vi "3.0.0_Power_Tunings & AW_Performance_Test_ECO_&_BOOST.vi"(7 "Data in":T1, 8 "error in (no error)":errorcluster, 9 "AllControls In":T2, 10 "?":T4, 11 "Message Queue out":T5) -> (0 "error out":errorcluster, 1 "Flow":string, 2 "Data":T4, 3 "Message Queue Out":T5, 5 "Data out":T1)   [LabVIEW 2017]
uses:
  Depends/AMC/subVIs/TypeDefs/amc_Message Queue.ctl
  Depends/AMC/subVIs/TypeDefs/amc_Message.ctl
  Depends/Tools/Keyed Array/Tools_KeyedArray KeyedArray.ctl
  Ctrls/Data.ctl
  DIPC 692 Daemon API/typdef/airwatt tune parameter.ctl
  Ctrls/AllControls.ctl
  Ctrls/CSV_Data.ctl
panel:
  in  "absolute position/mm 2":i32=10
  out "Array":T3[](array[typedef])
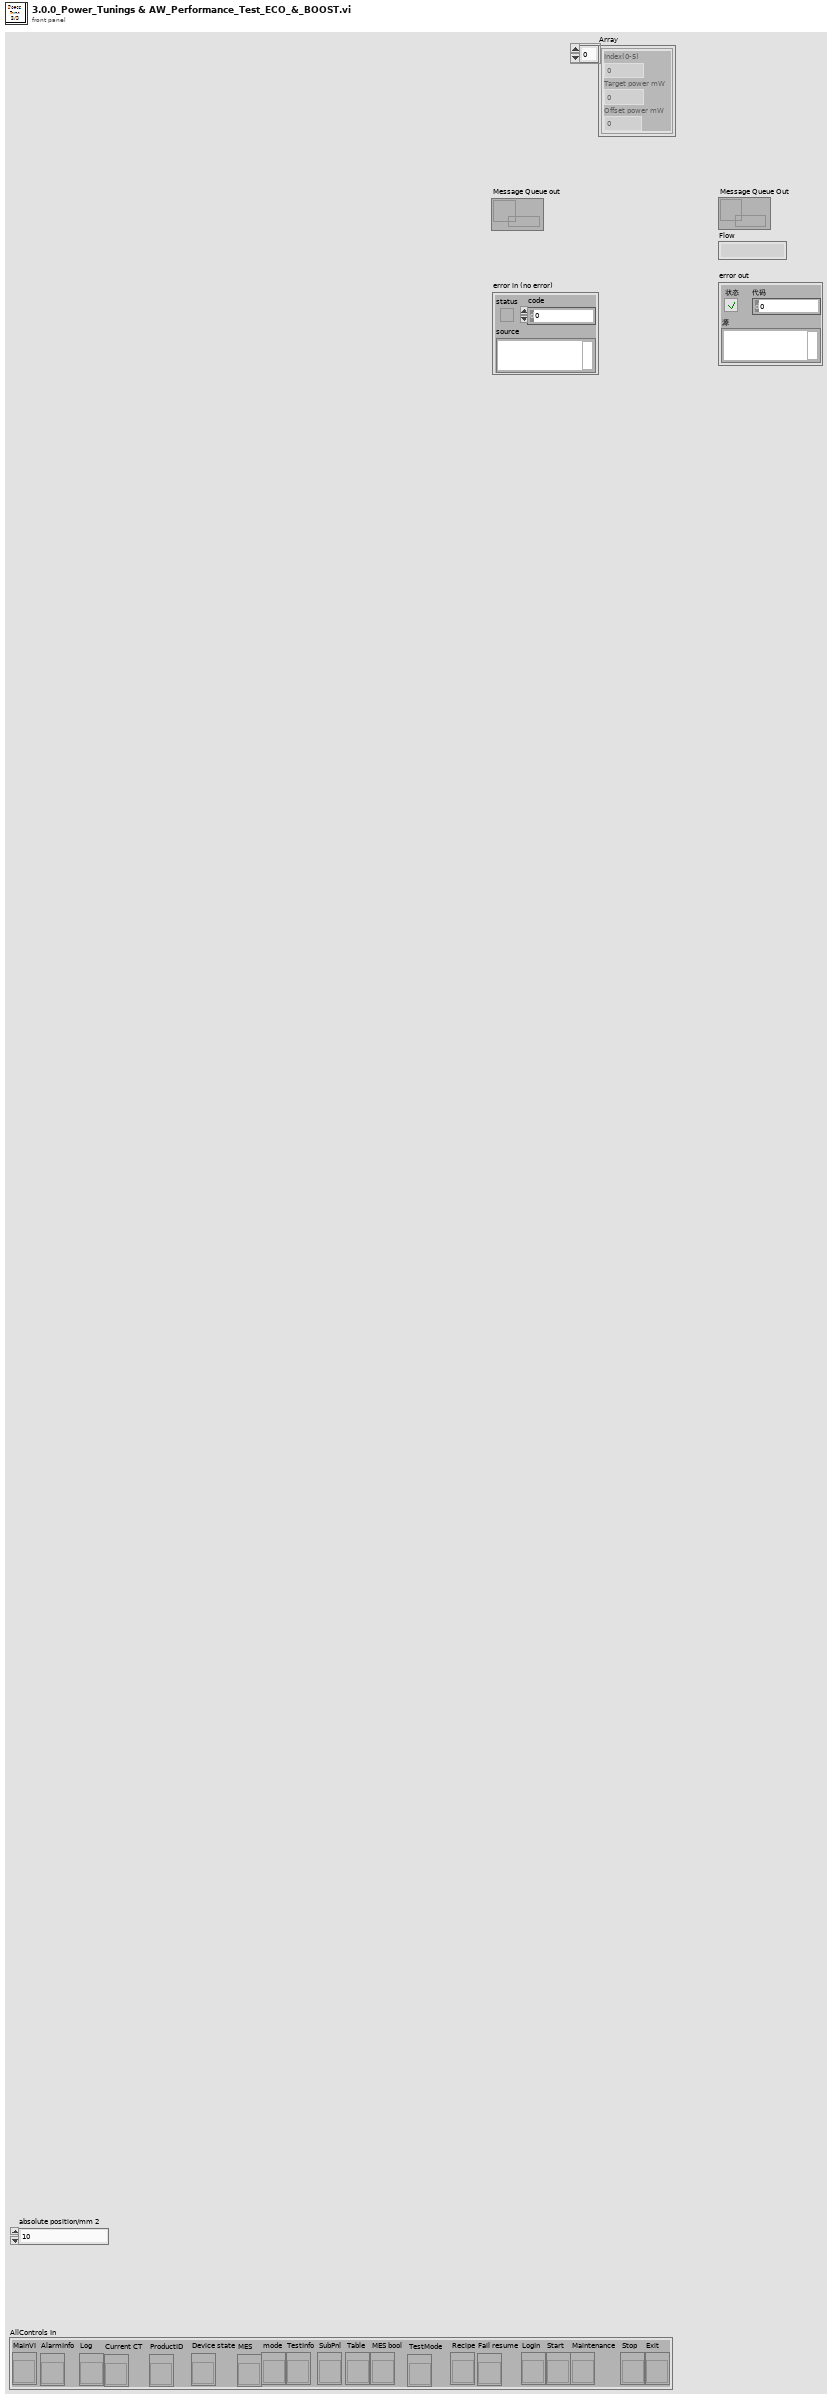
[diagram p1: front panel]
types:
  T1 = typedef "CSV_Data.ctl" = cluster{"Initialisation":cluster{"LMT - Connect UUT (con COM)":string, "LMT - Software Version (rrel)":string, "LMT - Write SKU file (wskuc)":string, "LMT - SKU file name":string, "Connect UUT DDM":string, "Read DDM EOL Timestamp - Mode":string, "Read DDM EOL Timestamp - Timestamp":string, "Read DDM EOL Timestamp - Rig ID":string, "Read DDM EOL Timestamp - Passmark ID":string, "Read DDM EOL Timestamp - Passmark Rev":string, "Software Version before flashing":string, "Read Hardware Serial":string, "UUT DDM SN":string, "Compare DDM SN with MES SN":string, "Backup PCBA Calibration EEPROM Response - CAL":string, "Flash Firmware Version":string, "Check SW Version":string, "Read DDM SW Version after flashing":string, "Set SKU Config":string, "Ready Status":string, "Set Device Mode to EOL":string, "DDM Parameter - Voltage":string, "DDM Parameter - Current":string, "DDM Parameter - Power":string, "DDM Parameter - Speed":string, "DDM Parameter - Pressure":string, "Tester Parameter - Voltage":string, "Tester Parameter - Current":string, "Tester Parameter - Power":string, "Tester Parameter - Ambient Pressure":string, "Tester Parameter - Ambient Temperature":string, "Calculated Parameter - DDM Pressure Corrected":string, "Calculated Parameter - DDM Real Power":string, "Calculated Parameter - Delta V":string}, "BEMF_Calibration":cluster{"Calibration Result - eol_cold_bemf_temp":string, "DDM Ambient Temp":string, "Restriction Plate Diameter":string, "Calibration Result - eol_bemf_mp_cold_coef_a":string, "Calibration Result - eol_bemf_mp_cold_coef_b":string, "Calibration Result - eol_bemf_mp_cold_coef_c":string, "Calibration Result - eol_bemf_lsi_cold_ref_coeffs":string, "Get - Calibration Result - eol_bemf_lsi_speed":string, "Get - Calibration Result - eol_bemf_lsi_integral_0":string, "Calibration Result - eol_bemf_lsi_integral_1":string, "Get - Calibration Result - eol_bemf_lsi_integral_2":string, "Get - Calibration Result - eol_cold_bemf":string, "Get - Calibration Result - eol_cold_bemf_fisf":string, "Finalise Calibration":string, "Compare -Calibration Result - eol_cold_bemf":string, "Compare -Calibration Result - eol_cold_bemf_fisf":string}, "ECO":cluster{"Reset Power Tune":string, "Reset BEMF FISF Calibration":string, "Restriction Plate Diameter":string, "ECO - Stabilisation Time":string, "ECO - DDM Parameter - Voltage":string, "ECO - DDM Parameter - Current":string, "ECO - DDM Parameter - Power":string, "ECO - DDM Parameter - Measured Power":string, "ECO - DDM Parameter - Speed":string, "ECO - DDM Parameter - Pressure":string, "ECO - Tester Parameter - Voltage":string, "ECO - Tester Parameter - Current":string, "ECO - Tester Parameter - Power":string, "ECO - Tester Parameter - Ambient Pressure":string, "ECO - Tester Parameter - Ambient Temperature":string, "ECO - Tester Parameter - Ambient Humidity":string, "ECO - Calculated Parameter - DDM Pressure Corrected":string, "ECO - Calculated Parameter - DDM Real Power":string, "ECO - Calculated Parameter - Delta V":string, "ECO - Calculated Parameter - Flowrate":string, "ECO - Calculated Parameter - Airwatt":string, "ECO - Formula":string, "PT ECO - Power Tune Mode Status":string}, "BOOST":cluster{"Restriction Plate Diameter":string, "BOOST - Stabilisation Time":string, "BOOST - DDM Parameter - Voltage":string, "BOOST - DDM Parameter - Current":string, "BOOST - DDM Parameter - Power":string, "BOOST - DDM Parameter - Measured Power":string, "BOOST - DDM Parameter - Speed":string, "BOOST - DDM Parameter - Pressure":string, "BOOST - Tester Parameter - Voltage":string, "BOOST - Tester Parameter - Current":string, "BOOST - Tester Parameter - Power":string, "BOOST - Tester Parameter - Ambient Pressure":string, "BOOST - Tester Parameter - Ambient Temperature":string, "BOOST - Tester Parameter - Ambient Humidity":string, "BOOST - Calculated Parameter - DDM Pressure Corrected":string, "BOOST - Calculated Parameter - DDM Real Power":string, "BOOST - Calculated Parameter - Delta V":string, "BOOST - Calculated Parameter - Flowrate":string, "BOOST - Calculated Parameter - Airwatt":string, "BOOST - Get AM Presence":string, "Air Muscle Turn Off Status":string, "BOOST - Air Muscle Calculated Parameter - Airwatt B":string, "BOOST - Air Muscle Calculate Airwatt Delta":string, "PT BOOST - Power Tune Mode Status":string, "Finalise Calibration":string, "ECO - Get AW Calibration value":string, "BOOST - Get AW Calibration value":string}, "MAX":cluster{"Restriction Plate Diameter":string, "MAX - Stabilisation Time":string, "Get Average Delta Tmag (LSIdelta_FISFdelta_LSItmag_FISFtmag_IIRtmag)":string, "Get Average Delta Tmag FISF":string, "MAX - DDM Parameter - Voltage":string, "MAX - DDM Parameter - Current":string, "MAX - DDM Parameter - Power":string, "MAX - DDM Parameter - Measured Power":string, "MAX - DDM Parameter - Speed":string, "MAX - DDM Parameter - Pressure":string, "MAX - Tester Parameter - Voltage":string, "MAX - Tester Parameter - Current":string, "MAX - Tester Parameter - Power":string, "MAX - Tester Parameter - Ambient Pressure":string, "MAX - Tester Parameter - Ambient Temperature":string, "MAX - Tester Parameter - Ambient Humidity":string, "MAX - Calculated Parameter - DDM Pressure Corrected":string, "MAX - Calculated Parameter - DDM Real Power":string, "MAX - Calculated Parameter - Delta V":string, "MAX - Calculated Parameter - Flowrate":string, "MAX - Calculated Parameter - Airwatt":string, "MAX_FISF_Check_Average_Delta_Tmag":string, "MAX - FISF - BEMF Finetune Result":string, "MAX tune - Delta P1":string, "MAX tune - Calculated Parameter - Airwatt":string, "Calculate Delta Airwatts - MAX finetune - Delta P2":string, "MAX finetune - DDM Parameter - Voltage":string, "MAX finetune - DDM Parameter - Current":string, "MAX finetune - DDM Parameter - Power":string, "MAX finetune - DDM Parameter - Measured Power":string, "MAX finetune - DDM Parameter - Speed":string, "MAX finetune - DDM Parameter - Pressure":string, "MAX finetune - Tester Parameter - Voltage":string, "MAX finetune - Tester Parameter - Current":string, "MAX finetune - Tester Parameter - Power":string, "MAX finetune - Tester Parameter - Ambient Pressure":string, "MAX finetune - Tester Parameter - Ambient Temperature":string, "MAX finetune - Tester Parameter - Ambient Humidity":string, "MAX finetune - Calculated Parameter - DDM Pressure Corrected":string, "MAX finetune - Calculated Parameter - DDM Real Power":string, "MAX finetune - Calculated Parameter - Delta V":string, "MAX finetune - Calculated Parameter - Flowrate":string, "MAX finetune - Calculated Parameter - Airwatt":string, "Check Derate Result":string, "Delta Tmag FISF":string, "Get Hot BEMF Result":string, "Calculate delta Pressure":string, "Finalise Calibration":string, "Calculate & Check Delta BEMF":string, "Delta P Airwatts Value":string}, "LL":cluster{"DDM Ambient Temp":string, "Restriction Plate Diameter":string, "LL - DDM Parameter - Voltage":string, "LL - DDM Parameter - Current":string, "LL - DDM Parameter - Power":string, "LL - DDM Parameter - Measured Power":string, "LL - DDM Parameter - Speed":string, "LL - DDM Parameter - Pressure":string, "LL - Tester Parameter - Voltage":string, "LL - Tester Parameter - Current":string, "LL - Tester Parameter - Power":string, "LL - DDM Real Power":string, "LL - Calibrate Task Detect LL":string}, "HL":cluster{"HL - DDM Parameter - Voltage":string, "HL - DDM Parameter - Current":string, "HL - DDM Parameter - Power":string, "HL - DDM Parameter - Measured Power":string, "HL - DDM Parameter - Speed":string, "HL - DDM Parameter - Pressure":string, "HL - Tester Parameter - Voltage":string, "HL - Tester Parameter - Current":string, "HL - Tester Parameter - Power":string, "HL - DDM Real Power":string, "HL - Calibrate Task Detect HL":string}, "LH":cluster{"Restriction Plate Diameter":string, "LH - DDM Parameter - Voltage":string, "LH - DDM Parameter - Current":string, "LH - DDM Parameter - Power":string, "LH - DDM Parameter - Measured Power":string, "LH - DDM Parameter - Speed":string, "LH - DDM Parameter - Pressure":string, "LH - Tester Parameter - Voltage":string, "LH - Tester Parameter - Current":string, "LH - Tester Parameter - Power":string, "LH - DDM Real Power":string, "LH - Calibrate Task Detect LH":string}, "HH":cluster{"HH - DDM Parameter - Voltage":string, "HH - DDM Parameter - Current":string, "HH - DDM Parameter - Power":string, "HH - DDM Parameter - Measured Power":string, "HH - DDM Parameter - Speed":string, "HH - DDM Parameter - Pressure":string, "HH - Tester Parameter - Voltage":string, "HH - Tester Parameter - Current":string, "HH - Tester Parameter - Power":string, "HH - DDM Real Power":string, "HH - Calibrate Task Detect HH":string}, "Inlet Blockage Calibration":cluster{"Inlet Blockage Calibration - DDM Parameter - Voltage":string, "Inlet Blockage Calibration - DDM Parameter - Current":string, "Inlet Blockage Calibration - DDM Parameter - Power":string, "Inlet Blockage Calibration - DDM Parameter - Measured Power":string, "Inlet Blockage Calibration - DDM Parameter - Speed":string, "Inlet Blockage Calibration - DDM Parameter - Pressure":string, "Inlet Blockage Calibration - Tester Parameter - Voltage":string, "Inlet Blockage Calibration - Tester Parameter - Current":string, "Inlet Blockage Calibration - Tester Parameter - Power":string, "Inlet Blockage Calibration - DDM Real Power":string, "Calibration Inlet Blockage_E":string, "Finalise Calibration":string, "Get Task Detect LL":string, "Get Task Detect HL":string, "Get Task Detect LH":string, "Get Task Detect HH":string, "Calibration Inlet Blockage":string, "Calibration eol cold bemf temp":string}, "GOOD":cluster{"GOOD UNIT - Clear EEPROM Error Log":string, "GOOD UNIT - Write Product Timestamp - Mode":string, "GOOD UNIT - Write Product Timestamp - Timestamp":string, "GOOD UNIT - Write Product Timestamp - Rig ID":string, "GOOD UNIT - Write Product Timestamp - Passmark ID":string, "GOOD UNIT - Write Product Timestamp - Passmark Rev":string, "GOOD UNIT - Set Device Mode to PROD":string, "GOOD UNIT - Backup PCBA Calibration EEPROM Response":string, "GOOD UNIT - Check Security Bit":string, "GOOD UNIT - Set Calibration Lock":string, "GOOD UNIT - Get_Calibration_Lock":string, "GOOD UNIT - Disconnect UUT":string}, "NG":cluster{"NG UNIT - Read NVM Error":string, "NG UNIT - Set Device Mode to FCT":string, "NG UNIT - Backup PCBA Calibration EEPROM Response - CAL":string, "NG UNIT - Backup PCBA Calibration EEPROM Response - ERROR":string, "NG UNIT - Backup PCBA Calibration EEPROM Response - USAGE":string, "NG UNIT - Disconnect UUT":string}, "SN":string, "Table":string[][], "Count":cluster{"Total":i32, "OK":i32, "NG":i32, "Yield":dbl}, "Start Time":timestamp, "daemon reference":refnum<k5>, "CT":dbl, "Config":string[][], "OK/NG":bool, "Station ID":string, "MES DDM SN":string, "MES PCBA SN":string, "Retest":string, "Lux":string, "Initialisation_Status":cluster{"LMT - Connect UUT (con COM)":string, "LMT - Software Version (rrel)":string, "LMT - Write SKU file (wskuc)":string, "LMT - SKU file name":string, "Connect UUT DDM":string, "Read DDM EOL Timestamp - Mode":string, "Read DDM EOL Timestamp - Timestamp":string, "Read DDM EOL Timestamp - Rig ID":string, "Read DDM EOL Timestamp - Passmark ID":string, "Read DDM EOL Timestamp - Passmark Rev":string, "Software Version before flashing":string, "Read Hardware Serial":string, "UUT DDM SN":string, "Compare DDM SN with MES SN":string, "Backup PCBA Calibration EEPROM Response - CAL":string, "Flash Firmware Version":string, "Check SW Version":string, "Read DDM SW Version after flashing":string, "Set SKU Config":string, "Ready Status":string, "Set Device Mode to EOL":string, "DDM Parameter - Voltage":string, "DDM Parameter - Current":string, "DDM Parameter - Power":string, "DDM Parameter - Speed":string, "DDM Parameter - Pressure":string, "Tester Parameter - Voltage":string, "Tester Parameter - Current":string, "Tester Parameter - Power":string, "Tester Parameter - Ambient Pressure":string, "Tester Parameter - Ambient Temperature":string, "Calculated Parameter - DDM Pressure Corrected":string, "Calculated Parameter - DDM Real Power":string, "Calculated Parameter - Delta V":string}, "BEMF_Calibration_Status":cluster{"Calibration Result - eol_cold_bemf_temp":string, "DDM Ambient Temp":string, "Restriction Plate Diameter":string, "Calibration Result - eol_bemf_mp_cold_coef_a":string, "Calibration Result - eol_bemf_mp_cold_coef_b":string, "Calibration Result - eol_bemf_mp_cold_coef_c":string, "Calibration Result - eol_bemf_lsi_cold_ref_coeffs":string, "Get - Calibration Result - eol_bemf_lsi_speed":string, "Get - Calibration Result - eol_bemf_lsi_integral_0":string, "Calibration Result - eol_bemf_lsi_integral_1":string, "Get - Calibration Result - eol_bemf_lsi_integral_2":string, "Get - Calibration Result - eol_cold_bemf":string, "Get - Calibration Result - eol_cold_bemf_fisf":string, "Finalise Calibration":string, "Compare -Calibration Result - eol_cold_bemf":string, "Compare -Calibration Result - eol_cold_bemf_fisf":string}, "ECO_Status":cluster{"Reset Power Tune":string, "Reset BEMF FISF Calibration":string, "Restriction Plate Diameter":string, "ECO - Stabilisation Time":string, "ECO - DDM Parameter - Voltage":string, "ECO - DDM Parameter - Current":string, "ECO - DDM Parameter - Power":string, "ECO - DDM Parameter - Measured Power":string, "ECO - DDM Parameter - Speed":string, "ECO - DDM Parameter - Pressure":string, "ECO - Tester Parameter - Voltage":string, "ECO - Tester Parameter - Current":string, "ECO - Tester Parameter - Power":string, "ECO - Tester Parameter - Ambient Pressure":string, "ECO - Tester Parameter - Ambient Temperature":string, "ECO - Tester Parameter - Ambient Humidity":string, "ECO - Calculated Parameter - DDM Pressure Corrected":string, "ECO - Calculated Parameter - DDM Real Power":string, "ECO - Calculated Parameter - Delta V":string, "ECO - Calculated Parameter - Flowrate":string, "ECO - Calculated Parameter - Airwatt":string, "ECO - Formula":string, "PT ECO - Power Tune Mode Status":string}, "BOOST_Status":cluster{"Restriction Plate Diameter":string, "BOOST - Stabilisation Time":string, "BOOST - DDM Parameter - Voltage":string, "BOOST - DDM Parameter - Current":string, "BOOST - DDM Parameter - Power":string, "BOOST - DDM Parameter - Measured Power":string, "BOOST - DDM Parameter - Speed":string, "BOOST - DDM Parameter - Pressure":string, "BOOST - Tester Parameter - Voltage":string, "BOOST - Tester Parameter - Current":string, "BOOST - Tester Parameter - Power":string, "BOOST - Tester Parameter - Ambient Pressure":string, "BOOST - Tester Parameter - Ambient Temperature":string, "BOOST - Tester Parameter - Ambient Humidity":string, "BOOST - Calculated Parameter - DDM Pressure Corrected":string, "BOOST - Calculated Parameter - DDM Real Power":string, "BOOST - Calculated Parameter - Delta V":string, "BOOST - Calculated Parameter - Flowrate":string, "BOOST - Calculated Parameter - Airwatt":string, "BOOST - Get AM Presence":string, "Air Muscle Turn Off Status":string, "BOOST - Air Muscle Calculated Parameter - Airwatt B":string, "BOOST - Air Muscle Calculate Airwatt Delta":string, "PT BOOST - Power Tune Mode Status":string, "Finalise Calibration":string, "ECO - Get AW Calibration value":string, "BOOST - Get AW Calibration value":string}, "MAX_Status":cluster{"Restriction Plate Diameter":string, "MAX - Stabilisation Time":string, "Get Average Delta Tmag (LSIdelta_FISFdelta_LSItmag_FISFtmag_IIRtmag)":string, "Get Average Delta Tmag FISF":string, "MAX - DDM Parameter - Voltage":string, "MAX - DDM Parameter - Current":string, "MAX - DDM Parameter - Power":string, "MAX - DDM Parameter - Measured Power":string, "MAX - DDM Parameter - Speed":string, "MAX - DDM Parameter - Pressure":string, "MAX - Tester Parameter - Voltage":string, "MAX - Tester Parameter - Current":string, "MAX - Tester Parameter - Power":string, "MAX - Tester Parameter - Ambient Pressure":string, "MAX - Tester Parameter - Ambient Temperature":string, "MAX - Tester Parameter - Ambient Humidity":string, "MAX - Calculated Parameter - DDM Pressure Corrected":string, "MAX - Calculated Parameter - DDM Real Power":string, "MAX - Calculated Parameter - Delta V":string, "MAX - Calculated Parameter - Flowrate":string, "MAX - Calculated Parameter - Airwatt":string, "MAX_FISF_Check_Average_Delta_Tmag":string, "MAX - FISF - BEMF Finetune Result":string, "MAX tune - Delta P1":string, "MAX tune - Calculated Parameter - Airwatt":string, "Calculate Delta Airwatts - MAX finetune - Delta P2":string, "MAX finetune - DDM Parameter - Voltage":string, "MAX finetune - DDM Parameter - Current":string, "MAX finetune - DDM Parameter - Power":string, "MAX finetune - DDM Parameter - Measured Power":string, "MAX finetune - DDM Parameter - Speed":string, "MAX finetune - DDM Parameter - Pressure":string, "MAX finetune - Tester Parameter - Voltage":string, "MAX finetune - Tester Parameter - Current":string, "MAX finetune - Tester Parameter - Power":string, "MAX finetune - Tester Parameter - Ambient Pressure":string, "MAX finetune - Tester Parameter - Ambient Temperature":string, "MAX finetune - Tester Parameter - Ambient Humidity":string, "MAX finetune - Calculated Parameter - DDM Pressure Corrected":string, "MAX finetune - Calculated Parameter - DDM Real Power":string, "MAX finetune - Calculated Parameter - Delta V":string, "MAX finetune - Calculated Parameter - Flowrate":string, "MAX finetune - Calculated Parameter - Airwatt":string, "Check Derate Result":string, "Delta Tmag FISF":string, "Get Hot BEMF Result":string, "Calculate delta Pressure":string, "Finalise Calibration":string, "Calculate & Check Delta BEMF":string, "Delta P Airwatts Value":string}, "LL_Status":cluster{"DDM Ambient Temp":string, "Restriction Plate Diameter":string, "LL - DDM Parameter - Voltage":string, "LL - DDM Parameter - Current":string, "LL - DDM Parameter - Power":string, "LL - DDM Parameter - Measured Power":string, "LL - DDM Parameter - Speed":string, "LL - DDM Parameter - Pressure":string, "LL - Tester Parameter - Voltage":string, "LL - Tester Parameter - Current":string, "LL - Tester Parameter - Power":string, "LL - DDM Real Power":string, "LL - Calibrate Task Detect LL":string}, "HL_Status":cluster{"HL - DDM Parameter - Voltage":string, "HL - DDM Parameter - Current":string, "HL - DDM Parameter - Power":string, "HL - DDM Parameter - Measured Power":string, "HL - DDM Parameter - Speed":string, "HL - DDM Parameter - Pressure":string, "HL - Tester Parameter - Voltage":string, "HL - Tester Parameter - Current":string, "HL - Tester Parameter - Power":string, "HL - DDM Real Power":string, "HL - Calibrate Task Detect HL":string}, "LH_Status":cluster{"Restriction Plate Diameter":string, "LH - DDM Parameter - Voltage":string, "LH - DDM Parameter - Current":string, "LH - DDM Parameter - Power":string, "LH - DDM Parameter - Measured Power":string, "LH - DDM Parameter - Speed":string, "LH - DDM Parameter - Pressure":string, "LH - Tester Parameter - Voltage":string, "LH - Tester Parameter - Current":string, "LH - Tester Parameter - Power":string, "LH - DDM Real Power":string, "LH - Calibrate Task Detect LH":string}, "HH_Status":cluster{"HH - DDM Parameter - Voltage":string, "HH - DDM Parameter - Current":string, "HH - DDM Parameter - Power":string, "HH - DDM Parameter - Measured Power":string, "HH - DDM Parameter - Speed":string, "HH - DDM Parameter - Pressure":string, "HH - Tester Parameter - Voltage":string, "HH - Tester Parameter - Current":string, "HH - Tester Parameter - Power":string, "HH - DDM Real Power":string, "HH - Calibrate Task Detect HH":string}, "Inlet Blockage Calibration_Status":cluster{"Inlet Blockage Calibration - DDM Parameter - Voltage":string, "Inlet Blockage Calibration - DDM Parameter - Current":string, "Inlet Blockage Calibration - DDM Parameter - Power":string, "Inlet Blockage Calibration - DDM Parameter - Measured Power":string, "Inlet Blockage Calibration - DDM Parameter - Speed":string, "Inlet Blockage Calibration - DDM Parameter - Pressure":string, "Inlet Blockage Calibration - Tester Parameter - Voltage":string, "Inlet Blockage Calibration - Tester Parameter - Current":string, "Inlet Blockage Calibration - Tester Parameter - Power":string, "Inlet Blockage Calibration - DDM Real Power":string, "Calibration Inlet Blockage_E":string, "Finalise Calibration":string, "Get Task Detect LL":string, "Get Task Detect HL":string, "Get Task Detect LH":string, "Get Task Detect HH":string, "Calibration Inlet Blockage":string, "Calibration eol cold bemf temp":string}, "GOOD_Status":cluster{"GOOD UNIT - Clear EEPROM Error Log":string, "GOOD UNIT - Write Product Timestamp - Mode":string, "GOOD UNIT - Write Product Timestamp - Timestamp":string, "GOOD UNIT - Write Product Timestamp - Rig ID":string, "GOOD UNIT - Write Product Timestamp - Passmark ID":string, "GOOD UNIT - Write Product Timestamp - Passmark Rev":string, "GOOD UNIT - Set Device Mode to PROD":string, "GOOD UNIT - Backup PCBA Calibration EEPROM Response":string, "GOOD UNIT - Check Security Bit":string, "GOOD UNIT - Set Calibration Lock":string, "GOOD UNIT - Get_Calibration_Lock":string, "GOOD UNIT - Disconnect UUT":string}, "NG_Status":cluster{"NG UNIT - Read NVM Error":string, "NG UNIT - Set Device Mode to FCT":string, "NG UNIT - Backup PCBA Calibration EEPROM Response - CAL":string, "NG UNIT - Backup PCBA Calibration EEPROM Response - ERROR":string, "NG UNIT - Backup PCBA Calibration EEPROM Response - USAGE":string, "NG UNIT - Disconnect UUT":string}, "SKU":string, "Plate_Diameter":string, "Alarm":string}
  T2 = typedef "AllControls.ctl" = cluster{"MainVI":refnum<vi>, "AlarmInfo":refnum<vi>, "Log":refnum<vi>, "Current CT":refnum<vi>, "ProductID":refnum<vi>, "Device state":refnum<vi>, "MES":refnum<vi>, "mode":refnum<vi>, "TestInfo":refnum<vi>, "SubPnl":refnum<vi>, "Table":refnum<vi>, "MES bool":refnum<vi>, "TestMode":refnum<vi>, "Recipe":refnum<vi>, "Fail resume":refnum<vi>, "LogIn":refnum<vi>, "Start":refnum<vi>, "Maintenance":refnum<vi>, "Stop":refnum<vi>, "Exit":refnum<vi>}
  T3 = typedef "airwatt tune parameter.ctl" = cluster{"Index(0-5)":i64, "Target power mW":i64, "Offset power mW":i64}
  T4 = typedef "Data.ctl" = cluster{"Initialisation":cluster{"DDM_Parameter":dbl[], "DDM_Parameter_status":bool[], "Get_Tester_Parameter":dbl[], "Get_Tester_Parameter_status":bool[], "Cal_Tester_Parameter":dbl[], "Cal_Tester_Parameter_status":bool[], "sw_version_before_status":bool, "sw_version_after_status":bool, "Set_SKU_Config_With_LMT_status":bool, "FCT_timestamp_status":bool, "LMT_Connect_to_UUT_status":bool}, "BEMF_Calibration":cluster{"Read_ambient_temperature":dbl, "Calibration_Vaule":dbl[], "Calibration_Vaule _B":dbl[], "Calibration_Vaule_status":bool[], "Calibration_Vaule_B_status":bool[]}, "ECO":cluster{"DDM_Parameter":dbl[], "DDM_Parameter_status":bool[], "Get_Tester_Parameter":dbl[], "Get_Tester_Parameter_status":bool[], "Cal_Tester_Parameter":dbl[], "Cal_Tester_Parameter_status":bool[], "DDM_Parameter_after_power_tune":dbl[], "Get_Tester_Parameter_after_power_tune":dbl[], "Cal_Tester_Parameter_after_power_tune":dbl[], "Cal_Tester_Parameter_after_power_tune_status":bool[], "Delta_P":dbl}, "BOOST":cluster{"DDM_Parameter":dbl[], "DDM_Parameter_status":bool[], "Get_Tester_Parameter":dbl[], "Get_Tester_Parameter_status":bool[], "Cal_Tester_Parameter":dbl[], "Cal_Tester_Parameter_status":bool[], "DDM_Parameter_after_power_tune":dbl[], "Get_Tester_Parameter_after_power_tune":dbl[], "Cal_Tester_Parameter_after_power_tune":dbl[], "Cal_Tester_Parameter_after_power_tune_status":bool[], "airwatts_am_off":dbl, "AW_Delta_(AM_on_and_off)":dbl, "AW_Delta_(AM_on_and_off)_Status":bool, "Delta_P":dbl}, "MAX":cluster{"Average_Tmag_Data":cluster{"LSI Delta in degC":dbl, "FISF Delta in degc":dbl, "LSI Tmag in degC":dbl, "Fisf Tmag in degC":dbl, "IIR Tmag in degC":dbl}, "DDM_Parameter":dbl[], "DDM_Parameter_status":bool[], "Get_Tester_Parameter":dbl[], "Get_Tester_Parameter_status":bool[], "Cal_Tester_Parameter":dbl[], "BEMF_Finetune":cluster{"eol_bemf_mp_cold_coef_c":dbl, "eol_cold_bemf_fisf_offset":dbl}, "AW_Tune":cluster{"delta_P1":dbl, "delta_P_Setting":dbl}, "DDM_Parameter_after_Airwatts_Tune":dbl[], "Get_Tester_Parameter_after_Airwatts_Tune":dbl[], "Cal_Tester_Parameter_after_Airwatts_Tune":dbl[], "DDM_Parameter_after_Airwatts_Finetune":dbl[], "Get_Tester_Parameter_after_Airwatts_Finetune":dbl[], "Cal_Tester_Parameter_after_Airwatts_Finetune":dbl[], "AW_Finetune":cluster{"delta_P2":dbl, "delta_P_Setting":dbl}, "Delta_Tmag_after_tune":cluster{"LSI Delta in degC":dbl, "FISF Delta in degc":dbl, "LSI Tmag in degC":dbl, "Fisf Tmag in degC":dbl, "IIR Tmag in degC":dbl}, "Hot Bemf in mV":dbl, "DDM_Pressure":dbl, "Delta_Pressure":dbl, " Cold Bemf in mV":dbl, " delta Bemf":dbl, " delta p":dbl, "Delta_Pressure_status":bool, " delta Bemf_status":bool, "LSI Delta in degC_status":bool, "FISF Delta in degc_status":bool, "Max_check_derate_status_status":bool, "Average_All_data":dbl[][], "Average_Tmag_Data_status":bool[], "Average_Tmag_Data_after_tune_status":bool[], "Cal_Tester_Parameter_status":bool[], "Cal_Tester_Parameter_status_after_Airwatts_Tune":bool[], "Cal_Tester_Parameter_status_after_Airwatts_FineTune":bool[]}, "Task_Detect_Calib":cluster{"LL":cluster{"DDM_Parameter":dbl[], "DDM_Parameter_status":bool[], "Get_Tester_Parameter":dbl[], "Get_Tester_Parameter_status":bool[], "Set_task_detect_A":dbl, "Set_task_detect_A_Status":bool}, "HL":cluster{"DDM_Parameter":dbl[], "DDM_Parameter_status":bool[], "Get_Tester_Parameter":dbl[], "Get_Tester_Parameter_status":bool[], "Set_task_detect_B":dbl, "Set_task_detect_B_Status":bool}, "LH":cluster{"DDM_Parameter":dbl[], "DDM_Parameter_status":bool[], "Get_Tester_Parameter":dbl[], "Get_Tester_Parameter_status":bool[], "Set_task_detect_C":dbl, "Set_task_detect_C_Status":bool}, "HH":cluster{"DDM_Parameter":dbl[], "DDM_Parameter_status":bool[], "Get_Tester_Parameter":dbl[], "Get_Tester_Parameter_status":bool[], "Set_task_detect_D":dbl, "Read_and_check_calibration_Status":bool[], "Set_task_detect_D_Status":bool}, "Get_eol_inlet_blockage_E":dbl, "Calib_vaule":cluster{"Get_task_detect_LL":dbl, "Get_task_detect_HL":dbl, "Get_task_detect_LH":dbl, "Get_task_detect_HH":dbl, "eol_inlet_blockage":dbl, "eol_code_bemf_temp":dbl}, "calibrated temp":dbl, "Inlet_Blockage_Calibration":cluster{"DDM_Parameter":dbl[], "DDM_Parameter_status":bool[], "Get_Tester_Parameter":dbl[], "Get_Tester_Parameter_status":bool[]}, "Get_eol_inlet_blockage_E_Status":bool}, "good":cluster{"Write_Product_TS":cluster{"TIMESTAMP":i64, "RIG_ID":i64, "PASSMARK_ID":i64, "PASSMARK_REV":i64}, "Read_Product_TS":cluster{"TIMESTAMP":i64, "RIG_ID":i64, "PASSMARK_ID":i64, "PASSMARK_REV":i64}, "Good_Check_Secuity_Bit_Stauts":bool}}
  T5 = typedef "amc_Message Queue.ctl" = refnum<queue>
  T6 = cluster{"getVersion":string, "Start Test mode":string, "Start camera test mode P1":string, "get one RAW Image":string, "Start camera test mode P0":string, "Stop Test Mode":string, "Stop Camera":string}
  T7 = typedef "HD Config.ctl" = cluster{" PC":cluster{"PC Address":u8[], "PC Port":i32}, "FCO":cluster{"COM":refnum<visa-resource-name>, "Baudrate":u32}, "DC Power ":cluster{"COM":refnum<visa-resource-name>, "Baudrate":u32}, "PW3336":cluster{"COM":refnum<visa-resource-name>, "Baudrate":u32}, "Lefoo":cluster{"COM":refnum<visa-resource-name>, "Baudrate":u32}, "Tempt&Hum":cluster{"COM":refnum<visa-resource-name>, "Baudrate":u32}, "DIPC":cluster{"COM":refnum<visa-resource-name>}, "Daemon":cluster{"IP Address":string, "Port":u16, "Retry":u16}, "Motor":cluster{"COM":refnum<visa-resource-name>, "Baudrate":u32}, "Fail_resume_mode":bool, "GRR":bool}
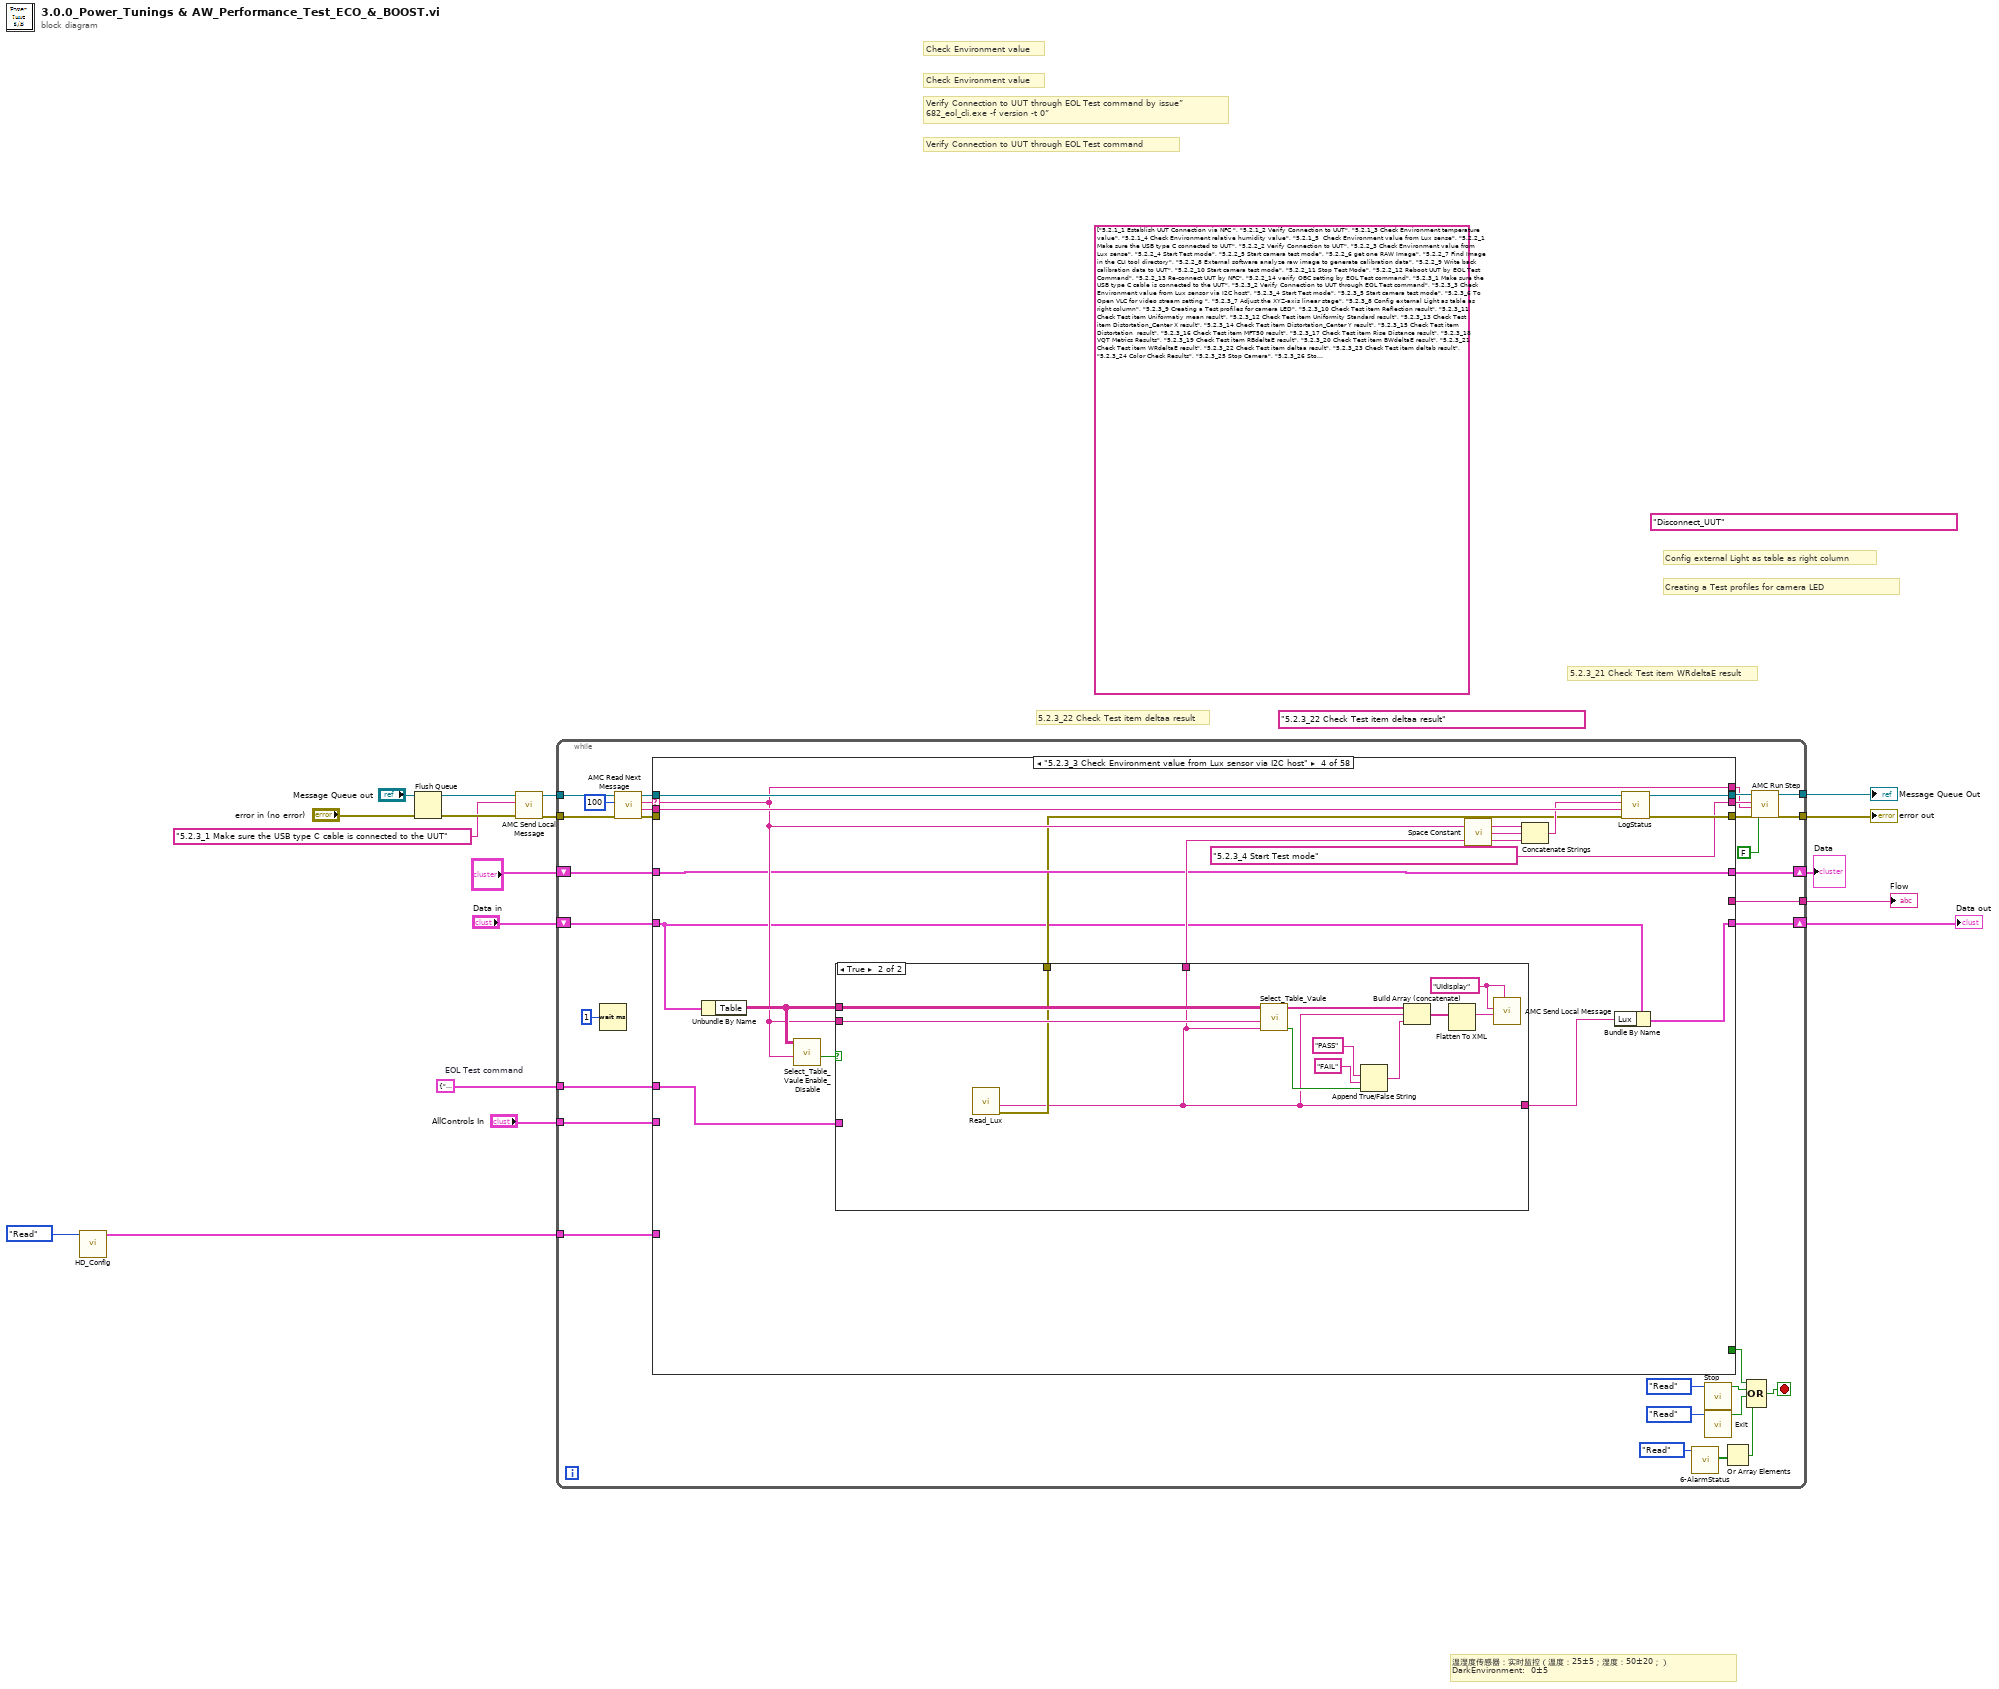
[diagram p0: block diagram]
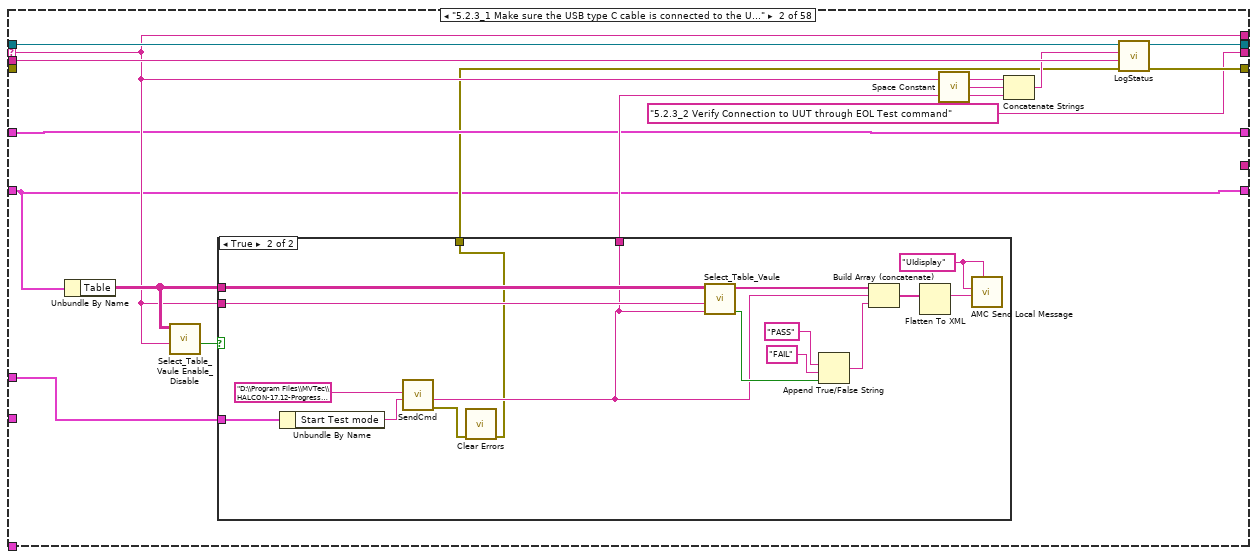
[diagram p3: hidden frame]
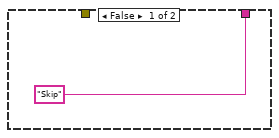
[diagram p4: hidden frame]
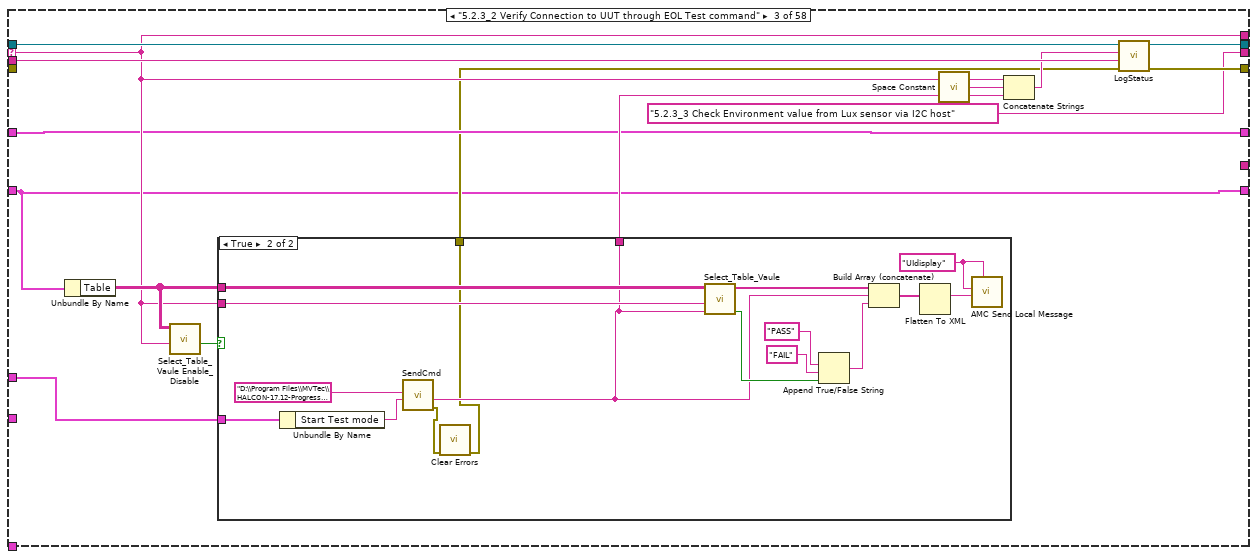
[diagram p5: hidden frame]
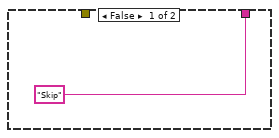
[diagram p6: hidden frame]
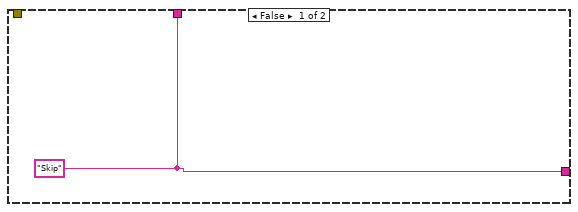
[diagram p7: hidden frame]
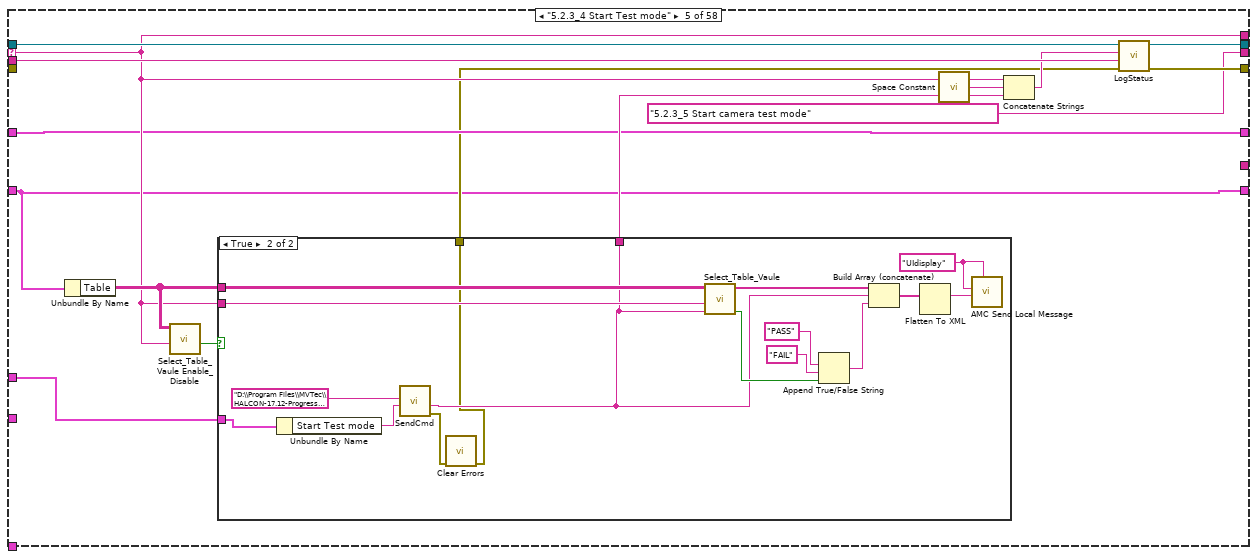
[diagram p8: hidden frame]
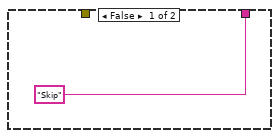
[diagram p9: hidden frame]
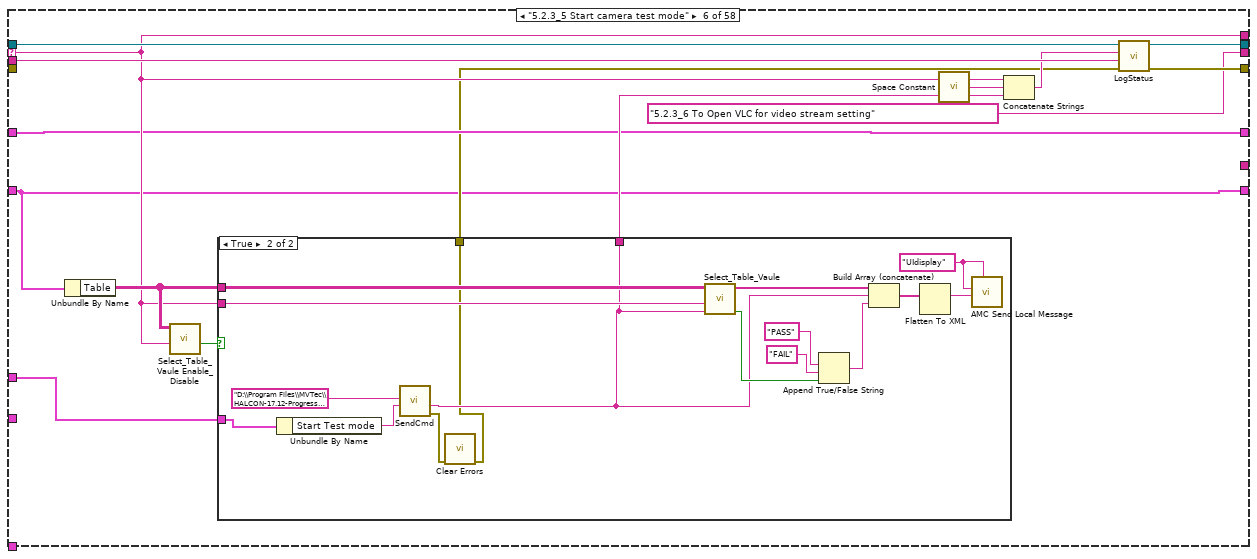
[diagram p10: hidden frame]
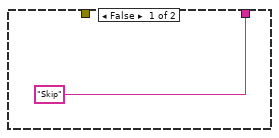
[diagram p11: hidden frame]
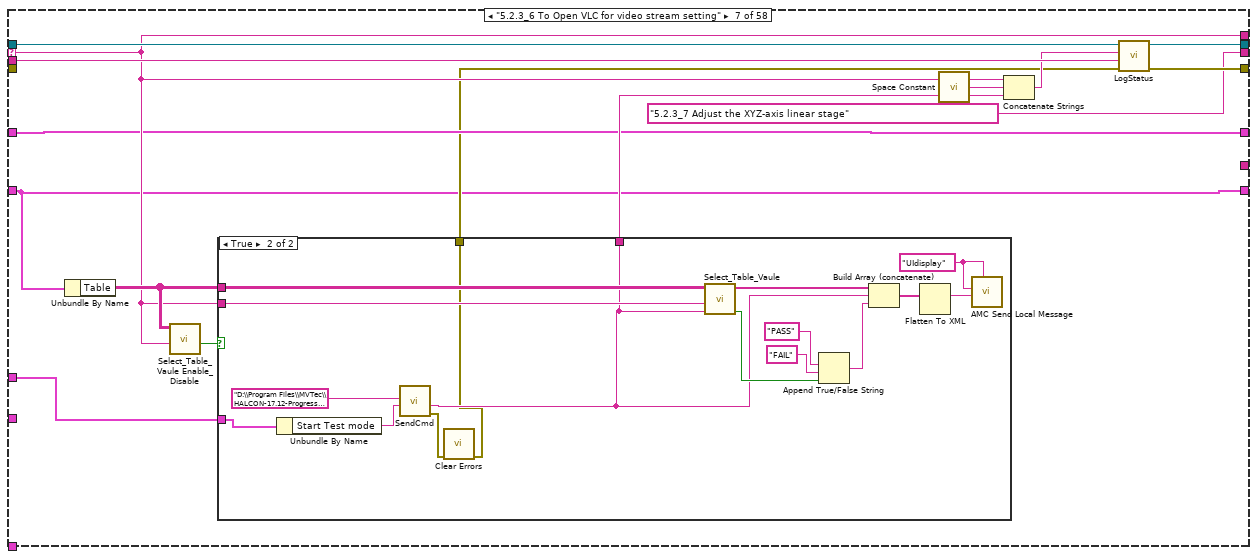
[diagram p12: hidden frame]
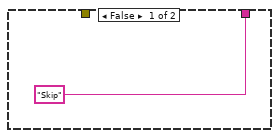
[diagram p13: hidden frame]
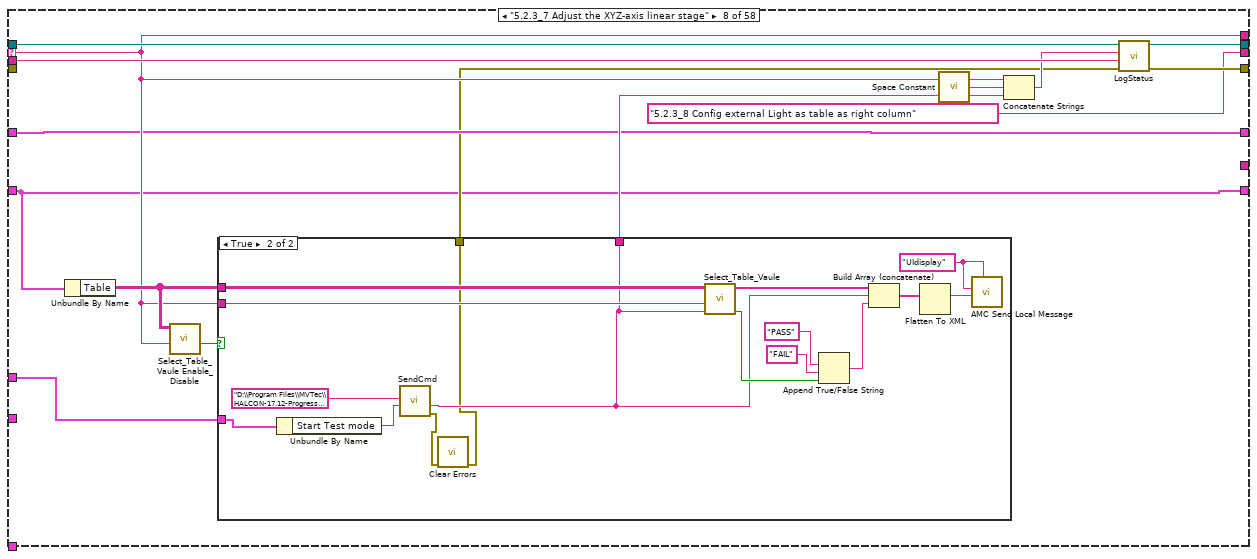
[diagram p14: hidden frame]
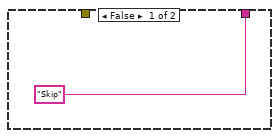
[diagram p15: hidden frame]
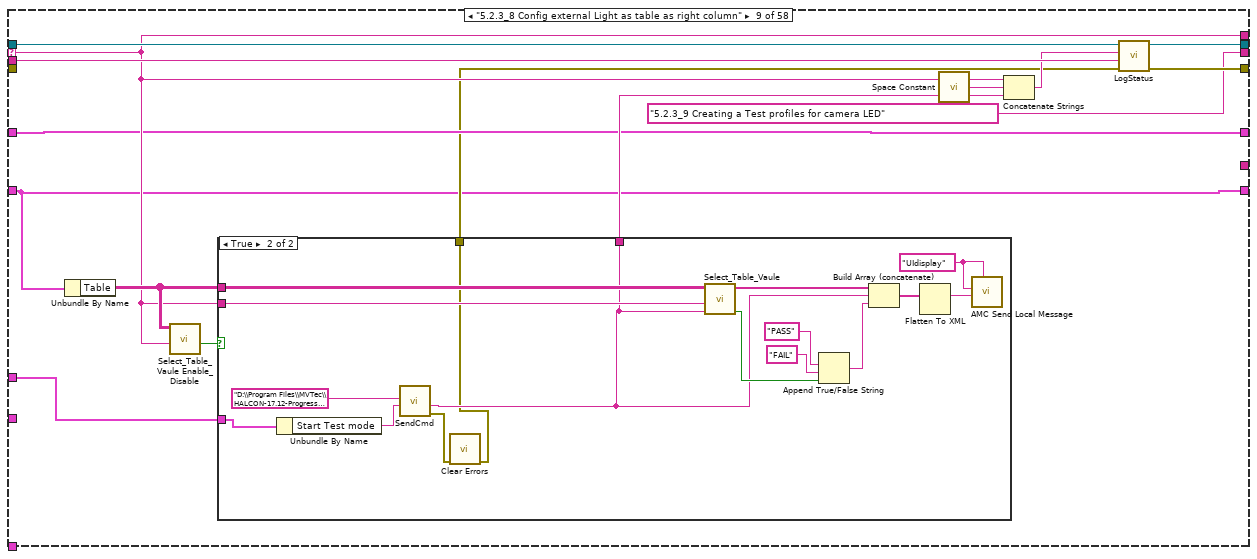
[diagram p16: hidden frame]
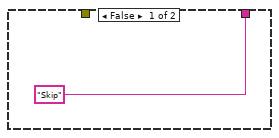
[diagram p17: hidden frame]
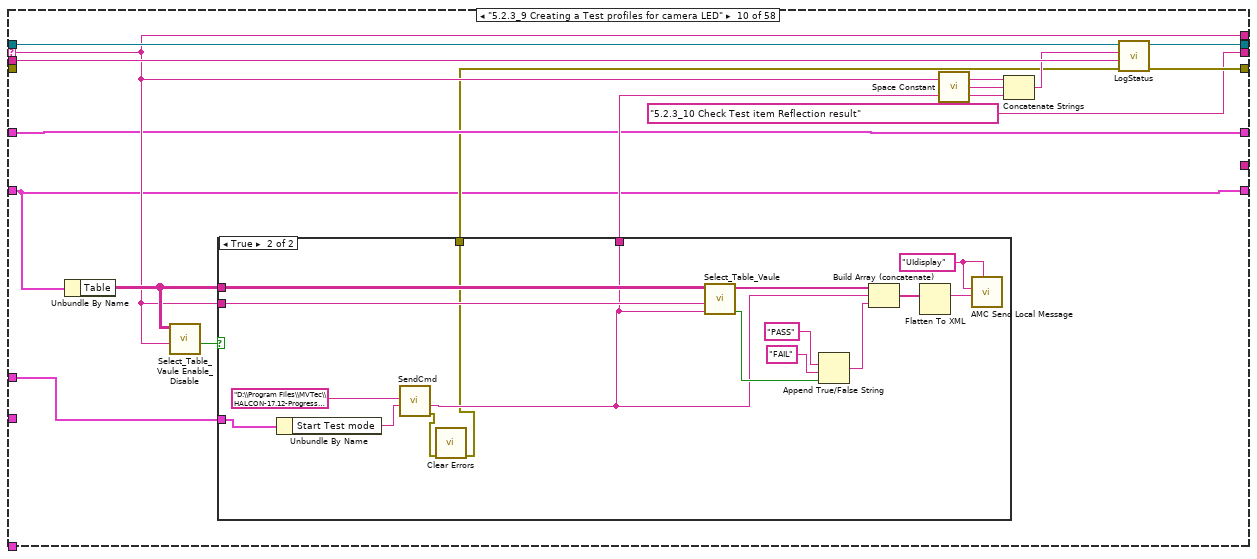
[diagram p18: hidden frame]
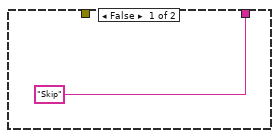
[diagram p19: hidden frame]
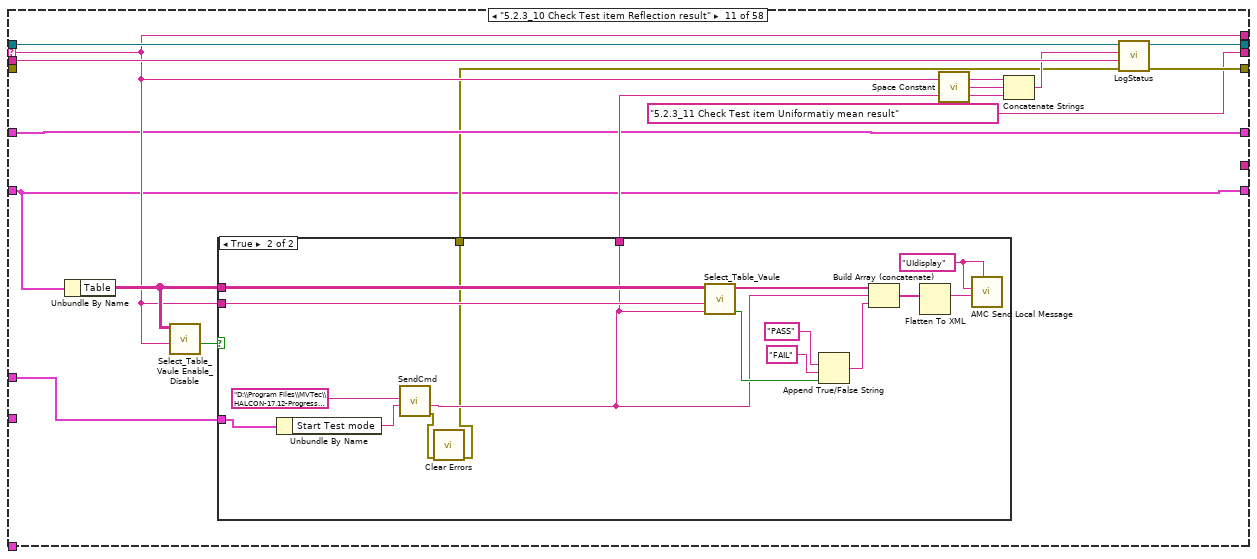
[diagram p20: hidden frame]
diagram:
  (unwired) "5.2.3_22 Check Test item deltaa result"
  (unwired) "Disconnect_UUT"
  (unwired) string[] ["5.2.1_1 Establish UUT Connection via NFC ", "5.2.1_2 Verify Connection to UUT", "5.2.1_3 Check Environment temperature value", "5.2.1_4 Check Environment relative humidity value", "5.2.1_5  Check Environment value from Lux sense", "5.2.2_1 Make sure the USB type C connected to UUT", "5.2.2_2 Verify Connection to UUT", "5.2.2_3 Check Environment value from Lux sense", "5.2.2_4 Start Test mode", "5.2.2_5 Start camera test mode", "5.2.2_6 get one RAW Image", "5.2.2_7 Find Image  in the CLI tool directory", "5.2.2_8 External software analyze raw image to generate calibration data", "5.2.2_9 Write back calibration data to UUT", "5.2.2_10 Start camera test mode", "5.2.2_11 Stop Test Mode", "5.2.2_12 Reboot UUT by EOL Test Command", "5.2.2_13 Re-connect UUT by NFC", "5.2.2_14 verify OBC setting by EOL Test command", "5.2.3_1 Make sure the USB type C cable is connected to the UUT", "5.2.3_2 Verify Connection to UUT through EOL Test command", "5.2.3_3 Check Environment value from Lux sensor via I2C host", "5.2.3_4 Start Test mode", "5.2.3_5 Start camera test mode", "5.2.3_6 To Open VLC for video stream setting ", "5.2.3_7 Adjust the XYZ-axis linear stage", "5.2.3_8 Config external Light as table as right column", "5.2.3_9 Creating a Test profiles for camera LED", "5.2.3_10 Check Test item Reflection result", "5.2.3_11 Check Test item Uniformatiy mean result", "5.2.3_12 Check Test item Uniformity Standard result", "5.2.3_13 Check Test item Distortation_Center X result", "5.2.3_14 Check Test item Distortation_Center Y result", "5.2.3_15 Check Test item Distortation  result", "5.2.3_16 Check Test item MFT50 result", "5.2.3_17 Check Test item Rise Distance result", "5.2.3_18 VQT Metrics Results", "5.2.3_19 Check Test item RBdeltaE result", "5.2.3_20 Check Test item BWdeltaE result", "5.2.3_21 Check Test item WRdeltaE result", "5.2.3_22 Check Test item deltaa result", "5.2.3_23 Check Test item deltab result", "5.2.3_24 Color Check Results", "5.2.3_25 Stop Camera", "5.2.3_26 Stop Test mode", "5.2.3_27 Shutdown UUT"] ("subarray")
  w1 = T6 {"getVersion"="682_eol_cli.exe -f version -t 0", "Start Test mode"="682_eol_cli.exe -f test -p 1", "Start camera test mode P1"="682_eol_cli.exe -f camera -p 1", "get one RAW Image"="“682_eol_cli.exe -f camera -p 2", "Start camera test mode P0"="682_eol_cli.exe -f camera -p 0", "Stop Test Mode"="682_eol_cli.exe -f test -p 0", "Stop Camera"="682_eol_cli.exe -f camera -p 0"}  # EOL Test command
  # "5.2.3_21 Check Test item WRdeltaE result"
  # "5.2.3_22 Check Test item deltaa result"
  # "Creating a Test profiles for camera LED"
  # "Config external Light as table as right column"
  # "温湿度传感器：实时监控（温度：25±5；湿度：50±20；）\nDarkEnvironment:  0±5"
  # "Check Environment value"
  # "Check Environment value"
  # "Verify Connection to UUT through EOL Test command by issue” \n682_eol_cli.exe -f version -t 0”"
  # "Verify Connection to UUT through EOL Test command"
  n1 = call "HD_Config.vi"("Step"=enum16{"Initial", "Write", "Read"}."Read") -> ("HD Config out"=w3:T7)  [unwired: 9 in, 1 out]
  n2 = Flush Queue(queue="Message Queue out") -> (queue out=w9:T5)  [unwired: 1 in, 2 out]
  n3 = call "AMC Send Local Message.vi"("error in (no error)"="error in (no error)", "Message Name"="5.2.3_1 Make sure the USB type C cable is connected to the UUT", "Message Queue in"=w9) -> ("error out"=w15:errorcluster, "Message Queue out"=w16:T5)  [unwired: 7 in]
  n4 = while {
    tunnel: w16 -> [w49]
    tunnel: [w45] -> w8
    tunnel: w15 -> [w43]
    tunnel: [w40] -> w7
    shift-right: [w36] -> w12
    shift-left: "?" -> [w37]
    tunnel: w3 -> [w35]
    tunnel: [w31] -> w10
    shift-right: [w23] -> w5
    shift-left: "Data in" -> [w22]
    tunnel: "AllControls In" -> [w24]
    tunnel: w1 -> [w18]
    stop <- w25 stop-if-true
    n5 = Wait (ms)(milliseconds to wait=u32 1 ("等待时间（毫秒）")) -> ()  [unwired: 1 out]
    n6 = call "AMC Read Next Message.vi"("error in (no error)"=w43, "timeout (1ms)"=100, "Message Queue in"=w49) -> ("error out"=w42:errorcluster, "Message Value"=w33:string, "Message Name"=w47:string, "Message Queue out"=w48:T5)  [unwired: 1 in, 4 out]
    n7 = case shown="\"5.2.3_3 Check Environment value from Lux sensor via I2C host\"" w47 {
      selector: w47 -> [_ w60 w91 w124 w151 w182 w213 w244 w275 w306 w337 w368 w399 w430 w461 w492 w523 w554 w585 w616 w647 w678 w709 w740 w771 w802 w833 w865 w896 w955 w995 w1035 w1073 w1122 w1159 w1196 w1233 w1270 w1307 w1344 w1381 w1418 w1455 w1492 w1529 w1566 w1603 w1640 w1677 w1714 w1751 w1791 w1831 w1872 w1904 w1943 w1991 w2058]
      tunnel: w48 -> [w53 w67 w98 w131 w158 w189 w220 w251 w282 w313 w344 w375 w406 w437 w468 w499 w530 w561 w592 w623 w654 w685 w716 w747 w778 w809 w840 w872 w904 w963 w1003 w1043 w1081 w1130 w1167 w1204 w1241 w1278 w1315 w1352 w1389 w1426 w1463 w1500 w1537 w1574 w1611 w1648 w1685 w1722 w1759 w1799 w1839 w1887 w1918 w1949 w1998 w2063]
      tunnel: [w53 w67 w98 w131 w158 w189 w220 w251 w282 w313 w344 w375 w406 w437 w468 w499 w530 w561 w592 w623 w654 w685 w716 w747 w778 w809 w840 w872 w904 w963 w1003 w1043 w1081 w1130 w1167 w1204 w1241 w1278 w1315 w1352 w1389 w1426 w1463 w1500 w1537 w1574 w1611 w1648 w1685 w1722 w1759 w1799 w1839 w1886 w1898 w1949 w1998 w2063] -> w46
      tunnel: w42 -> [w52 _ _ _ _ _ _ _ _ _ _ _ _ _ _ _ _ _ _ _ _ _ _ _ _ _ _ _ _ _ _ _ _ _ _ _ _ _ _ _ _ _ _ _ _ _ _ _ _ _ _ _ _ w1891 w1922 _ _ _]
      tunnel: [w52 w66 w97 w130 w157 w188 w219 w250 w281 w312 w343 w374 w405 w436 w467 w498 w529 w560 w591 w622 w653 w684 w715 w746 w777 w808 w839 w871 w903 w962 w1002 w1042 w1080 w1129 w1166 w1203 w1240 w1277 w1314 w1351 w1388 w1425 w1462 w1499 w1536 w1573 w1610 w1647 w1684 w1721 w1758 w1798 w1838 w1888 w1919 w1948 w1997 w2062] -> w41
      tunnel: [_ _ _ _ _ _ _ _ _ _ _ _ _ _ _ _ _ _ _ _ _ _ _ _ _ _ _ TRUE w893 w952 w992 w1032 w1070 w1119 w1156 w1193 w1230 w1267 w1304 w1341 w1378 w1415 w1452 w1489 w1526 w1563 w1600 w1637 w1674 w1711 w1748 w1788 w1828 w1868 w1899 w1939 w1986 TRUE] -> w26
      tunnel: w37 -> [w51 w58 w89 w122 w149 w180 w211 w242 w273 w304 w335 w366 w397 w428 w459 w490 w521 w552 w583 w614 w645 w676 w707 w738 w769 w800 w831 w863 w892 w951 w991 w1031 w1069 w1118 w1155 w1192 w1229 w1266 w1303 w1340 w1377 w1414 w1451 w1488 w1525 w1562 w1599 w1636 w1673 w1710 w1747 w1787 w1827 w1873 w1905 w1937 w1984 w2049]
      tunnel: [w51 w58 w89 w122 w149 w180 w211 w242 w273 w304 w335 w366 w397 w428 w459 w490 w521 w552 w583 w614 w645 w676 w707 w738 w769 w800 w831 w863 w892 w951 w991 w1031 w1069 w1118 w1155 w1192 w1229 w1266 w1303 w1340 w1377 w1414 w1451 w1488 w1525 w1562 w1599 w1636 w1673 w1710 w1747 w1787 w1827 w1885 w1916 w1937 w1984 w2049] -> w36
      tunnel: w33 -> [_ w65 w96 w129 w156 w187 w218 w249 w280 w311 w342 w373 w404 w435 w466 w497 w528 w559 w590 w621 w652 w683 w714 w745 w776 w807 w838 w870 w902 w961 w1001 w1041 w1079 w1128 w1165 w1202 w1239 w1276 w1313 w1350 w1387 w1424 w1461 w1498 w1535 w1572 w1609 w1646 w1683 w1720 w1757 w1797 w1837 w1890 w1921 w1947 w1996 w2061]
      tunnel: [_ w60 w91 w124 w151 w182 w213 w244 w275 w306 w337 w368 w399 w430 w461 w492 w523 w554 w585 w616 w647 w678 w709 w740 w771 w802 w833 w865 w896 w955 w995 w1035 w1073 w1122 w1159 w1196 w1233 w1270 w1307 w1344 w1381 w1418 w1455 w1492 w1529 w1566 w1603 w1640 w1677 w1714 w1751 w1791 w1831 w1872 w1904 w1943 w1991 w2058] -> w32
      tunnel: w35 -> [_ _ _ _ _ _ _ _ _ _ _ _ _ _ _ _ _ _ _ _ _ _ _ _ _ _ _ _ _ _ _ _ _ _ _ _ _ _ _ _ _ _ _ _ _ _ _ _ _ _ _ _ _ _ _ _ _ _]
      tunnel: [_ "5.2.3_2 Verify Connection to UUT through EOL Test command" "5.2.3_3 Check Environment value from Lux sensor via I2C host" "5.2.3_4 Start Test mode" "5.2.3_5 Start camera test mode" "5.2.3_6 To Open VLC for video stream setting" "5.2.3_7 Adjust the XYZ-axis linear stage" "5.2.3_8 Config external Light as table as right column" "5.2.3_9 Creating a Test profiles for camera LED" "5.2.3_10 Check Test item Reflection result" "5.2.3_11 Check Test item Uniformatiy mean result" "5.2.3_12 Check Test item Uniformity Standard result" "5.2.3_13 Check Test item Distortation_Center X result" "5.2.3_14 Check Test item Distortation_Center Y result" "5.2.3_15 Check Test item Distortation  result" "5.2.3_16 Check Test item MFT50 result" "5.2.3_17 Check Test item Rise Distance result" "5.2.3_18 VQT Metrics Results" "5.2.3_19 Check Test item RBdeltaE result" "5.2.3_20 Check Test item BWdeltaE result" "5.2.3_21 Check Test item WRdeltaE result" "5.2.3_22 Check Test item deltaa result" "5.2.3_23 Check Test item deltab result" "5.2.3_24 Color Check Results" "5.2.3_25 Stop Camera" "5.2.3_26 Stop Test mode" "5.2.3_27 Shutdown UUT" "Disconnect_UUT" " Start Test mode " "Start camera test mode" "Open VLC for video stream setting" "Adjust motor to alignment ROI overlay" "Config external Light" "Creating a Test profiles for camera LED" "Check Test item “Reflection” result" "Check Test item “Uniformatiy mean” result" "Check Test item “Uniformity Standard” result " "Check Test item “Distortation_Center X” result" "Check Test item “Distortation_Center Y” result" "Check Test item “Distortation %” result" "Check Test item “MFT50” result" "Check Test item “Rise Distance” result" "VQT Test result " "Check Test item” RBdeltaE” result" "Check Test item” BWdeltaE” result" "Check Test item” WRdeltaE” result" " Check Test item” deltaa” result" "Check Test item” deltab” result" "Color Check Results" "Stop Camera" "Stop Test mode" "Shutdown UUT" "Shutdown UUT" w1870 w1893 w1923 "BOOST_Get_AW_Calibration_value" w2052] -> w34
      tunnel: [_ _ _ _ _ _ _ _ _ _ _ _ _ _ _ _ _ _ _ _ _ _ _ _ _ _ _ _ w894 w953 w993 w1033 w1071 w1120 w1157 w1194 w1231 w1268 w1305 w1342 w1379 w1416 w1453 w1490 w1527 w1564 w1601 w1638 w1675 w1712 w1749 w1789 w1829 w1870 w1893 w1940 w1987 w2052] -> w31
      tunnel: w24 -> [_ _ _ _ _ _ _ _ _ _ _ _ _ _ _ _ _ _ _ _ _ _ _ _ _ _ _ _ _ _ _ _ _ _ _ _ _ _ _ _ _ _ _ _ _ _ _ _ _ _ _ _ _ w1864 w1897 w1925 w1971 w2036]
      tunnel: [w50 w56 w87 w117 w147 w178 w209 w240 w271 w302 w333 w364 w395 w426 w457 w488 w519 w550 w581 w612 w643 w674 w705 w736 w767 w798 w829 w861 w890 w949 w989 w1029 w1067 w1116 w1153 w1190 w1227 w1264 w1301 w1338 w1375 w1412 w1449 w1486 w1523 w1560 w1597 w1634 w1671 w1708 w1745 w1785 w1825 w1865 w1896 w1933 w1980 w2043] -> w23
      tunnel: w22 -> [w50 w56 w87 w118 w147 w178 w209 w240 w271 w302 w333 w364 w395 w426 w457 w488 w519 w550 w581 w612 w643 w674 w705 w736 w767 w798 w829 w861 w890 w949 w989 w1029 w1067 w1116 w1153 w1190 w1227 w1264 w1301 w1338 w1375 w1412 w1449 w1486 w1523 w1560 w1597 w1634 w1671 w1708 w1745 w1785 w1825 w1866 w1895 w1936 w1983 w2047]
      tunnel: w18 -> [_ w54 w85 w119 w145 w176 w207 w238 w269 w300 w331 w362 w393 w424 w455 w486 w517 w548 w579 w610 w641 w672 w703 w734 w765 w796 w827 w859 _ w948 w988 w1028 w1066 w1115 w1152 w1189 w1226 w1263 w1300 w1337 w1374 w1411 w1448 w1485 w1522 w1559 w1596 w1633 w1670 w1707 w1744 w1784 w1824 _ _ _ _ _]
      frame "假", Default {
      }
      frame "5.2.3_1 Make sure the USB type C cable is connected to the UUT" {
        n8 = Unbundle By Name(w56) -> ("Table"=w61:string[][])
        n9 = call "Select_Table_Vaule Enable_Disable.vi"("Action"=w60, "Table"=w61) -> ("Enable"=w59:bool)  [unwired: 8 in, 1 out]
        n10 = case shown="True" w59 {
          tunnel: ["Skip" ("response") w71] -> w62
          tunnel: w61 -> [_ w77]
          tunnel: w60 -> [_ w76]
          tunnel: [_ w69] -> w57
          tunnel: w54 -> [_ w72]
          frame False {
          }
          frame True {
            w83 = "UIdisplay" ("Process (\"\" - local)")
            n11 = Unbundle By Name(w72) -> ("Start Test mode"=w73:string)
            n12 = call "SendCmd.vi"("cmd"=w73, "exe"="D:\\Program Files\\MVTec\\HALCON-17.12-Progress\\bin\\x64-win64\\hdevelop.exe") -> ("error out"=w70:errorcluster, "standard output"=w71:string)  [unwired: 6 in, 2 out]
            n13 = call <vilib>:"Clear Errors.vi"("error in (no error)"=w70) -> ("error out"=w69:errorcluster)  [unwired: 5 in, 1 out]
            n14 = call "Select_Table_Vaule.vi"("Vaule"=w71, "Action"=w76, "Table"=w77) -> ("Result"=w78:bool, "vaule"=w84:string[])  [unwired: 7 in]
            n15 = Append True/False String(1:w78, 2:"FAIL" ("真字符串"), 3:"PASS" ("真字符串")) -> (0:w75:string)  [unwired: 1 in]
            n16 = Build Array (concatenate)(w84, w71, w75) -> (w82:string[])
            n17 = Flatten To XML(anything=w82) -> (xml string=w81:string)
            n18 = call "AMC Send Local Message.vi"("Process (\"\" - local)"=w83, "Message Value"=w81, "Message Name"=w83) -> ()  [unwired: 7 in, 2 out]
          }
        }
        n19 = call <vilib>:"Space Constant.vi"() -> ("String"=w63:string)
        n20 = Concatenate Strings(w60, w63, w62) -> (w64:string)
        n21 = call "LogStatus.vi"("error in (no error)"=w57, "last message"=w65, "message"=w64) -> ("error  out"=w66:errorcluster)  [unwired: 8 in]
      }
      frame "5.2.3_2 Verify Connection to UUT through EOL Test command" {
        n22 = Unbundle By Name(w87) -> ("Table"=w92:string[][])
        n23 = call "Select_Table_Vaule Enable_Disable.vi"("Action"=w91, "Table"=w92) -> ("Enable"=w90:bool)  [unwired: 8 in, 1 out]
        n24 = case shown="True" w90 {
          tunnel: ["Skip" ("response") w102] -> w93
          tunnel: w92 -> [_ w108]
          tunnel: w91 -> [_ w107]
          tunnel: [_ w100] -> w88
          tunnel: w85 -> [_ w103]
          frame False {
          }
          frame True {
            w114 = "UIdisplay" ("Process (\"\" - local)")
            n25 = Unbundle By Name(w103) -> ("Start Test mode"=w104:string)
            n26 = call "SendCmd.vi"("cmd"=w104, "exe"="D:\\Program Files\\MVTec\\HALCON-17.12-Progress\\bin\\x64-win64\\hdevelop.exe") -> ("error out"=w101:errorcluster, "standard output"=w102:string)  [unwired: 6 in, 2 out]
            n27 = call <vilib>:"Clear Errors.vi"("error in (no error)"=w101) -> ("error out"=w100:errorcluster)  [unwired: 5 in, 1 out]
            n28 = call "Select_Table_Vaule.vi"("Vaule"=w102, "Action"=w107, "Table"=w108) -> ("Result"=w109:bool, "vaule"=w115:string[])  [unwired: 7 in]
            n29 = Append True/False String(1:w109, 2:"FAIL" ("真字符串"), 3:"PASS" ("真字符串")) -> (0:w106:string)  [unwired: 1 in]
            n30 = Build Array (concatenate)(w115, w102, w106) -> (w113:string[])
            n31 = Flatten To XML(anything=w113) -> (xml string=w112:string)
            n32 = call "AMC Send Local Message.vi"("Process (\"\" - local)"=w114, "Message Value"=w112, "Message Name"=w114) -> ()  [unwired: 7 in, 2 out]
          }
        }
        n33 = call <vilib>:"Space Constant.vi"() -> ("String"=w94:string)
        n34 = Concatenate Strings(w91, w94, w93) -> (w95:string)
        n35 = call "LogStatus.vi"("error in (no error)"=w88, "last message"=w96, "message"=w95) -> ("error  out"=w97:errorcluster)  [unwired: 8 in]
      }
      frame "5.2.3_3 Check Environment value from Lux sensor via I2C host" {
        n36 = Unbundle By Name(w118) -> ("Table"=w125:string[][])
        n37 = call "Select_Table_Vaule Enable_Disable.vi"("Action"=w124, "Table"=w125) -> ("Enable"=w123:bool)  [unwired: 8 in, 1 out]
        n38 = case shown="True" w123 {
          tunnel: [w132 w133] -> w126
          tunnel: w125 -> [_ w137]
          tunnel: w124 -> [_ w136]
          tunnel: [_ w134] -> w121
          tunnel: w119 -> [_ _]
          tunnel: [w132 w133] -> w116
          frame False {
            w132 = "Skip" ("response")
          }
          frame True {
            w143 = "UIdisplay" ("Process (\"\" - local)")
            n39 = call "Read_Lux.vi"() -> ("error out"=w134:errorcluster, "Lux_Value"=w133:string)  [unwired: 9 in, 1 out]
            n40 = call "Select_Table_Vaule.vi"("Vaule"=w133, "Action"=w136, "Table"=w137) -> ("Result"=w138:bool, "vaule"=w144:string[])  [unwired: 7 in]
            n41 = Append True/False String(1:w138, 2:"FAIL" ("真字符串"), 3:"PASS" ("真字符串")) -> (0:w135:string)  [unwired: 1 in]
            n42 = Build Array (concatenate)(w144, w133, w135) -> (w142:string[])
            n43 = Flatten To XML(anything=w142) -> (xml string=w141:string)
            n44 = call "AMC Send Local Message.vi"("Process (\"\" - local)"=w143, "Message Value"=w141, "Message Name"=w143) -> ()  [unwired: 7 in, 2 out]
          }
        }
        n45 = call <vilib>:"Space Constant.vi"() -> ("String"=w127:string)
        n46 = Concatenate Strings(w124, w127, w126) -> (w128:string)
        n47 = Bundle By Name(cluster=w118, "Lux"=w116) -> (w117:T1)
        n48 = call "LogStatus.vi"("error in (no error)"=w121, "last message"=w129, "message"=w128) -> ("error  out"=w130:errorcluster)  [unwired: 8 in]
      }
      frame "5.2.3_4 Start Test mode" {
        n49 = Unbundle By Name(w147) -> ("Table"=w152:string[][])
        n50 = call "Select_Table_Vaule Enable_Disable.vi"("Action"=w151, "Table"=w152) -> ("Enable"=w150:bool)  [unwired: 8 in, 1 out]
        n51 = case shown="True" w150 {
          tunnel: ["Skip" ("response") w162] -> w153
          tunnel: w152 -> [_ w168]
          tunnel: w151 -> [_ w167]
          tunnel: [_ w160] -> w148
          tunnel: w145 -> [_ w163]
          frame False {
          }
          frame True {
            w174 = "UIdisplay" ("Process (\"\" - local)")
            n52 = Unbundle By Name(w163) -> ("Start Test mode"=w164:string)
            n53 = call "SendCmd.vi"("cmd"=w164, "exe"="D:\\Program Files\\MVTec\\HALCON-17.12-Progress\\bin\\x64-win64\\hdevelop.exe") -> ("error out"=w161:errorcluster, "standard output"=w162:string)  [unwired: 6 in, 2 out]
            n54 = call <vilib>:"Clear Errors.vi"("error in (no error)"=w161) -> ("error out"=w160:errorcluster)  [unwired: 5 in, 1 out]
            n55 = call "Select_Table_Vaule.vi"("Vaule"=w162, "Action"=w167, "Table"=w168) -> ("Result"=w169:bool, "vaule"=w175:string[])  [unwired: 7 in]
            n56 = Append True/False String(1:w169, 2:"FAIL" ("真字符串"), 3:"PASS" ("真字符串")) -> (0:w166:string)  [unwired: 1 in]
            n57 = Build Array (concatenate)(w175, w162, w166) -> (w173:string[])
            n58 = Flatten To XML(anything=w173) -> (xml string=w172:string)
            n59 = call "AMC Send Local Message.vi"("Process (\"\" - local)"=w174, "Message Value"=w172, "Message Name"=w174) -> ()  [unwired: 7 in, 2 out]
          }
        }
        n60 = call <vilib>:"Space Constant.vi"() -> ("String"=w154:string)
        n61 = Concatenate Strings(w151, w154, w153) -> (w155:string)
        n62 = call "LogStatus.vi"("error in (no error)"=w148, "last message"=w156, "message"=w155) -> ("error  out"=w157:errorcluster)  [unwired: 8 in]
      }
      frame "5.2.3_5 Start camera test mode" {
        n63 = Unbundle By Name(w178) -> ("Table"=w183:string[][])
        n64 = call "Select_Table_Vaule Enable_Disable.vi"("Action"=w182, "Table"=w183) -> ("Enable"=w181:bool)  [unwired: 8 in, 1 out]
        n65 = case shown="True" w181 {
          tunnel: ["Skip" ("response") w193] -> w184
          tunnel: w183 -> [_ w199]
          tunnel: w182 -> [_ w198]
          tunnel: [_ w191] -> w179
          tunnel: w176 -> [_ w194]
          frame False {
          }
          frame True {
            w205 = "UIdisplay" ("Process (\"\" - local)")
            n66 = Unbundle By Name(w194) -> ("Start Test mode"=w195:string)
            n67 = call "SendCmd.vi"("cmd"=w195, "exe"="D:\\Program Files\\MVTec\\HALCON-17.12-Progress\\bin\\x64-win64\\hdevelop.exe") -> ("error out"=w192:errorcluster, "standard output"=w193:string)  [unwired: 6 in, 2 out]
            n68 = call <vilib>:"Clear Errors.vi"("error in (no error)"=w192) -> ("error out"=w191:errorcluster)  [unwired: 5 in, 1 out]
            n69 = call "Select_Table_Vaule.vi"("Vaule"=w193, "Action"=w198, "Table"=w199) -> ("Result"=w200:bool, "vaule"=w206:string[])  [unwired: 7 in]
            n70 = Append True/False String(1:w200, 2:"FAIL" ("真字符串"), 3:"PASS" ("真字符串")) -> (0:w197:string)  [unwired: 1 in]
            n71 = Build Array (concatenate)(w206, w193, w197) -> (w204:string[])
            n72 = Flatten To XML(anything=w204) -> (xml string=w203:string)
            n73 = call "AMC Send Local Message.vi"("Process (\"\" - local)"=w205, "Message Value"=w203, "Message Name"=w205) -> ()  [unwired: 7 in, 2 out]
          }
        }
        n74 = call <vilib>:"Space Constant.vi"() -> ("String"=w185:string)
        n75 = Concatenate Strings(w182, w185, w184) -> (w186:string)
        n76 = call "LogStatus.vi"("error in (no error)"=w179, "last message"=w187, "message"=w186) -> ("error  out"=w188:errorcluster)  [unwired: 8 in]
      }
      frame "5.2.3_6 To Open VLC for video stream setting" {
        n77 = Unbundle By Name(w209) -> ("Table"=w214:string[][])
        n78 = call "Select_Table_Vaule Enable_Disable.vi"("Action"=w213, "Table"=w214) -> ("Enable"=w212:bool)  [unwired: 8 in, 1 out]
        n79 = case shown="True" w212 {
          tunnel: ["Skip" ("response") w224] -> w215
          tunnel: w214 -> [_ w230]
          tunnel: w213 -> [_ w229]
          tunnel: [_ w222] -> w210
          tunnel: w207 -> [_ w225]
          frame False {
          }
          frame True {
            w236 = "UIdisplay" ("Process (\"\" - local)")
            n80 = Unbundle By Name(w225) -> ("Start Test mode"=w226:string)
            n81 = call "SendCmd.vi"("cmd"=w226, "exe"="D:\\Program Files\\MVTec\\HALCON-17.12-Progress\\bin\\x64-win64\\hdevelop.exe") -> ("error out"=w223:errorcluster, "standard output"=w224:string)  [unwired: 6 in, 2 out]
            n82 = call <vilib>:"Clear Errors.vi"("error in (no error)"=w223) -> ("error out"=w222:errorcluster)  [unwired: 5 in, 1 out]
            n83 = call "Select_Table_Vaule.vi"("Vaule"=w224, "Action"=w229, "Table"=w230) -> ("Result"=w231:bool, "vaule"=w237:string[])  [unwired: 7 in]
            n84 = Append True/False String(1:w231, 2:"FAIL" ("真字符串"), 3:"PASS" ("真字符串")) -> (0:w228:string)  [unwired: 1 in]
            n85 = Build Array (concatenate)(w237, w224, w228) -> (w235:string[])
            n86 = Flatten To XML(anything=w235) -> (xml string=w234:string)
            n87 = call "AMC Send Local Message.vi"("Process (\"\" - local)"=w236, "Message Value"=w234, "Message Name"=w236) -> ()  [unwired: 7 in, 2 out]
          }
        }
        n88 = call <vilib>:"Space Constant.vi"() -> ("String"=w216:string)
        n89 = Concatenate Strings(w213, w216, w215) -> (w217:string)
        n90 = call "LogStatus.vi"("error in (no error)"=w210, "last message"=w218, "message"=w217) -> ("error  out"=w219:errorcluster)  [unwired: 8 in]
      }
      frame "5.2.3_7 Adjust the XYZ-axis linear stage" {
        n91 = Unbundle By Name(w240) -> ("Table"=w245:string[][])
        n92 = call "Select_Table_Vaule Enable_Disable.vi"("Action"=w244, "Table"=w245) -> ("Enable"=w243:bool)  [unwired: 8 in, 1 out]
        n93 = case shown="True" w243 {
          tunnel: ["Skip" ("response") w255] -> w246
          tunnel: w245 -> [_ w261]
          tunnel: w244 -> [_ w260]
          tunnel: [_ w253] -> w241
          tunnel: w238 -> [_ w256]
          frame False {
          }
          frame True {
            w267 = "UIdisplay" ("Process (\"\" - local)")
            n94 = Unbundle By Name(w256) -> ("Start Test mode"=w257:string)
            n95 = call "SendCmd.vi"("cmd"=w257, "exe"="D:\\Program Files\\MVTec\\HALCON-17.12-Progress\\bin\\x64-win64\\hdevelop.exe") -> ("error out"=w254:errorcluster, "standard output"=w255:string)  [unwired: 6 in, 2 out]
            n96 = call <vilib>:"Clear Errors.vi"("error in (no error)"=w254) -> ("error out"=w253:errorcluster)  [unwired: 5 in, 1 out]
            n97 = call "Select_Table_Vaule.vi"("Vaule"=w255, "Action"=w260, "Table"=w261) -> ("Result"=w262:bool, "vaule"=w268:string[])  [unwired: 7 in]
            n98 = Append True/False String(1:w262, 2:"FAIL" ("真字符串"), 3:"PASS" ("真字符串")) -> (0:w259:string)  [unwired: 1 in]
            n99 = Build Array (concatenate)(w268, w255, w259) -> (w266:string[])
            n100 = Flatten To XML(anything=w266) -> (xml string=w265:string)
            n101 = call "AMC Send Local Message.vi"("Process (\"\" - local)"=w267, "Message Value"=w265, "Message Name"=w267) -> ()  [unwired: 7 in, 2 out]
          }
        }
        n102 = call <vilib>:"Space Constant.vi"() -> ("String"=w247:string)
        n103 = Concatenate Strings(w244, w247, w246) -> (w248:string)
        n104 = call "LogStatus.vi"("error in (no error)"=w241, "last message"=w249, "message"=w248) -> ("error  out"=w250:errorcluster)  [unwired: 8 in]
      }
      frame "5.2.3_8 Config external Light as table as right column" {
        n105 = Unbundle By Name(w271) -> ("Table"=w276:string[][])
        n106 = call "Select_Table_Vaule Enable_Disable.vi"("Action"=w275, "Table"=w276) -> ("Enable"=w274:bool)  [unwired: 8 in, 1 out]
        n107 = case shown="True" w274 {
          tunnel: ["Skip" ("response") w286] -> w277
          tunnel: w276 -> [_ w292]
          tunnel: w275 -> [_ w291]
          tunnel: [_ w284] -> w272
          tunnel: w269 -> [_ w287]
          frame False {
          }
          frame True {
            w298 = "UIdisplay" ("Process (\"\" - local)")
            n108 = Unbundle By Name(w287) -> ("Start Test mode"=w288:string)
            n109 = call "SendCmd.vi"("cmd"=w288, "exe"="D:\\Program Files\\MVTec\\HALCON-17.12-Progress\\bin\\x64-win64\\hdevelop.exe") -> ("error out"=w285:errorcluster, "standard output"=w286:string)  [unwired: 6 in, 2 out]
            n110 = call <vilib>:"Clear Errors.vi"("error in (no error)"=w285) -> ("error out"=w284:errorcluster)  [unwired: 5 in, 1 out]
            n111 = call "Select_Table_Vaule.vi"("Vaule"=w286, "Action"=w291, "Table"=w292) -> ("Result"=w293:bool, "vaule"=w299:string[])  [unwired: 7 in]
            n112 = Append True/False String(1:w293, 2:"FAIL" ("真字符串"), 3:"PASS" ("真字符串")) -> (0:w290:string)  [unwired: 1 in]
            n113 = Build Array (concatenate)(w299, w286, w290) -> (w297:string[])
            n114 = Flatten To XML(anything=w297) -> (xml string=w296:string)
            n115 = call "AMC Send Local Message.vi"("Process (\"\" - local)"=w298, "Message Value"=w296, "Message Name"=w298) -> ()  [unwired: 7 in, 2 out]
          }
        }
        n116 = call <vilib>:"Space Constant.vi"() -> ("String"=w278:string)
        n117 = Concatenate Strings(w275, w278, w277) -> (w279:string)
        n118 = call "LogStatus.vi"("error in (no error)"=w272, "last message"=w280, "message"=w279) -> ("error  out"=w281:errorcluster)  [unwired: 8 in]
      }
      frame "5.2.3_9 Creating a Test profiles for camera LED" {
        n119 = Unbundle By Name(w302) -> ("Table"=w307:string[][])
        n120 = call "Select_Table_Vaule Enable_Disable.vi"("Action"=w306, "Table"=w307) -> ("Enable"=w305:bool)  [unwired: 8 in, 1 out]
        n121 = case shown="True" w305 {
          tunnel: ["Skip" ("response") w317] -> w308
          tunnel: w307 -> [_ w323]
          tunnel: w306 -> [_ w322]
          tunnel: [_ w315] -> w303
          tunnel: w300 -> [_ w318]
          frame False {
          }
          frame True {
            w329 = "UIdisplay" ("Process (\"\" - local)")
            n122 = Unbundle By Name(w318) -> ("Start Test mode"=w319:string)
            n123 = call "SendCmd.vi"("cmd"=w319, "exe"="D:\\Program Files\\MVTec\\HALCON-17.12-Progress\\bin\\x64-win64\\hdevelop.exe") -> ("error out"=w316:errorcluster, "standard output"=w317:string)  [unwired: 6 in, 2 out]
            n124 = call <vilib>:"Clear Errors.vi"("error in (no error)"=w316) -> ("error out"=w315:errorcluster)  [unwired: 5 in, 1 out]
            n125 = call "Select_Table_Vaule.vi"("Vaule"=w317, "Action"=w322, "Table"=w323) -> ("Result"=w324:bool, "vaule"=w330:string[])  [unwired: 7 in]
            n126 = Append True/False String(1:w324, 2:"FAIL" ("真字符串"), 3:"PASS" ("真字符串")) -> (0:w321:string)  [unwired: 1 in]
            n127 = Build Array (concatenate)(w330, w317, w321) -> (w328:string[])
            n128 = Flatten To XML(anything=w328) -> (xml string=w327:string)
            n129 = call "AMC Send Local Message.vi"("Process (\"\" - local)"=w329, "Message Value"=w327, "Message Name"=w329) -> ()  [unwired: 7 in, 2 out]
          }
        }
        n130 = call <vilib>:"Space Constant.vi"() -> ("String"=w309:string)
        n131 = Concatenate Strings(w306, w309, w308) -> (w310:string)
        n132 = call "LogStatus.vi"("error in (no error)"=w303, "last message"=w311, "message"=w310) -> ("error  out"=w312:errorcluster)  [unwired: 8 in]
      }
      frame "5.2.3_10 Check Test item Reflection result" {
        n133 = Unbundle By Name(w333) -> ("Table"=w338:string[][])
        n134 = call "Select_Table_Vaule Enable_Disable.vi"("Action"=w337, "Table"=w338) -> ("Enable"=w336:bool)  [unwired: 8 in, 1 out]
        n135 = case shown="True" w336 {
          tunnel: ["Skip" ("response") w348] -> w339
          tunnel: w338 -> [_ w354]
          tunnel: w337 -> [_ w353]
          tunnel: [_ w346] -> w334
          tunnel: w331 -> [_ w349]
          frame False {
          }
          frame True {
            w360 = "UIdisplay" ("Process (\"\" - local)")
            n136 = Unbundle By Name(w349) -> ("Start Test mode"=w350:string)
            n137 = call "SendCmd.vi"("cmd"=w350, "exe"="D:\\Program Files\\MVTec\\HALCON-17.12-Progress\\bin\\x64-win64\\hdevelop.exe") -> ("error out"=w347:errorcluster, "standard output"=w348:string)  [unwired: 6 in, 2 out]
            n138 = call <vilib>:"Clear Errors.vi"("error in (no error)"=w347) -> ("error out"=w346:errorcluster)  [unwired: 5 in, 1 out]
            n139 = call "Select_Table_Vaule.vi"("Vaule"=w348, "Action"=w353, "Table"=w354) -> ("Result"=w355:bool, "vaule"=w361:string[])  [unwired: 7 in]
            n140 = Append True/False String(1:w355, 2:"FAIL" ("真字符串"), 3:"PASS" ("真字符串")) -> (0:w352:string)  [unwired: 1 in]
            n141 = Build Array (concatenate)(w361, w348, w352) -> (w359:string[])
            n142 = Flatten To XML(anything=w359) -> (xml string=w358:string)
            n143 = call "AMC Send Local Message.vi"("Process (\"\" - local)"=w360, "Message Value"=w358, "Message Name"=w360) -> ()  [unwired: 7 in, 2 out]
          }
        }
        n144 = call <vilib>:"Space Constant.vi"() -> ("String"=w340:string)
        n145 = Concatenate Strings(w337, w340, w339) -> (w341:string)
        n146 = call "LogStatus.vi"("error in (no error)"=w334, "last message"=w342, "message"=w341) -> ("error  out"=w343:errorcluster)  [unwired: 8 in]
      }
      frame "5.2.3_11 Check Test item Uniformatiy mean result" {
        n147 = Unbundle By Name(w364) -> ("Table"=w369:string[][])
        n148 = call "Select_Table_Vaule Enable_Disable.vi"("Action"=w368, "Table"=w369) -> ("Enable"=w367:bool)  [unwired: 8 in, 1 out]
        n149 = case shown="True" w367 {
          tunnel: ["Skip" ("response") w379] -> w370
          tunnel: w369 -> [_ w385]
          tunnel: w368 -> [_ w384]
          tunnel: [_ w377] -> w365
          tunnel: w362 -> [_ w380]
          frame False {
          }
          frame True {
            w391 = "UIdisplay" ("Process (\"\" - local)")
            n150 = Unbundle By Name(w380) -> ("Start Test mode"=w381:string)
            n151 = call "SendCmd.vi"("cmd"=w381, "exe"="D:\\Program Files\\MVTec\\HALCON-17.12-Progress\\bin\\x64-win64\\hdevelop.exe") -> ("error out"=w378:errorcluster, "standard output"=w379:string)  [unwired: 6 in, 2 out]
            n152 = call <vilib>:"Clear Errors.vi"("error in (no error)"=w378) -> ("error out"=w377:errorcluster)  [unwired: 5 in, 1 out]
            n153 = call "Select_Table_Vaule.vi"("Vaule"=w379, "Action"=w384, "Table"=w385) -> ("Result"=w386:bool, "vaule"=w392:string[])  [unwired: 7 in]
            n154 = Append True/False String(1:w386, 2:"FAIL" ("真字符串"), 3:"PASS" ("真字符串")) -> (0:w383:string)  [unwired: 1 in]
            n155 = Build Array (concatenate)(w392, w379, w383) -> (w390:string[])
            n156 = Flatten To XML(anything=w390) -> (xml string=w389:string)
            n157 = call "AMC Send Local Message.vi"("Process (\"\" - local)"=w391, "Message Value"=w389, "Message Name"=w391) -> ()  [unwired: 7 in, 2 out]
          }
        }
        n158 = call <vilib>:"Space Constant.vi"() -> ("String"=w371:string)
        n159 = Concatenate Strings(w368, w371, w370) -> (w372:string)
        n160 = call "LogStatus.vi"("error in (no error)"=w365, "last message"=w373, "message"=w372) -> ("error  out"=w374:errorcluster)  [unwired: 8 in]
      }
      frame "5.2.3_12 Check Test item Uniformity Standard result" {
        n161 = Unbundle By Name(w395) -> ("Table"=w400:string[][])
        n162 = call "Select_Table_Vaule Enable_Disable.vi"("Action"=w399, "Table"=w400) -> ("Enable"=w398:bool)  [unwired: 8 in, 1 out]
        n163 = case shown="True" w398 {
          tunnel: ["Skip" ("response") w410] -> w401
          tunnel: w400 -> [_ w416]
          tunnel: w399 -> [_ w415]
          tunnel: [_ w408] -> w396
          tunnel: w393 -> [_ w411]
          frame False {
          }
          frame True {
            w422 = "UIdisplay" ("Process (\"\" - local)")
            n164 = Unbundle By Name(w411) -> ("Start Test mode"=w412:string)
            n165 = call "SendCmd.vi"("cmd"=w412, "exe"="D:\\Program Files\\MVTec\\HALCON-17.12-Progress\\bin\\x64-win64\\hdevelop.exe") -> ("error out"=w409:errorcluster, "standard output"=w410:string)  [unwired: 6 in, 2 out]
            n166 = call <vilib>:"Clear Errors.vi"("error in (no error)"=w409) -> ("error out"=w408:errorcluster)  [unwired: 5 in, 1 out]
            n167 = call "Select_Table_Vaule.vi"("Vaule"=w410, "Action"=w415, "Table"=w416) -> ("Result"=w417:bool, "vaule"=w423:string[])  [unwired: 7 in]
            n168 = Append True/False String(1:w417, 2:"FAIL" ("真字符串"), 3:"PASS" ("真字符串")) -> (0:w414:string)  [unwired: 1 in]
            n169 = Build Array (concatenate)(w423, w410, w414) -> (w421:string[])
            n170 = Flatten To XML(anything=w421) -> (xml string=w420:string)
            n171 = call "AMC Send Local Message.vi"("Process (\"\" - local)"=w422, "Message Value"=w420, "Message Name"=w422) -> ()  [unwired: 7 in, 2 out]
          }
        }
        n172 = call <vilib>:"Space Constant.vi"() -> ("String"=w402:string)
        n173 = Concatenate Strings(w399, w402, w401) -> (w403:string)
        n174 = call "LogStatus.vi"("error in (no error)"=w396, "last message"=w404, "message"=w403) -> ("error  out"=w405:errorcluster)  [unwired: 8 in]
      }
      frame "5.2.3_13 Check Test item Distortation_Center X result" {
        n175 = Unbundle By Name(w426) -> ("Table"=w431:string[][])
        n176 = call "Select_Table_Vaule Enable_Disable.vi"("Action"=w430, "Table"=w431) -> ("Enable"=w429:bool)  [unwired: 8 in, 1 out]
        n177 = case shown="True" w429 {
          tunnel: ["Skip" ("response") w441] -> w432
          tunnel: w431 -> [_ w447]
          tunnel: w430 -> [_ w446]
          tunnel: [_ w439] -> w427
          tunnel: w424 -> [_ w442]
          frame False {
          }
          frame True {
            w453 = "UIdisplay" ("Process (\"\" - local)")
            n178 = Unbundle By Name(w442) -> ("Start Test mode"=w443:string)
            n179 = call "SendCmd.vi"("cmd"=w443, "exe"="D:\\Program Files\\MVTec\\HALCON-17.12-Progress\\bin\\x64-win64\\hdevelop.exe") -> ("error out"=w440:errorcluster, "standard output"=w441:string)  [unwired: 6 in, 2 out]
            n180 = call <vilib>:"Clear Errors.vi"("error in (no error)"=w440) -> ("error out"=w439:errorcluster)  [unwired: 5 in, 1 out]
            n181 = call "Select_Table_Vaule.vi"("Vaule"=w441, "Action"=w446, "Table"=w447) -> ("Result"=w448:bool, "vaule"=w454:string[])  [unwired: 7 in]
            n182 = Append True/False String(1:w448, 2:"FAIL" ("真字符串"), 3:"PASS" ("真字符串")) -> (0:w445:string)  [unwired: 1 in]
            n183 = Build Array (concatenate)(w454, w441, w445) -> (w452:string[])
            n184 = Flatten To XML(anything=w452) -> (xml string=w451:string)
            n185 = call "AMC Send Local Message.vi"("Process (\"\" - local)"=w453, "Message Value"=w451, "Message Name"=w453) -> ()  [unwired: 7 in, 2 out]
          }
        }
        n186 = call <vilib>:"Space Constant.vi"() -> ("String"=w433:string)
        n187 = Concatenate Strings(w430, w433, w432) -> (w434:string)
        n188 = call "LogStatus.vi"("error in (no error)"=w427, "last message"=w435, "message"=w434) -> ("error  out"=w436:errorcluster)  [unwired: 8 in]
      }
      frame "5.2.3_14 Check Test item Distortation_Center Y result" {
        n189 = Unbundle By Name(w457) -> ("Table"=w462:string[][])
        n190 = call "Select_Table_Vaule Enable_Disable.vi"("Action"=w461, "Table"=w462) -> ("Enable"=w460:bool)  [unwired: 8 in, 1 out]
        n191 = case shown="True" w460 {
          tunnel: ["Skip" ("response") w472] -> w463
          tunnel: w462 -> [_ w478]
          tunnel: w461 -> [_ w477]
          tunnel: [_ w470] -> w458
          tunnel: w455 -> [_ w473]
          frame False {
          }
          frame True {
            w484 = "UIdisplay" ("Process (\"\" - local)")
            n192 = Unbundle By Name(w473) -> ("Start Test mode"=w474:string)
            n193 = call "SendCmd.vi"("cmd"=w474, "exe"="D:\\Program Files\\MVTec\\HALCON-17.12-Progress\\bin\\x64-win64\\hdevelop.exe") -> ("error out"=w471:errorcluster, "standard output"=w472:string)  [unwired: 6 in, 2 out]
            n194 = call <vilib>:"Clear Errors.vi"("error in (no error)"=w471) -> ("error out"=w470:errorcluster)  [unwired: 5 in, 1 out]
            n195 = call "Select_Table_Vaule.vi"("Vaule"=w472, "Action"=w477, "Table"=w478) -> ("Result"=w479:bool, "vaule"=w485:string[])  [unwired: 7 in]
            n196 = Append True/False String(1:w479, 2:"FAIL" ("真字符串"), 3:"PASS" ("真字符串")) -> (0:w476:string)  [unwired: 1 in]
            n197 = Build Array (concatenate)(w485, w472, w476) -> (w483:string[])
            n198 = Flatten To XML(anything=w483) -> (xml string=w482:string)
            n199 = call "AMC Send Local Message.vi"("Process (\"\" - local)"=w484, "Message Value"=w482, "Message Name"=w484) -> ()  [unwired: 7 in, 2 out]
          }
        }
        n200 = call <vilib>:"Space Constant.vi"() -> ("String"=w464:string)
        n201 = Concatenate Strings(w461, w464, w463) -> (w465:string)
        n202 = call "LogStatus.vi"("error in (no error)"=w458, "last message"=w466, "message"=w465) -> ("error  out"=w467:errorcluster)  [unwired: 8 in]
      }
      frame "5.2.3_15 Check Test item Distortation  result" {
        n203 = Unbundle By Name(w488) -> ("Table"=w493:string[][])
        n204 = call "Select_Table_Vaule Enable_Disable.vi"("Action"=w492, "Table"=w493) -> ("Enable"=w491:bool)  [unwired: 8 in, 1 out]
        n205 = case shown="True" w491 {
          tunnel: ["Skip" ("response") w503] -> w494
          tunnel: w493 -> [_ w509]
          tunnel: w492 -> [_ w508]
          tunnel: [_ w501] -> w489
          tunnel: w486 -> [_ w504]
          frame False {
          }
          frame True {
            w515 = "UIdisplay" ("Process (\"\" - local)")
            n206 = Unbundle By Name(w504) -> ("Start Test mode"=w505:string)
            n207 = call "SendCmd.vi"("cmd"=w505, "exe"="D:\\Program Files\\MVTec\\HALCON-17.12-Progress\\bin\\x64-win64\\hdevelop.exe") -> ("error out"=w502:errorcluster, "standard output"=w503:string)  [unwired: 6 in, 2 out]
            n208 = call <vilib>:"Clear Errors.vi"("error in (no error)"=w502) -> ("error out"=w501:errorcluster)  [unwired: 5 in, 1 out]
            n209 = call "Select_Table_Vaule.vi"("Vaule"=w503, "Action"=w508, "Table"=w509) -> ("Result"=w510:bool, "vaule"=w516:string[])  [unwired: 7 in]
            n210 = Append True/False String(1:w510, 2:"FAIL" ("真字符串"), 3:"PASS" ("真字符串")) -> (0:w507:string)  [unwired: 1 in]
            n211 = Build Array (concatenate)(w516, w503, w507) -> (w514:string[])
            n212 = Flatten To XML(anything=w514) -> (xml string=w513:string)
            n213 = call "AMC Send Local Message.vi"("Process (\"\" - local)"=w515, "Message Value"=w513, "Message Name"=w515) -> ()  [unwired: 7 in, 2 out]
          }
        }
        n214 = call <vilib>:"Space Constant.vi"() -> ("String"=w495:string)
        n215 = Concatenate Strings(w492, w495, w494) -> (w496:string)
        n216 = call "LogStatus.vi"("error in (no error)"=w489, "last message"=w497, "message"=w496) -> ("error  out"=w498:errorcluster)  [unwired: 8 in]
      }
      frame "5.2.3_16 Check Test item MFT50 result" {
        n217 = Unbundle By Name(w519) -> ("Table"=w524:string[][])
        n218 = call "Select_Table_Vaule Enable_Disable.vi"("Action"=w523, "Table"=w524) -> ("Enable"=w522:bool)  [unwired: 8 in, 1 out]
        n219 = case shown="True" w522 {
          tunnel: ["Skip" ("response") w534] -> w525
          tunnel: w524 -> [_ w540]
          tunnel: w523 -> [_ w539]
          tunnel: [_ w532] -> w520
          tunnel: w517 -> [_ w535]
          frame False {
          }
          frame True {
            w546 = "UIdisplay" ("Process (\"\" - local)")
            n220 = Unbundle By Name(w535) -> ("Start Test mode"=w536:string)
            n221 = call "SendCmd.vi"("cmd"=w536, "exe"="D:\\Program Files\\MVTec\\HALCON-17.12-Progress\\bin\\x64-win64\\hdevelop.exe") -> ("error out"=w533:errorcluster, "standard output"=w534:string)  [unwired: 6 in, 2 out]
            n222 = call <vilib>:"Clear Errors.vi"("error in (no error)"=w533) -> ("error out"=w532:errorcluster)  [unwired: 5 in, 1 out]
            n223 = call "Select_Table_Vaule.vi"("Vaule"=w534, "Action"=w539, "Table"=w540) -> ("Result"=w541:bool, "vaule"=w547:string[])  [unwired: 7 in]
            n224 = Append True/False String(1:w541, 2:"FAIL" ("真字符串"), 3:"PASS" ("真字符串")) -> (0:w538:string)  [unwired: 1 in]
            n225 = Build Array (concatenate)(w547, w534, w538) -> (w545:string[])
            n226 = Flatten To XML(anything=w545) -> (xml string=w544:string)
            n227 = call "AMC Send Local Message.vi"("Process (\"\" - local)"=w546, "Message Value"=w544, "Message Name"=w546) -> ()  [unwired: 7 in, 2 out]
          }
        }
        n228 = call <vilib>:"Space Constant.vi"() -> ("String"=w526:string)
        n229 = Concatenate Strings(w523, w526, w525) -> (w527:string)
        n230 = call "LogStatus.vi"("error in (no error)"=w520, "last message"=w528, "message"=w527) -> ("error  out"=w529:errorcluster)  [unwired: 8 in]
      }
      frame "5.2.3_17 Check Test item Rise Distance result" {
        n231 = Unbundle By Name(w550) -> ("Table"=w555:string[][])
        n232 = call "Select_Table_Vaule Enable_Disable.vi"("Action"=w554, "Table"=w555) -> ("Enable"=w553:bool)  [unwired: 8 in, 1 out]
        n233 = case shown="True" w553 {
          tunnel: ["Skip" ("response") w565] -> w556
          tunnel: w555 -> [_ w571]
          tunnel: w554 -> [_ w570]
          tunnel: [_ w563] -> w551
          tunnel: w548 -> [_ w566]
          frame False {
          }
          frame True {
            w577 = "UIdisplay" ("Process (\"\" - local)")
            n234 = Unbundle By Name(w566) -> ("Start Test mode"=w567:string)
            n235 = call "SendCmd.vi"("cmd"=w567, "exe"="D:\\Program Files\\MVTec\\HALCON-17.12-Progress\\bin\\x64-win64\\hdevelop.exe") -> ("error out"=w564:errorcluster, "standard output"=w565:string)  [unwired: 6 in, 2 out]
            n236 = call <vilib>:"Clear Errors.vi"("error in (no error)"=w564) -> ("error out"=w563:errorcluster)  [unwired: 5 in, 1 out]
            n237 = call "Select_Table_Vaule.vi"("Vaule"=w565, "Action"=w570, "Table"=w571) -> ("Result"=w572:bool, "vaule"=w578:string[])  [unwired: 7 in]
            n238 = Append True/False String(1:w572, 2:"FAIL" ("真字符串"), 3:"PASS" ("真字符串")) -> (0:w569:string)  [unwired: 1 in]
            n239 = Build Array (concatenate)(w578, w565, w569) -> (w576:string[])
            n240 = Flatten To XML(anything=w576) -> (xml string=w575:string)
            n241 = call "AMC Send Local Message.vi"("Process (\"\" - local)"=w577, "Message Value"=w575, "Message Name"=w577) -> ()  [unwired: 7 in, 2 out]
          }
        }
        n242 = call <vilib>:"Space Constant.vi"() -> ("String"=w557:string)
        n243 = Concatenate Strings(w554, w557, w556) -> (w558:string)
        n244 = call "LogStatus.vi"("error in (no error)"=w551, "last message"=w559, "message"=w558) -> ("error  out"=w560:errorcluster)  [unwired: 8 in]
      }
      frame "5.2.3_18 VQT Metrics Results" {
        n245 = Unbundle By Name(w581) -> ("Table"=w586:string[][])
        n246 = call "Select_Table_Vaule Enable_Disable.vi"("Action"=w585, "Table"=w586) -> ("Enable"=w584:bool)  [unwired: 8 in, 1 out]
        n247 = case shown="True" w584 {
          tunnel: ["Skip" ("response") w596] -> w587
          tunnel: w586 -> [_ w602]
          tunnel: w585 -> [_ w601]
          tunnel: [_ w594] -> w582
          tunnel: w579 -> [_ w597]
          frame False {
          }
          frame True {
            w608 = "UIdisplay" ("Process (\"\" - local)")
            n248 = Unbundle By Name(w597) -> ("Start Test mode"=w598:string)
            n249 = call "SendCmd.vi"("cmd"=w598, "exe"="D:\\Program Files\\MVTec\\HALCON-17.12-Progress\\bin\\x64-win64\\hdevelop.exe") -> ("error out"=w595:errorcluster, "standard output"=w596:string)  [unwired: 6 in, 2 out]
            n250 = call <vilib>:"Clear Errors.vi"("error in (no error)"=w595) -> ("error out"=w594:errorcluster)  [unwired: 5 in, 1 out]
            n251 = call "Select_Table_Vaule.vi"("Vaule"=w596, "Action"=w601, "Table"=w602) -> ("Result"=w603:bool, "vaule"=w609:string[])  [unwired: 7 in]
            n252 = Append True/False String(1:w603, 2:"FAIL" ("真字符串"), 3:"PASS" ("真字符串")) -> (0:w600:string)  [unwired: 1 in]
            n253 = Build Array (concatenate)(w609, w596, w600) -> (w607:string[])
            n254 = Flatten To XML(anything=w607) -> (xml string=w606:string)
            n255 = call "AMC Send Local Message.vi"("Process (\"\" - local)"=w608, "Message Value"=w606, "Message Name"=w608) -> ()  [unwired: 7 in, 2 out]
          }
        }
        n256 = call <vilib>:"Space Constant.vi"() -> ("String"=w588:string)
        n257 = Concatenate Strings(w585, w588, w587) -> (w589:string)
        n258 = call "LogStatus.vi"("error in (no error)"=w582, "last message"=w590, "message"=w589) -> ("error  out"=w591:errorcluster)  [unwired: 8 in]
      }
      frame "5.2.3_19 Check Test item RBdeltaE result" {
        n259 = Unbundle By Name(w612) -> ("Table"=w617:string[][])
        n260 = call "Select_Table_Vaule Enable_Disable.vi"("Action"=w616, "Table"=w617) -> ("Enable"=w615:bool)  [unwired: 8 in, 1 out]
        n261 = case shown="True" w615 {
          tunnel: ["Skip" ("response") w627] -> w618
          tunnel: w617 -> [_ w633]
          tunnel: w616 -> [_ w632]
          tunnel: [_ w625] -> w613
          tunnel: w610 -> [_ w628]
          frame False {
          }
          frame True {
            w639 = "UIdisplay" ("Process (\"\" - local)")
            n262 = Unbundle By Name(w628) -> ("Start Test mode"=w629:string)
            n263 = call "SendCmd.vi"("cmd"=w629, "exe"="D:\\Program Files\\MVTec\\HALCON-17.12-Progress\\bin\\x64-win64\\hdevelop.exe") -> ("error out"=w626:errorcluster, "standard output"=w627:string)  [unwired: 6 in, 2 out]
            n264 = call <vilib>:"Clear Errors.vi"("error in (no error)"=w626) -> ("error out"=w625:errorcluster)  [unwired: 5 in, 1 out]
            n265 = call "Select_Table_Vaule.vi"("Vaule"=w627, "Action"=w632, "Table"=w633) -> ("Result"=w634:bool, "vaule"=w640:string[])  [unwired: 7 in]
            n266 = Append True/False String(1:w634, 2:"FAIL" ("真字符串"), 3:"PASS" ("真字符串")) -> (0:w631:string)  [unwired: 1 in]
            n267 = Build Array (concatenate)(w640, w627, w631) -> (w638:string[])
            n268 = Flatten To XML(anything=w638) -> (xml string=w637:string)
            n269 = call "AMC Send Local Message.vi"("Process (\"\" - local)"=w639, "Message Value"=w637, "Message Name"=w639) -> ()  [unwired: 7 in, 2 out]
          }
        }
        n270 = call <vilib>:"Space Constant.vi"() -> ("String"=w619:string)
        n271 = Concatenate Strings(w616, w619, w618) -> (w620:string)
        n272 = call "LogStatus.vi"("error in (no error)"=w613, "last message"=w621, "message"=w620) -> ("error  out"=w622:errorcluster)  [unwired: 8 in]
      }
      frame "5.2.3_20 Check Test item BWdeltaE result" {
        n273 = Unbundle By Name(w643) -> ("Table"=w648:string[][])
        n274 = call "Select_Table_Vaule Enable_Disable.vi"("Action"=w647, "Table"=w648) -> ("Enable"=w646:bool)  [unwired: 8 in, 1 out]
        n275 = case shown="True" w646 {
          tunnel: ["Skip" ("response") w658] -> w649
          tunnel: w648 -> [_ w664]
          tunnel: w647 -> [_ w663]
          tunnel: [_ w656] -> w644
          tunnel: w641 -> [_ w659]
          frame False {
          }
          frame True {
            w670 = "UIdisplay" ("Process (\"\" - local)")
            n276 = Unbundle By Name(w659) -> ("Start Test mode"=w660:string)
            n277 = call "SendCmd.vi"("cmd"=w660, "exe"="D:\\Program Files\\MVTec\\HALCON-17.12-Progress\\bin\\x64-win64\\hdevelop.exe") -> ("error out"=w657:errorcluster, "standard output"=w658:string)  [unwired: 6 in, 2 out]
            n278 = call <vilib>:"Clear Errors.vi"("error in (no error)"=w657) -> ("error out"=w656:errorcluster)  [unwired: 5 in, 1 out]
            n279 = call "Select_Table_Vaule.vi"("Vaule"=w658, "Action"=w663, "Table"=w664) -> ("Result"=w665:bool, "vaule"=w671:string[])  [unwired: 7 in]
            n280 = Append True/False String(1:w665, 2:"FAIL" ("真字符串"), 3:"PASS" ("真字符串")) -> (0:w662:string)  [unwired: 1 in]
            n281 = Build Array (concatenate)(w671, w658, w662) -> (w669:string[])
            n282 = Flatten To XML(anything=w669) -> (xml string=w668:string)
            n283 = call "AMC Send Local Message.vi"("Process (\"\" - local)"=w670, "Message Value"=w668, "Message Name"=w670) -> ()  [unwired: 7 in, 2 out]
          }
        }
        n284 = call <vilib>:"Space Constant.vi"() -> ("String"=w650:string)
        n285 = Concatenate Strings(w647, w650, w649) -> (w651:string)
        n286 = call "LogStatus.vi"("error in (no error)"=w644, "last message"=w652, "message"=w651) -> ("error  out"=w653:errorcluster)  [unwired: 8 in]
      }
      frame "5.2.3_21 Check Test item WRdeltaE result" {
        # "Disconnect_UUT"
        n287 = Unbundle By Name(w674) -> ("Table"=w679:string[][])
        n288 = call "Select_Table_Vaule Enable_Disable.vi"("Action"=w678, "Table"=w679) -> ("Enable"=w677:bool)  [unwired: 8 in, 1 out]
        n289 = case shown="True" w677 {
          tunnel: ["Skip" ("response") w689] -> w680
          tunnel: w679 -> [_ w695]
          tunnel: w678 -> [_ w694]
          tunnel: [_ w687] -> w675
          tunnel: w672 -> [_ w690]
          frame False {
          }
          frame True {
            w701 = "UIdisplay" ("Process (\"\" - local)")
            n290 = Unbundle By Name(w690) -> ("Start Test mode"=w691:string)
            n291 = call "SendCmd.vi"("cmd"=w691, "exe"="D:\\Program Files\\MVTec\\HALCON-17.12-Progress\\bin\\x64-win64\\hdevelop.exe") -> ("error out"=w688:errorcluster, "standard output"=w689:string)  [unwired: 6 in, 2 out]
            n292 = call <vilib>:"Clear Errors.vi"("error in (no error)"=w688) -> ("error out"=w687:errorcluster)  [unwired: 5 in, 1 out]
            n293 = call "Select_Table_Vaule.vi"("Vaule"=w689, "Action"=w694, "Table"=w695) -> ("Result"=w696:bool, "vaule"=w702:string[])  [unwired: 7 in]
            n294 = Append True/False String(1:w696, 2:"FAIL" ("真字符串"), 3:"PASS" ("真字符串")) -> (0:w693:string)  [unwired: 1 in]
            n295 = Build Array (concatenate)(w702, w689, w693) -> (w700:string[])
            n296 = Flatten To XML(anything=w700) -> (xml string=w699:string)
            n297 = call "AMC Send Local Message.vi"("Process (\"\" - local)"=w701, "Message Value"=w699, "Message Name"=w701) -> ()  [unwired: 7 in, 2 out]
          }
        }
        n298 = call <vilib>:"Space Constant.vi"() -> ("String"=w681:string)
        n299 = Concatenate Strings(w678, w681, w680) -> (w682:string)
        n300 = call "LogStatus.vi"("error in (no error)"=w675, "last message"=w683, "message"=w682) -> ("error  out"=w684:errorcluster)  [unwired: 8 in]
      }
      frame "5.2.3_22 Check Test item deltaa result" {
        # "Disconnect_UUT"
        n301 = Unbundle By Name(w705) -> ("Table"=w710:string[][])
        n302 = call "Select_Table_Vaule Enable_Disable.vi"("Action"=w709, "Table"=w710) -> ("Enable"=w708:bool)  [unwired: 8 in, 1 out]
        n303 = case shown="True" w708 {
          tunnel: ["Skip" ("response") w720] -> w711
          tunnel: w710 -> [_ w726]
          tunnel: w709 -> [_ w725]
          tunnel: [_ w718] -> w706
          tunnel: w703 -> [_ w721]
          frame False {
          }
          frame True {
            w732 = "UIdisplay" ("Process (\"\" - local)")
            n304 = Unbundle By Name(w721) -> ("Start Test mode"=w722:string)
            n305 = call "SendCmd.vi"("cmd"=w722, "exe"="D:\\Program Files\\MVTec\\HALCON-17.12-Progress\\bin\\x64-win64\\hdevelop.exe") -> ("error out"=w719:errorcluster, "standard output"=w720:string)  [unwired: 6 in, 2 out]
            n306 = call <vilib>:"Clear Errors.vi"("error in (no error)"=w719) -> ("error out"=w718:errorcluster)  [unwired: 5 in, 1 out]
            n307 = call "Select_Table_Vaule.vi"("Vaule"=w720, "Action"=w725, "Table"=w726) -> ("Result"=w727:bool, "vaule"=w733:string[])  [unwired: 7 in]
            n308 = Append True/False String(1:w727, 2:"FAIL" ("真字符串"), 3:"PASS" ("真字符串")) -> (0:w724:string)  [unwired: 1 in]
            n309 = Build Array (concatenate)(w733, w720, w724) -> (w731:string[])
            n310 = Flatten To XML(anything=w731) -> (xml string=w730:string)
            n311 = call "AMC Send Local Message.vi"("Process (\"\" - local)"=w732, "Message Value"=w730, "Message Name"=w732) -> ()  [unwired: 7 in, 2 out]
          }
        }
        n312 = call <vilib>:"Space Constant.vi"() -> ("String"=w712:string)
        n313 = Concatenate Strings(w709, w712, w711) -> (w713:string)
        n314 = call "LogStatus.vi"("error in (no error)"=w706, "last message"=w714, "message"=w713) -> ("error  out"=w715:errorcluster)  [unwired: 8 in]
      }
      frame "5.2.3_23 Check Test item deltab result" {
        # "Disconnect_UUT"
        n315 = Unbundle By Name(w736) -> ("Table"=w741:string[][])
        n316 = call "Select_Table_Vaule Enable_Disable.vi"("Action"=w740, "Table"=w741) -> ("Enable"=w739:bool)  [unwired: 8 in, 1 out]
        n317 = case shown="True" w739 {
          tunnel: ["Skip" ("response") w751] -> w742
          tunnel: w741 -> [_ w757]
          tunnel: w740 -> [_ w756]
          tunnel: [_ w749] -> w737
          tunnel: w734 -> [_ w752]
          frame False {
          }
          frame True {
            w763 = "UIdisplay" ("Process (\"\" - local)")
            n318 = Unbundle By Name(w752) -> ("Start Test mode"=w753:string)
            n319 = call "SendCmd.vi"("cmd"=w753, "exe"="D:\\Program Files\\MVTec\\HALCON-17.12-Progress\\bin\\x64-win64\\hdevelop.exe") -> ("error out"=w750:errorcluster, "standard output"=w751:string)  [unwired: 6 in, 2 out]
            n320 = call <vilib>:"Clear Errors.vi"("error in (no error)"=w750) -> ("error out"=w749:errorcluster)  [unwired: 5 in, 1 out]
            n321 = call "Select_Table_Vaule.vi"("Vaule"=w751, "Action"=w756, "Table"=w757) -> ("Result"=w758:bool, "vaule"=w764:string[])  [unwired: 7 in]
            n322 = Append True/False String(1:w758, 2:"FAIL" ("真字符串"), 3:"PASS" ("真字符串")) -> (0:w755:string)  [unwired: 1 in]
            n323 = Build Array (concatenate)(w764, w751, w755) -> (w762:string[])
            n324 = Flatten To XML(anything=w762) -> (xml string=w761:string)
            n325 = call "AMC Send Local Message.vi"("Process (\"\" - local)"=w763, "Message Value"=w761, "Message Name"=w763) -> ()  [unwired: 7 in, 2 out]
          }
        }
        n326 = call <vilib>:"Space Constant.vi"() -> ("String"=w743:string)
        n327 = Concatenate Strings(w740, w743, w742) -> (w744:string)
        n328 = call "LogStatus.vi"("error in (no error)"=w737, "last message"=w745, "message"=w744) -> ("error  out"=w746:errorcluster)  [unwired: 8 in]
      }
      frame "5.2.3_24 Color Check Results" {
        # "Disconnect_UUT"
        n329 = Unbundle By Name(w767) -> ("Table"=w772:string[][])
        n330 = call "Select_Table_Vaule Enable_Disable.vi"("Action"=w771, "Table"=w772) -> ("Enable"=w770:bool)  [unwired: 8 in, 1 out]
        n331 = case shown="True" w770 {
          tunnel: ["Skip" ("response") w782] -> w773
          tunnel: w772 -> [_ w788]
          tunnel: w771 -> [_ w787]
          tunnel: [_ w780] -> w768
          tunnel: w765 -> [_ w783]
          frame False {
          }
          frame True {
            w794 = "UIdisplay" ("Process (\"\" - local)")
            n332 = Unbundle By Name(w783) -> ("Start Test mode"=w784:string)
            n333 = call "SendCmd.vi"("cmd"=w784, "exe"="D:\\Program Files\\MVTec\\HALCON-17.12-Progress\\bin\\x64-win64\\hdevelop.exe") -> ("error out"=w781:errorcluster, "standard output"=w782:string)  [unwired: 6 in, 2 out]
            n334 = call <vilib>:"Clear Errors.vi"("error in (no error)"=w781) -> ("error out"=w780:errorcluster)  [unwired: 5 in, 1 out]
            n335 = call "Select_Table_Vaule.vi"("Vaule"=w782, "Action"=w787, "Table"=w788) -> ("Result"=w789:bool, "vaule"=w795:string[])  [unwired: 7 in]
            n336 = Append True/False String(1:w789, 2:"FAIL" ("真字符串"), 3:"PASS" ("真字符串")) -> (0:w786:string)  [unwired: 1 in]
            n337 = Build Array (concatenate)(w795, w782, w786) -> (w793:string[])
            n338 = Flatten To XML(anything=w793) -> (xml string=w792:string)
            n339 = call "AMC Send Local Message.vi"("Process (\"\" - local)"=w794, "Message Value"=w792, "Message Name"=w794) -> ()  [unwired: 7 in, 2 out]
          }
        }
        n340 = call <vilib>:"Space Constant.vi"() -> ("String"=w774:string)
        n341 = Concatenate Strings(w771, w774, w773) -> (w775:string)
        n342 = call "LogStatus.vi"("error in (no error)"=w768, "last message"=w776, "message"=w775) -> ("error  out"=w777:errorcluster)  [unwired: 8 in]
      }
      frame "5.2.3_25 Stop Camera" {
        # "Disconnect_UUT"
        n343 = Unbundle By Name(w798) -> ("Table"=w803:string[][])
        n344 = call "Select_Table_Vaule Enable_Disable.vi"("Action"=w802, "Table"=w803) -> ("Enable"=w801:bool)  [unwired: 8 in, 1 out]
        n345 = case shown="True" w801 {
          tunnel: ["Skip" ("response") w813] -> w804
          tunnel: w803 -> [_ w819]
          tunnel: w802 -> [_ w818]
          tunnel: [_ w811] -> w799
          tunnel: w796 -> [_ w814]
          frame False {
          }
          frame True {
            w825 = "UIdisplay" ("Process (\"\" - local)")
            n346 = Unbundle By Name(w814) -> ("Start Test mode"=w815:string)
            n347 = call "SendCmd.vi"("cmd"=w815, "exe"="D:\\Program Files\\MVTec\\HALCON-17.12-Progress\\bin\\x64-win64\\hdevelop.exe") -> ("error out"=w812:errorcluster, "standard output"=w813:string)  [unwired: 6 in, 2 out]
            n348 = call <vilib>:"Clear Errors.vi"("error in (no error)"=w812) -> ("error out"=w811:errorcluster)  [unwired: 5 in, 1 out]
            n349 = call "Select_Table_Vaule.vi"("Vaule"=w813, "Action"=w818, "Table"=w819) -> ("Result"=w820:bool, "vaule"=w826:string[])  [unwired: 7 in]
            n350 = Append True/False String(1:w820, 2:"FAIL" ("真字符串"), 3:"PASS" ("真字符串")) -> (0:w817:string)  [unwired: 1 in]
            n351 = Build Array (concatenate)(w826, w813, w817) -> (w824:string[])
            n352 = Flatten To XML(anything=w824) -> (xml string=w823:string)
            n353 = call "AMC Send Local Message.vi"("Process (\"\" - local)"=w825, "Message Value"=w823, "Message Name"=w825) -> ()  [unwired: 7 in, 2 out]
          }
        }
        n354 = call <vilib>:"Space Constant.vi"() -> ("String"=w805:string)
        n355 = Concatenate Strings(w802, w805, w804) -> (w806:string)
        n356 = call "LogStatus.vi"("error in (no error)"=w799, "last message"=w807, "message"=w806) -> ("error  out"=w808:errorcluster)  [unwired: 8 in]
      }
      frame "5.2.3_26 Stop Test mode" {
        # "Disconnect_UUT"
        n357 = Unbundle By Name(w829) -> ("Table"=w834:string[][])
        n358 = call "Select_Table_Vaule Enable_Disable.vi"("Action"=w833, "Table"=w834) -> ("Enable"=w832:bool)  [unwired: 8 in, 1 out]
        n359 = case shown="True" w832 {
          tunnel: ["Skip" ("response") w844] -> w835
          tunnel: w834 -> [_ w850]
          tunnel: w833 -> [_ w849]
          tunnel: [_ w842] -> w830
          tunnel: w827 -> [_ w845]
          frame False {
          }
          frame True {
            w856 = "UIdisplay" ("Process (\"\" - local)")
            n360 = Unbundle By Name(w845) -> ("Start Test mode"=w846:string)
            n361 = call "SendCmd.vi"("cmd"=w846, "exe"="D:\\Program Files\\MVTec\\HALCON-17.12-Progress\\bin\\x64-win64\\hdevelop.exe") -> ("error out"=w843:errorcluster, "standard output"=w844:string)  [unwired: 6 in, 2 out]
            n362 = call <vilib>:"Clear Errors.vi"("error in (no error)"=w843) -> ("error out"=w842:errorcluster)  [unwired: 5 in, 1 out]
            n363 = call "Select_Table_Vaule.vi"("Vaule"=w844, "Action"=w849, "Table"=w850) -> ("Result"=w851:bool, "vaule"=w857:string[])  [unwired: 7 in]
            n364 = Append True/False String(1:w851, 2:"FAIL" ("真字符串"), 3:"PASS" ("真字符串")) -> (0:w848:string)  [unwired: 1 in]
            n365 = Build Array (concatenate)(w857, w844, w848) -> (w855:string[])
            n366 = Flatten To XML(anything=w855) -> (xml string=w854:string)
            n367 = call "AMC Send Local Message.vi"("Process (\"\" - local)"=w856, "Message Value"=w854, "Message Name"=w856) -> ()  [unwired: 7 in, 2 out]
          }
        }
        n368 = call <vilib>:"Space Constant.vi"() -> ("String"=w836:string)
        n369 = Concatenate Strings(w833, w836, w835) -> (w837:string)
        n370 = call "LogStatus.vi"("error in (no error)"=w830, "last message"=w838, "message"=w837) -> ("error  out"=w839:errorcluster)  [unwired: 8 in]
      }
      frame "5.2.3_27 Shutdown UUT" {
        # "Disconnect_UUT"
        n371 = Unbundle By Name(w861) -> ("Table"=w866:string[][])
        n372 = call "Select_Table_Vaule Enable_Disable.vi"("Action"=w865, "Table"=w866) -> ("Enable"=w864:bool)  [unwired: 8 in, 1 out]
        n373 = case shown="True" w864 {
          tunnel: ["Skip" ("response") w876] -> w867
          tunnel: w866 -> [_ w882]
          tunnel: w865 -> [_ w881]
          tunnel: [_ w874] -> w862
          tunnel: w859 -> [_ w877]
          frame False {
          }
          frame True {
            w888 = "UIdisplay" ("Process (\"\" - local)")
            n374 = Unbundle By Name(w877) -> ("Start Test mode"=w878:string)
            n375 = call "SendCmd.vi"("cmd"=w878, "exe"="D:\\Program Files\\MVTec\\HALCON-17.12-Progress\\bin\\x64-win64\\hdevelop.exe") -> ("error out"=w875:errorcluster, "standard output"=w876:string)  [unwired: 6 in, 2 out]
            n376 = call <vilib>:"Clear Errors.vi"("error in (no error)"=w875) -> ("error out"=w874:errorcluster)  [unwired: 5 in, 1 out]
            n377 = call "Select_Table_Vaule.vi"("Vaule"=w876, "Action"=w881, "Table"=w882) -> ("Result"=w883:bool, "vaule"=w889:string[])  [unwired: 7 in]
            n378 = Append True/False String(1:w883, 2:"FAIL" ("真字符串"), 3:"PASS" ("真字符串")) -> (0:w880:string)  [unwired: 1 in]
            n379 = Build Array (concatenate)(w889, w876, w880) -> (w887:string[])
            n380 = Flatten To XML(anything=w887) -> (xml string=w886:string)
            n381 = call "AMC Send Local Message.vi"("Process (\"\" - local)"=w888, "Message Value"=w886, "Message Name"=w888) -> ()  [unwired: 7 in, 2 out]
          }
        }
        n382 = call <vilib>:"Space Constant.vi"() -> ("String"=w868:string)
        n383 = Concatenate Strings(w865, w868, w867) -> (w869:string)
        n384 = call "LogStatus.vi"("error in (no error)"=w862, "last message"=w870, "message"=w869) -> ("error  out"=w871:errorcluster)  [unwired: 8 in]
      }
      frame "Check Environment value" {
        n385 = Unbundle By Name(w890) -> ("Table"=w897:string[][])
        n386 = call "Select_Table_Vaule Enable_Disable.vi"("Action"=w896, "Table"=w897) -> ("Enable"=w895:bool)  [unwired: 8 in, 1 out]
        n387 = case shown="True" w895 {
          tunnel: ["Skip" ("response") w922] -> w898
          tunnel: w897 -> [_ w927]
          tunnel: w896 -> [_ w926]
          tunnel: [_ w918] -> w891
          frame False {
          }
          frame True {
            w917 = errorcluster {"status"=FALSE, "code"=0, "source"=""} ("错误输入（无错误）")
            w933 = "UIdisplay" ("Process (\"\" - local)")
            # "humidity"
            # "temperature"
            # "Ambient Temperature"
            n388 = call "I2C_read.vi"("错误输入（无错误）"=w917) -> ("readSucess"=w923:bool, "Led"=w924:string, "错误输出"=w918:errorcluster)  [unwired: 7 in, 1 out]
            n389 = call "HD_Config.vi"("error in (no error)"=w917, "Step"=enum16{"Initial", "Write", "Read"}."Read") -> ("HD Config out"=w920:T7)  [unwired: 8 in, 1 out]
            n390 = Unbundle By Name(w920) -> ("Tempt&Hum.COM"=w921:refnum<visa-resource-name>)
            n391 = call "ADAM_Read.vi"("VISA resource name"=w921) -> ("humidity"=w912:dbl, "temperature"=w911:dbl)  [unwired: 7 in, 2 out]
            n392 = In Range and Coerce(upper limit=30 ("y"), x=w911, lower limit=20 ("y")) -> (In Range?=w910:bool)  [unwired: 1 out]
            n393 = In Range and Coerce(upper limit=70 ("y"), x=w912, lower limit=30 ("y")) -> (In Range?=w909:bool)  [unwired: 1 out]
            n394 = And(x=w910, y=w909) -> (x .and. y?=w908:bool)
            n395 = case shown="True" w923 {
              tunnel: w924 -> [_ w945]
              tunnel: ["Error:  Read Environment Illuminance Value Fail" w940] -> w922
              tunnel: w908 -> [_ w937]
              frame False {
              }
              frame True {
                n396 = Decimal String To Number(string=w945) -> (number=w939:i32)  [unwired: 2 in, 1 out]
                n397 = Greater?(x=w939, y=0) -> (0:w942:bool)
                n398 = Less?(x=w939, y=5) -> (x < y?=w941:bool)
                n399 = And(x=w942, y=w941) -> (x .and. y?=w938:bool)
                n400 = And(x=w938, y=w937) -> (x .and. y?=w936:bool)
                n401 = case shown="True" w936 {
                  tunnel: ["Error: Luminance value out of range" "Read Environment Illuminance Value Success"] -> w940
                  frame False {
                  }
                  frame True {
                  }
                }
              }
            }
            n402 = call "Select_Table_Vaule.vi"("Vaule"=w922, "Action"=w926, "Table"=w927) -> ("Result"=w928:bool, "vaule"=w934:string[])  [unwired: 7 in]
            n403 = Append True/False String(1:w928, 2:"FAIL" ("真字符串"), 3:"PASS" ("真字符串")) -> (0:w925:string)  [unwired: 1 in]
            n404 = Build Array (concatenate)(w934, w922, w925) -> (w932:string[])
            n405 = Flatten To XML(anything=w932) -> (xml string=w931:string)
            n406 = call "AMC Send Local Message.vi"("Process (\"\" - local)"=w933, "Message Value"=w931, "Message Name"=w933) -> ()  [unwired: 7 in, 2 out]
          }
        }
        n407 = call <vilib>:"Space Constant.vi"() -> ("String"=w899:string)
        n408 = Concatenate Strings(w896, w899, w898) -> (w900:string)
        n409 = call "LogStatus.vi"("error in (no error)"=w891, "last message"=w902, "message"=w900) -> ("error  out"=w903:errorcluster)  [unwired: 8 in]
        n410 = case shown="Error" w891 {
          tunnel: [_ TRUE] -> w893
          tunnel: [_ "Error"] -> w894
          frame No Error {
          }
          frame Error {
          }
        }
      }
      frame "Start Test mode" {
        n411 = Unbundle By Name(w949) -> ("Table"=w956:string[][])
        n412 = call "Select_Table_Vaule Enable_Disable.vi"("Action"=w955, "Table"=w956) -> ("Enable"=w954:bool)  [unwired: 8 in, 1 out]
        n413 = case shown="True" w954 {
          tunnel: ["Skip" ("response") w970] -> w957
          tunnel: w956 -> [_ w978]
          tunnel: w955 -> [_ w977]
          tunnel: [_ w969] -> w950
          tunnel: w948 -> [_ w967]
          frame False {
          }
          frame True {
            w984 = "UIdisplay" ("Process (\"\" - local)")
            n414 = Unbundle By Name(w967) -> ("Start Test mode"=w975:string)
            n415 = call "SendCmd.vi"("cmd"=w975, "exe"="D:\\Program Files\\MVTec\\HALCON-17.12-Progress\\bin\\x64-win64\\hdevelop.exe") -> ("error out"=w969:errorcluster, "standard output"=w972:string, "return code"=w973:i32, "standard error"=w971:string)  [unwired: 6 in]
            n416 = Equal To 0?(x=w973) -> (x = 0?=w974:bool)
            n417 = case shown="False" w974 {
              tunnel: w972 -> [_ w987]
              tunnel: [w986 w987] -> w970
              tunnel: w971 -> [w986 _]
              frame False {
              }
              frame True {
              }
            }
            n418 = call "Select_Table_Vaule.vi"("Vaule"=w970, "Action"=w977, "Table"=w978) -> ("Result"=w979:bool, "vaule"=w985:string[])  [unwired: 7 in]
            n419 = Append True/False String(1:w979, 2:"FAIL" ("真字符串"), 3:"PASS" ("真字符串")) -> (0:w976:string)  [unwired: 1 in]
            n420 = Build Array (concatenate)(w985, w970, w976) -> (w983:string[])
            n421 = Flatten To XML(anything=w983) -> (xml string=w982:string)
            n422 = call "AMC Send Local Message.vi"("Process (\"\" - local)"=w984, "Message Value"=w982, "Message Name"=w984) -> ()  [unwired: 7 in, 2 out]
          }
        }
        n423 = call <vilib>:"Space Constant.vi"() -> ("String"=w958:string)
        n424 = Concatenate Strings(w955, w958, w957) -> (w959:string)
        n425 = call "LogStatus.vi"("error in (no error)"=w950, "last message"=w961, "message"=w959) -> ("error  out"=w962:errorcluster)  [unwired: 8 in]
        n426 = case shown="Error" w950 {
          tunnel: [_ TRUE] -> w952
          tunnel: [_ "Error"] -> w953
          frame No Error {
          }
          frame Error {
          }
        }
      }
      frame "Start camera test mode" {
        n427 = Unbundle By Name(w989) -> ("Table"=w996:string[][])
        n428 = call "Select_Table_Vaule Enable_Disable.vi"("Action"=w995, "Table"=w996) -> ("Enable"=w994:bool)  [unwired: 8 in, 1 out]
        n429 = case shown="True" w994 {
          tunnel: ["Skip" ("response") w1009] -> w997
          tunnel: w996 -> [_ w1018]
          tunnel: w995 -> [_ w1017]
          tunnel: [_ w1008] -> w990
          tunnel: w988 -> [_ w1007]
          frame False {
          }
          frame True {
            w1024 = "UIdisplay" ("Process (\"\" - local)")
            n430 = Unbundle By Name(w1007) -> ("Start camera test mode P1"=w1015:string)
            n431 = call "SendCmd.vi"("cmd"=w1015, "exe"="D:\\Program Files\\MVTec\\HALCON-17.12-Progress\\bin\\x64-win64\\hdevelop.exe") -> ("error out"=w1008:errorcluster, "standard output"=w1011:string, "return code"=w1012:i32, "standard error"=w1010:string)  [unwired: 6 in]
            n432 = Equal To 0?(x=w1012) -> (x = 0?=w1013:bool)
            n433 = case shown="False" w1013 {
              tunnel: w1011 -> [_ w1027]
              tunnel: [w1026 w1027] -> w1009
              tunnel: w1010 -> [w1026 _]
              frame False {
              }
              frame True {
              }
            }
            n434 = call "Select_Table_Vaule.vi"("Vaule"=w1009, "Action"=w1017, "Table"=w1018) -> ("Result"=w1019:bool, "vaule"=w1025:string[])  [unwired: 7 in]
            n435 = Append True/False String(1:w1019, 2:"FAIL" ("真字符串"), 3:"PASS" ("真字符串")) -> (0:w1016:string)  [unwired: 1 in]
            n436 = Build Array (concatenate)(w1025, w1009, w1016) -> (w1023:string[])
            n437 = Flatten To XML(anything=w1023) -> (xml string=w1022:string)
            n438 = call "AMC Send Local Message.vi"("Process (\"\" - local)"=w1024, "Message Value"=w1022, "Message Name"=w1024) -> ()  [unwired: 7 in, 2 out]
          }
        }
        n439 = call <vilib>:"Space Constant.vi"() -> ("String"=w998:string)
        n440 = Concatenate Strings(w995, w998, w997) -> (w999:string)
        n441 = call "LogStatus.vi"("error in (no error)"=w990, "last message"=w1001, "message"=w999) -> ("error  out"=w1002:errorcluster)  [unwired: 8 in]
        n442 = case shown="Error" w990 {
          tunnel: [_ TRUE] -> w992
          tunnel: [_ "Error"] -> w993
          frame No Error {
          }
          frame Error {
          }
        }
      }
      frame "Open VLC for video stream setting" {
        n443 = Unbundle By Name(w1029) -> ("Table"=w1036:string[][])
        n444 = call "Select_Table_Vaule Enable_Disable.vi"("Action"=w1035, "Table"=w1036) -> ("Enable"=w1034:bool)  [unwired: 8 in, 1 out]
        n445 = case shown="True" w1034 {
          tunnel: ["Skip" ("response") w1048] -> w1037
          tunnel: w1036 -> [_ w1056]
          tunnel: w1035 -> [_ w1055]
          tunnel: [_ w1047] -> w1030
          tunnel: w1028 -> [_ _]
          frame False {
          }
          frame True {
            w1062 = "UIdisplay" ("Process (\"\" - local)")
            # "这部分 不确定\"Open VLC for video stream setting\""
            n446 = call "SendCmd.vi"("exe"="D:\\Program Files\\MVTec\\HALCON-17.12-Progress\\bin\\x64-win64\\hdevelop.exe") -> ("error out"=w1047:errorcluster, "standard output"=w1050:string, "return code"=w1051:i32, "standard error"=w1049:string)  [unwired: 7 in]
            n447 = Equal To 0?(x=w1051) -> (x = 0?=w1052:bool)
            n448 = case shown="False" w1052 {
              tunnel: w1050 -> [_ w1065]
              tunnel: [w1064 w1065] -> w1048
              tunnel: w1049 -> [w1064 _]
              frame False {
              }
              frame True {
              }
            }
            n449 = call "Select_Table_Vaule.vi"("Vaule"=w1048, "Action"=w1055, "Table"=w1056) -> ("Result"=w1057:bool, "vaule"=w1063:string[])  [unwired: 7 in]
            n450 = Append True/False String(1:w1057, 2:"FAIL" ("真字符串"), 3:"PASS" ("真字符串")) -> (0:w1054:string)  [unwired: 1 in]
            n451 = Build Array (concatenate)(w1063, w1048, w1054) -> (w1061:string[])
            n452 = Flatten To XML(anything=w1061) -> (xml string=w1060:string)
            n453 = call "AMC Send Local Message.vi"("Process (\"\" - local)"=w1062, "Message Value"=w1060, "Message Name"=w1062) -> ()  [unwired: 7 in, 2 out]
          }
        }
        n454 = call <vilib>:"Space Constant.vi"() -> ("String"=w1038:string)
        n455 = Concatenate Strings(w1035, w1038, w1037) -> (w1039:string)
        n456 = call "LogStatus.vi"("error in (no error)"=w1030, "last message"=w1041, "message"=w1039) -> ("error  out"=w1042:errorcluster)  [unwired: 8 in]
        n457 = case shown="Error" w1030 {
          tunnel: [_ TRUE] -> w1032
          tunnel: [_ "Error"] -> w1033
          frame No Error {
          }
          frame Error {
          }
        }
      }
      frame "Adjust motor to alignment ROI overlay" {
        n458 = Unbundle By Name(w1067) -> ("Table"=w1074:string[][])
        n459 = call "Select_Table_Vaule Enable_Disable.vi"("Action"=w1073, "Table"=w1074) -> ("Enable"=w1072:bool)  [unwired: 8 in, 1 out]
        n460 = case shown="True" w1072 {
          tunnel: ["Skip" ("response") w1102] -> w1075
          tunnel: w1074 -> [_ w1105]
          tunnel: w1073 -> [_ w1104]
          tunnel: [_ w1087] -> w1068
          tunnel: w1066 -> [_ _]
          frame False {
          }
          frame True {
            w1111 = "UIdisplay" ("Process (\"\" - local)")
            n461 = call "HD_Config.vi"("Step"=enum16{"Initial", "Write", "Read"}."Read") -> ("error out"=w1092:errorcluster, "HD Config out"=w1100:T7)  [unwired: 9 in]
            n462 = Unbundle By Name(w1100) -> ("Motor.COM"=w1099:refnum<visa-resource-name>)  [unwired: 1 out]
            n463 = call "MotorMoveAbsPos.vi"("error in (no error)"=w1092, "Chan Ident"="1", "absolute position/mm"="absolute position/mm 2", "VISA资源名称"=w1099) -> ("error out"=w1090:errorcluster, "MoveCOMPLETE"=w1095:bool)  [unwired: 5 in]
            n464 = call "MotorMoveAbsPos.vi"("error in (no error)"=w1090, "Chan Ident"="1", "absolute position/mm"="absolute position/mm 2", "VISA资源名称"=w1099) -> ("error out"=w1089:errorcluster, "MoveCOMPLETE"=w1094:bool)  [unwired: 5 in]
            n465 = call "MotorMoveAbsPos.vi"("error in (no error)"=w1089, "Chan Ident"="1", "absolute position/mm"="absolute position/mm 2", "VISA资源名称"=w1099) -> ("error out"=w1087:errorcluster, "MoveCOMPLETE"=w1093:bool)  [unwired: 5 in]
            n466 = Compound Arithmetic op=AND ("复合运算")(w1095, w1094, w1093) -> (w1091:bool)
            n467 = case shown="True" w1091 {
              tunnel: "Adjust the XY-axis and Z-axis linear stage success" ("standard error") -> [_ w1114]
              tunnel: [w1113 w1114] -> w1102
              tunnel: "Adjust the XY-axis and Z-axis linear stage fail" ("standard error") -> [w1113 _]
              frame False {
              }
              frame True {
              }
            }
            n468 = call "Select_Table_Vaule.vi"("Vaule"=w1102, "Action"=w1104, "Table"=w1105) -> ("Result"=w1106:bool, "vaule"=w1112:string[])  [unwired: 7 in]
            n469 = Append True/False String(1:w1106, 2:"FAIL" ("真字符串"), 3:"PASS" ("真字符串")) -> (0:w1103:string)  [unwired: 1 in]
            n470 = Build Array (concatenate)(w1112, w1102, w1103) -> (w1110:string[])
            n471 = Flatten To XML(anything=w1110) -> (xml string=w1109:string)
            n472 = call "AMC Send Local Message.vi"("Process (\"\" - local)"=w1111, "Message Value"=w1109, "Message Name"=w1111) -> ()  [unwired: 7 in, 2 out]
          }
        }
        n473 = call <vilib>:"Space Constant.vi"() -> ("String"=w1076:string)
        n474 = Concatenate Strings(w1073, w1076, w1075) -> (w1077:string)
        n475 = call "LogStatus.vi"("error in (no error)"=w1068, "last message"=w1079, "message"=w1077) -> ("error  out"=w1080:errorcluster)  [unwired: 8 in]
        n476 = case shown="Error" w1068 {
          tunnel: [_ TRUE] -> w1070
          tunnel: [_ "Error"] -> w1071
          frame No Error {
          }
          frame Error {
          }
        }
      }
      frame "Config external Light" {
        n477 = Unbundle By Name(w1116) -> ("Table"=w1123:string[][])
        n478 = call "Select_Table_Vaule Enable_Disable.vi"("Action"=w1122, "Table"=w1123) -> ("Enable"=w1121:bool)  [unwired: 8 in, 1 out]
        n479 = case shown="True" w1121 {
          tunnel: ["Skip" ("response") w1139] -> w1124
          tunnel: w1123 -> [_ w1142]
          tunnel: w1122 -> [_ w1141]
          tunnel: [_ w1135] -> w1117
          tunnel: w1115 -> [_ _]
          frame False {
          }
          frame True {
            w1148 = "UIdisplay" ("Process (\"\" - local)")
            # "Config external Light"
            n480 = call "SendCmd.vi"() -> ("error out"=w1135:errorcluster, "standard output"=w1136:string, "return code"=w1138:i32, "standard error"=w1137:string)  [unwired: 8 in]
            n481 = Equal To 0?(x=w1138) -> (x = 0?=w1134:bool)
            n482 = case shown="True" w1134 {
              tunnel: w1136 -> [_ w1151]
              tunnel: [w1150 w1151] -> w1139
              tunnel: w1137 -> [w1150 _]
              frame False {
              }
              frame True {
              }
            }
            n483 = call "Select_Table_Vaule.vi"("Vaule"=w1139, "Action"=w1141, "Table"=w1142) -> ("Result"=w1143:bool, "vaule"=w1149:string[])  [unwired: 7 in]
            n484 = Append True/False String(1:w1143, 2:"FAIL" ("真字符串"), 3:"PASS" ("真字符串")) -> (0:w1140:string)  [unwired: 1 in]
            n485 = Build Array (concatenate)(w1149, w1139, w1140) -> (w1147:string[])
            n486 = Flatten To XML(anything=w1147) -> (xml string=w1146:string)
            n487 = call "AMC Send Local Message.vi"("Process (\"\" - local)"=w1148, "Message Value"=w1146, "Message Name"=w1148) -> ()  [unwired: 7 in, 2 out]
          }
        }
        n488 = call <vilib>:"Space Constant.vi"() -> ("String"=w1125:string)
        n489 = Concatenate Strings(w1122, w1125, w1124) -> (w1126:string)
        n490 = call "LogStatus.vi"("error in (no error)"=w1117, "last message"=w1128, "message"=w1126) -> ("error  out"=w1129:errorcluster)  [unwired: 8 in]
        n491 = case shown="Error" w1117 {
          tunnel: [_ TRUE] -> w1119
          tunnel: [_ "Error"] -> w1120
          frame No Error {
          }
          frame Error {
          }
        }
      }
      frame "Creating a Test profiles for camera LED" {
        n492 = Unbundle By Name(w1153) -> ("Table"=w1160:string[][])
        n493 = call "Select_Table_Vaule Enable_Disable.vi"("Action"=w1159, "Table"=w1160) -> ("Enable"=w1158:bool)  [unwired: 8 in, 1 out]
        n494 = case shown="True" w1158 {
          tunnel: ["Skip" ("response") w1176] -> w1161
          tunnel: w1160 -> [_ w1179]
          tunnel: w1159 -> [_ w1178]
          tunnel: [_ w1172] -> w1154
          tunnel: w1152 -> [_ _]
          frame False {
          }
          frame True {
            w1185 = "UIdisplay" ("Process (\"\" - local)")
            # "Config external Light"
            n495 = call "SendCmd.vi"() -> ("error out"=w1172:errorcluster, "standard output"=w1173:string, "return code"=w1175:i32, "standard error"=w1174:string)  [unwired: 8 in]
            n496 = Equal To 0?(x=w1175) -> (x = 0?=w1171:bool)
            n497 = case shown="True" w1171 {
              tunnel: w1173 -> [_ w1188]
              tunnel: [w1187 w1188] -> w1176
              tunnel: w1174 -> [w1187 _]
              frame False {
              }
              frame True {
              }
            }
            n498 = call "Select_Table_Vaule.vi"("Vaule"=w1176, "Action"=w1178, "Table"=w1179) -> ("Result"=w1180:bool, "vaule"=w1186:string[])  [unwired: 7 in]
            n499 = Append True/False String(1:w1180, 2:"FAIL" ("真字符串"), 3:"PASS" ("真字符串")) -> (0:w1177:string)  [unwired: 1 in]
            n500 = Build Array (concatenate)(w1186, w1176, w1177) -> (w1184:string[])
            n501 = Flatten To XML(anything=w1184) -> (xml string=w1183:string)
            n502 = call "AMC Send Local Message.vi"("Process (\"\" - local)"=w1185, "Message Value"=w1183, "Message Name"=w1185) -> ()  [unwired: 7 in, 2 out]
          }
        }
        n503 = call <vilib>:"Space Constant.vi"() -> ("String"=w1162:string)
        n504 = Concatenate Strings(w1159, w1162, w1161) -> (w1163:string)
        n505 = call "LogStatus.vi"("error in (no error)"=w1154, "last message"=w1165, "message"=w1163) -> ("error  out"=w1166:errorcluster)  [unwired: 8 in]
        n506 = case shown="Error" w1154 {
          tunnel: [_ TRUE] -> w1156
          tunnel: [_ "Error"] -> w1157
          frame No Error {
          }
          frame Error {
          }
        }
      }
      frame "Check Test item “Reflection” result" {
        n507 = Unbundle By Name(w1190) -> ("Table"=w1197:string[][])
        n508 = call "Select_Table_Vaule Enable_Disable.vi"("Action"=w1196, "Table"=w1197) -> ("Enable"=w1195:bool)  [unwired: 8 in, 1 out]
        n509 = case shown="True" w1195 {
          tunnel: ["Skip" ("response") w1213] -> w1198
          tunnel: w1197 -> [_ w1216]
          tunnel: w1196 -> [_ w1215]
          tunnel: [_ w1209] -> w1191
          tunnel: w1189 -> [_ _]
          frame False {
          }
          frame True {
            w1222 = "UIdisplay" ("Process (\"\" - local)")
            # "<1%"
            # "Config external Light"
            n510 = call "SendCmd.vi"() -> ("error out"=w1209:errorcluster, "standard output"=w1210:string, "return code"=w1212:i32, "standard error"=w1211:string)  [unwired: 8 in]
            n511 = Equal To 0?(x=w1212) -> (x = 0?=w1208:bool)
            n512 = case shown="True" w1208 {
              tunnel: w1210 -> [_ w1225]
              tunnel: [w1224 w1225] -> w1213
              tunnel: w1211 -> [w1224 _]
              frame False {
              }
              frame True {
              }
            }
            n513 = call "Select_Table_Vaule.vi"("Vaule"=w1213, "Action"=w1215, "Table"=w1216) -> ("Result"=w1217:bool, "vaule"=w1223:string[])  [unwired: 7 in]
            n514 = Append True/False String(1:w1217, 2:"FAIL" ("真字符串"), 3:"PASS" ("真字符串")) -> (0:w1214:string)  [unwired: 1 in]
            n515 = Build Array (concatenate)(w1223, w1213, w1214) -> (w1221:string[])
            n516 = Flatten To XML(anything=w1221) -> (xml string=w1220:string)
            n517 = call "AMC Send Local Message.vi"("Process (\"\" - local)"=w1222, "Message Value"=w1220, "Message Name"=w1222) -> ()  [unwired: 7 in, 2 out]
          }
        }
        n518 = call <vilib>:"Space Constant.vi"() -> ("String"=w1199:string)
        n519 = Concatenate Strings(w1196, w1199, w1198) -> (w1200:string)
        n520 = call "LogStatus.vi"("error in (no error)"=w1191, "last message"=w1202, "message"=w1200) -> ("error  out"=w1203:errorcluster)  [unwired: 8 in]
        n521 = case shown="Error" w1191 {
          tunnel: [_ TRUE] -> w1193
          tunnel: [_ "Error"] -> w1194
          frame No Error {
          }
          frame Error {
          }
        }
      }
      frame "Check Test item “Uniformatiy mean” result" {
        n522 = Unbundle By Name(w1227) -> ("Table"=w1234:string[][])
        n523 = call "Select_Table_Vaule Enable_Disable.vi"("Action"=w1233, "Table"=w1234) -> ("Enable"=w1232:bool)  [unwired: 8 in, 1 out]
        n524 = case shown="True" w1232 {
          tunnel: ["Skip" ("response") w1250] -> w1235
          tunnel: w1234 -> [_ w1253]
          tunnel: w1233 -> [_ w1252]
          tunnel: [_ w1246] -> w1228
          tunnel: w1226 -> [_ _]
          frame False {
          }
          frame True {
            w1259 = "UIdisplay" ("Process (\"\" - local)")
            # "TBD"
            # "Config external Light"
            n525 = call "SendCmd.vi"() -> ("error out"=w1246:errorcluster, "standard output"=w1247:string, "return code"=w1249:i32, "standard error"=w1248:string)  [unwired: 8 in]
            n526 = Equal To 0?(x=w1249) -> (x = 0?=w1245:bool)
            n527 = case shown="True" w1245 {
              tunnel: w1247 -> [_ w1262]
              tunnel: [w1261 w1262] -> w1250
              tunnel: w1248 -> [w1261 _]
              frame False {
              }
              frame True {
              }
            }
            n528 = call "Select_Table_Vaule.vi"("Vaule"=w1250, "Action"=w1252, "Table"=w1253) -> ("Result"=w1254:bool, "vaule"=w1260:string[])  [unwired: 7 in]
            n529 = Append True/False String(1:w1254, 2:"FAIL" ("真字符串"), 3:"PASS" ("真字符串")) -> (0:w1251:string)  [unwired: 1 in]
            n530 = Build Array (concatenate)(w1260, w1250, w1251) -> (w1258:string[])
            n531 = Flatten To XML(anything=w1258) -> (xml string=w1257:string)
            n532 = call "AMC Send Local Message.vi"("Process (\"\" - local)"=w1259, "Message Value"=w1257, "Message Name"=w1259) -> ()  [unwired: 7 in, 2 out]
          }
        }
        n533 = call <vilib>:"Space Constant.vi"() -> ("String"=w1236:string)
        n534 = Concatenate Strings(w1233, w1236, w1235) -> (w1237:string)
        n535 = call "LogStatus.vi"("error in (no error)"=w1228, "last message"=w1239, "message"=w1237) -> ("error  out"=w1240:errorcluster)  [unwired: 8 in]
        n536 = case shown="Error" w1228 {
          tunnel: [_ TRUE] -> w1230
          tunnel: [_ "Error"] -> w1231
          frame No Error {
          }
          frame Error {
          }
        }
      }
      frame "Check Test item “Uniformity Standard” result" {
        n537 = Unbundle By Name(w1264) -> ("Table"=w1271:string[][])
        n538 = call "Select_Table_Vaule Enable_Disable.vi"("Action"=w1270, "Table"=w1271) -> ("Enable"=w1269:bool)  [unwired: 8 in, 1 out]
        n539 = case shown="True" w1269 {
          tunnel: ["Skip" ("response") w1287] -> w1272
          tunnel: w1271 -> [_ w1290]
          tunnel: w1270 -> [_ w1289]
          tunnel: [_ w1283] -> w1265
          tunnel: w1263 -> [_ _]
          frame False {
          }
          frame True {
            w1296 = "UIdisplay" ("Process (\"\" - local)")
            # "<30"
            # "Config external Light"
            n540 = call "SendCmd.vi"() -> ("error out"=w1283:errorcluster, "standard output"=w1284:string, "return code"=w1286:i32, "standard error"=w1285:string)  [unwired: 8 in]
            n541 = Equal To 0?(x=w1286) -> (x = 0?=w1282:bool)
            n542 = case shown="True" w1282 {
              tunnel: w1284 -> [_ w1299]
              tunnel: [w1298 w1299] -> w1287
              tunnel: w1285 -> [w1298 _]
              frame False {
              }
              frame True {
              }
            }
            n543 = call "Select_Table_Vaule.vi"("Vaule"=w1287, "Action"=w1289, "Table"=w1290) -> ("Result"=w1291:bool, "vaule"=w1297:string[])  [unwired: 7 in]
            n544 = Append True/False String(1:w1291, 2:"FAIL" ("真字符串"), 3:"PASS" ("真字符串")) -> (0:w1288:string)  [unwired: 1 in]
            n545 = Build Array (concatenate)(w1297, w1287, w1288) -> (w1295:string[])
            n546 = Flatten To XML(anything=w1295) -> (xml string=w1294:string)
            n547 = call "AMC Send Local Message.vi"("Process (\"\" - local)"=w1296, "Message Value"=w1294, "Message Name"=w1296) -> ()  [unwired: 7 in, 2 out]
          }
        }
        n548 = call <vilib>:"Space Constant.vi"() -> ("String"=w1273:string)
        n549 = Concatenate Strings(w1270, w1273, w1272) -> (w1274:string)
        n550 = call "LogStatus.vi"("error in (no error)"=w1265, "last message"=w1276, "message"=w1274) -> ("error  out"=w1277:errorcluster)  [unwired: 8 in]
        n551 = case shown="Error" w1265 {
          tunnel: [_ TRUE] -> w1267
          tunnel: [_ "Error"] -> w1268
          frame No Error {
          }
          frame Error {
          }
        }
      }
      frame "Check Test item “Distortation_Center X” result" {
        n552 = Unbundle By Name(w1301) -> ("Table"=w1308:string[][])
        n553 = call "Select_Table_Vaule Enable_Disable.vi"("Action"=w1307, "Table"=w1308) -> ("Enable"=w1306:bool)  [unwired: 8 in, 1 out]
        n554 = case shown="True" w1306 {
          tunnel: ["Skip" ("response") w1324] -> w1309
          tunnel: w1308 -> [_ w1327]
          tunnel: w1307 -> [_ w1326]
          tunnel: [_ w1320] -> w1302
          tunnel: w1300 -> [_ _]
          frame False {
          }
          frame True {
            w1333 = "UIdisplay" ("Process (\"\" - local)")
            # "TBD"
            # "Config external Light"
            n555 = call "SendCmd.vi"() -> ("error out"=w1320:errorcluster, "standard output"=w1321:string, "return code"=w1323:i32, "standard error"=w1322:string)  [unwired: 8 in]
            n556 = Equal To 0?(x=w1323) -> (x = 0?=w1319:bool)
            n557 = case shown="True" w1319 {
              tunnel: w1321 -> [_ w1336]
              tunnel: [w1335 w1336] -> w1324
              tunnel: w1322 -> [w1335 _]
              frame False {
              }
              frame True {
              }
            }
            n558 = call "Select_Table_Vaule.vi"("Vaule"=w1324, "Action"=w1326, "Table"=w1327) -> ("Result"=w1328:bool, "vaule"=w1334:string[])  [unwired: 7 in]
            n559 = Append True/False String(1:w1328, 2:"FAIL" ("真字符串"), 3:"PASS" ("真字符串")) -> (0:w1325:string)  [unwired: 1 in]
            n560 = Build Array (concatenate)(w1334, w1324, w1325) -> (w1332:string[])
            n561 = Flatten To XML(anything=w1332) -> (xml string=w1331:string)
            n562 = call "AMC Send Local Message.vi"("Process (\"\" - local)"=w1333, "Message Value"=w1331, "Message Name"=w1333) -> ()  [unwired: 7 in, 2 out]
          }
        }
        n563 = call <vilib>:"Space Constant.vi"() -> ("String"=w1310:string)
        n564 = Concatenate Strings(w1307, w1310, w1309) -> (w1311:string)
        n565 = call "LogStatus.vi"("error in (no error)"=w1302, "last message"=w1313, "message"=w1311) -> ("error  out"=w1314:errorcluster)  [unwired: 8 in]
        n566 = case shown="Error" w1302 {
          tunnel: [_ TRUE] -> w1304
          tunnel: [_ "Error"] -> w1305
          frame No Error {
          }
          frame Error {
          }
        }
      }
      frame "Check Test item “Distortation_Center Y” result" {
        n567 = Unbundle By Name(w1338) -> ("Table"=w1345:string[][])
        n568 = call "Select_Table_Vaule Enable_Disable.vi"("Action"=w1344, "Table"=w1345) -> ("Enable"=w1343:bool)  [unwired: 8 in, 1 out]
        n569 = case shown="True" w1343 {
          tunnel: ["Skip" ("response") w1361] -> w1346
          tunnel: w1345 -> [_ w1364]
          tunnel: w1344 -> [_ w1363]
          tunnel: [_ w1357] -> w1339
          tunnel: w1337 -> [_ _]
          frame False {
          }
          frame True {
            w1370 = "UIdisplay" ("Process (\"\" - local)")
            # "TBD"
            # "Config external Light"
            n570 = call "SendCmd.vi"() -> ("error out"=w1357:errorcluster, "standard output"=w1358:string, "return code"=w1360:i32, "standard error"=w1359:string)  [unwired: 8 in]
            n571 = Equal To 0?(x=w1360) -> (x = 0?=w1356:bool)
            n572 = case shown="True" w1356 {
              tunnel: w1358 -> [_ w1373]
              tunnel: [w1372 w1373] -> w1361
              tunnel: w1359 -> [w1372 _]
              frame False {
              }
              frame True {
              }
            }
            n573 = call "Select_Table_Vaule.vi"("Vaule"=w1361, "Action"=w1363, "Table"=w1364) -> ("Result"=w1365:bool, "vaule"=w1371:string[])  [unwired: 7 in]
            n574 = Append True/False String(1:w1365, 2:"FAIL" ("真字符串"), 3:"PASS" ("真字符串")) -> (0:w1362:string)  [unwired: 1 in]
            n575 = Build Array (concatenate)(w1371, w1361, w1362) -> (w1369:string[])
            n576 = Flatten To XML(anything=w1369) -> (xml string=w1368:string)
            n577 = call "AMC Send Local Message.vi"("Process (\"\" - local)"=w1370, "Message Value"=w1368, "Message Name"=w1370) -> ()  [unwired: 7 in, 2 out]
          }
        }
        n578 = call <vilib>:"Space Constant.vi"() -> ("String"=w1347:string)
        n579 = Concatenate Strings(w1344, w1347, w1346) -> (w1348:string)
        n580 = call "LogStatus.vi"("error in (no error)"=w1339, "last message"=w1350, "message"=w1348) -> ("error  out"=w1351:errorcluster)  [unwired: 8 in]
        n581 = case shown="Error" w1339 {
          tunnel: [_ TRUE] -> w1341
          tunnel: [_ "Error"] -> w1342
          frame No Error {
          }
          frame Error {
          }
        }
      }
      frame "Check Test item “Distortation %” result" {
        n582 = Unbundle By Name(w1375) -> ("Table"=w1382:string[][])
        n583 = call "Select_Table_Vaule Enable_Disable.vi"("Action"=w1381, "Table"=w1382) -> ("Enable"=w1380:bool)  [unwired: 8 in, 1 out]
        n584 = case shown="True" w1380 {
          tunnel: ["Skip" ("response") w1398] -> w1383
          tunnel: w1382 -> [_ w1401]
          tunnel: w1381 -> [_ w1400]
          tunnel: [_ w1394] -> w1376
          tunnel: w1374 -> [_ _]
          frame False {
          }
          frame True {
            w1407 = "UIdisplay" ("Process (\"\" - local)")
            # "<75%"
            # "Config external Light"
            n585 = call "SendCmd.vi"() -> ("error out"=w1394:errorcluster, "standard output"=w1395:string, "return code"=w1397:i32, "standard error"=w1396:string)  [unwired: 8 in]
            n586 = Equal To 0?(x=w1397) -> (x = 0?=w1393:bool)
            n587 = case shown="True" w1393 {
              tunnel: w1395 -> [_ w1410]
              tunnel: [w1409 w1410] -> w1398
              tunnel: w1396 -> [w1409 _]
              frame False {
              }
              frame True {
              }
            }
            n588 = call "Select_Table_Vaule.vi"("Vaule"=w1398, "Action"=w1400, "Table"=w1401) -> ("Result"=w1402:bool, "vaule"=w1408:string[])  [unwired: 7 in]
            n589 = Append True/False String(1:w1402, 2:"FAIL" ("真字符串"), 3:"PASS" ("真字符串")) -> (0:w1399:string)  [unwired: 1 in]
            n590 = Build Array (concatenate)(w1408, w1398, w1399) -> (w1406:string[])
            n591 = Flatten To XML(anything=w1406) -> (xml string=w1405:string)
            n592 = call "AMC Send Local Message.vi"("Process (\"\" - local)"=w1407, "Message Value"=w1405, "Message Name"=w1407) -> ()  [unwired: 7 in, 2 out]
          }
        }
        n593 = call <vilib>:"Space Constant.vi"() -> ("String"=w1384:string)
        n594 = Concatenate Strings(w1381, w1384, w1383) -> (w1385:string)
        n595 = call "LogStatus.vi"("error in (no error)"=w1376, "last message"=w1387, "message"=w1385) -> ("error  out"=w1388:errorcluster)  [unwired: 8 in]
        n596 = case shown="Error" w1376 {
          tunnel: [_ TRUE] -> w1378
          tunnel: [_ "Error"] -> w1379
          frame No Error {
          }
          frame Error {
          }
        }
      }
      frame "Check Test item “MFT50” result" {
        n597 = Unbundle By Name(w1412) -> ("Table"=w1419:string[][])
        n598 = call "Select_Table_Vaule Enable_Disable.vi"("Action"=w1418, "Table"=w1419) -> ("Enable"=w1417:bool)  [unwired: 8 in, 1 out]
        n599 = case shown="True" w1417 {
          tunnel: ["Skip" ("response") w1435] -> w1420
          tunnel: w1419 -> [_ w1438]
          tunnel: w1418 -> [_ w1437]
          tunnel: [_ w1431] -> w1413
          tunnel: w1411 -> [_ _]
          frame False {
          }
          frame True {
            w1444 = "UIdisplay" ("Process (\"\" - local)")
            # ">0.25"
            # "Config external Light"
            n600 = call "SendCmd.vi"() -> ("error out"=w1431:errorcluster, "standard output"=w1432:string, "return code"=w1434:i32, "standard error"=w1433:string)  [unwired: 8 in]
            n601 = Equal To 0?(x=w1434) -> (x = 0?=w1430:bool)
            n602 = case shown="True" w1430 {
              tunnel: w1432 -> [_ w1447]
              tunnel: [w1446 w1447] -> w1435
              tunnel: w1433 -> [w1446 _]
              frame False {
              }
              frame True {
              }
            }
            n603 = call "Select_Table_Vaule.vi"("Vaule"=w1435, "Action"=w1437, "Table"=w1438) -> ("Result"=w1439:bool, "vaule"=w1445:string[])  [unwired: 7 in]
            n604 = Append True/False String(1:w1439, 2:"FAIL" ("真字符串"), 3:"PASS" ("真字符串")) -> (0:w1436:string)  [unwired: 1 in]
            n605 = Build Array (concatenate)(w1445, w1435, w1436) -> (w1443:string[])
            n606 = Flatten To XML(anything=w1443) -> (xml string=w1442:string)
            n607 = call "AMC Send Local Message.vi"("Process (\"\" - local)"=w1444, "Message Value"=w1442, "Message Name"=w1444) -> ()  [unwired: 7 in, 2 out]
          }
        }
        n608 = call <vilib>:"Space Constant.vi"() -> ("String"=w1421:string)
        n609 = Concatenate Strings(w1418, w1421, w1420) -> (w1422:string)
        n610 = call "LogStatus.vi"("error in (no error)"=w1413, "last message"=w1424, "message"=w1422) -> ("error  out"=w1425:errorcluster)  [unwired: 8 in]
        n611 = case shown="Error" w1413 {
          tunnel: [_ TRUE] -> w1415
          tunnel: [_ "Error"] -> w1416
          frame No Error {
          }
          frame Error {
          }
        }
      }
      frame "Check Test item “Rise Distance” result" {
        n612 = Unbundle By Name(w1449) -> ("Table"=w1456:string[][])
        n613 = call "Select_Table_Vaule Enable_Disable.vi"("Action"=w1455, "Table"=w1456) -> ("Enable"=w1454:bool)  [unwired: 8 in, 1 out]
        n614 = case shown="True" w1454 {
          tunnel: ["Skip" ("response") w1472] -> w1457
          tunnel: w1456 -> [_ w1475]
          tunnel: w1455 -> [_ w1474]
          tunnel: [_ w1468] -> w1450
          tunnel: w1448 -> [_ _]
          frame False {
          }
          frame True {
            w1481 = "UIdisplay" ("Process (\"\" - local)")
            # "<2.5"
            # "Config external Light"
            n615 = call "SendCmd.vi"() -> ("error out"=w1468:errorcluster, "standard output"=w1469:string, "return code"=w1471:i32, "standard error"=w1470:string)  [unwired: 8 in]
            n616 = Equal To 0?(x=w1471) -> (x = 0?=w1467:bool)
            n617 = case shown="True" w1467 {
              tunnel: w1469 -> [_ w1484]
              tunnel: [w1483 w1484] -> w1472
              tunnel: w1470 -> [w1483 _]
              frame False {
              }
              frame True {
              }
            }
            n618 = call "Select_Table_Vaule.vi"("Vaule"=w1472, "Action"=w1474, "Table"=w1475) -> ("Result"=w1476:bool, "vaule"=w1482:string[])  [unwired: 7 in]
            n619 = Append True/False String(1:w1476, 2:"FAIL" ("真字符串"), 3:"PASS" ("真字符串")) -> (0:w1473:string)  [unwired: 1 in]
            n620 = Build Array (concatenate)(w1482, w1472, w1473) -> (w1480:string[])
            n621 = Flatten To XML(anything=w1480) -> (xml string=w1479:string)
            n622 = call "AMC Send Local Message.vi"("Process (\"\" - local)"=w1481, "Message Value"=w1479, "Message Name"=w1481) -> ()  [unwired: 7 in, 2 out]
          }
        }
        n623 = call <vilib>:"Space Constant.vi"() -> ("String"=w1458:string)
        n624 = Concatenate Strings(w1455, w1458, w1457) -> (w1459:string)
        n625 = call "LogStatus.vi"("error in (no error)"=w1450, "last message"=w1461, "message"=w1459) -> ("error  out"=w1462:errorcluster)  [unwired: 8 in]
        n626 = case shown="Error" w1450 {
          tunnel: [_ TRUE] -> w1452
          tunnel: [_ "Error"] -> w1453
          frame No Error {
          }
          frame Error {
          }
        }
      }
      frame "VQT Test result" {
        n627 = Unbundle By Name(w1486) -> ("Table"=w1493:string[][])
        n628 = call "Select_Table_Vaule Enable_Disable.vi"("Action"=w1492, "Table"=w1493) -> ("Enable"=w1491:bool)  [unwired: 8 in, 1 out]
        n629 = case shown="True" w1491 {
          tunnel: ["Skip" ("response") w1509] -> w1494
          tunnel: w1493 -> [_ w1512]
          tunnel: w1492 -> [_ w1511]
          tunnel: [_ w1505] -> w1487
          tunnel: w1485 -> [_ _]
          frame False {
          }
          frame True {
            w1518 = "UIdisplay" ("Process (\"\" - local)")
            # "VQT Test result"
            # "Config external Light"
            n630 = call "SendCmd.vi"() -> ("error out"=w1505:errorcluster, "standard output"=w1506:string, "return code"=w1508:i32, "standard error"=w1507:string)  [unwired: 8 in]
            n631 = Equal To 0?(x=w1508) -> (x = 0?=w1504:bool)
            n632 = case shown="True" w1504 {
              tunnel: w1506 -> [_ w1521]
              tunnel: [w1520 w1521] -> w1509
              tunnel: w1507 -> [w1520 _]
              frame False {
              }
              frame True {
              }
            }
            n633 = call "Select_Table_Vaule.vi"("Vaule"=w1509, "Action"=w1511, "Table"=w1512) -> ("Result"=w1513:bool, "vaule"=w1519:string[])  [unwired: 7 in]
            n634 = Append True/False String(1:w1513, 2:"FAIL" ("真字符串"), 3:"PASS" ("真字符串")) -> (0:w1510:string)  [unwired: 1 in]
            n635 = Build Array (concatenate)(w1519, w1509, w1510) -> (w1517:string[])
            n636 = Flatten To XML(anything=w1517) -> (xml string=w1516:string)
            n637 = call "AMC Send Local Message.vi"("Process (\"\" - local)"=w1518, "Message Value"=w1516, "Message Name"=w1518) -> ()  [unwired: 7 in, 2 out]
          }
        }
        n638 = call <vilib>:"Space Constant.vi"() -> ("String"=w1495:string)
        n639 = Concatenate Strings(w1492, w1495, w1494) -> (w1496:string)
        n640 = call "LogStatus.vi"("error in (no error)"=w1487, "last message"=w1498, "message"=w1496) -> ("error  out"=w1499:errorcluster)  [unwired: 8 in]
        n641 = case shown="Error" w1487 {
          tunnel: [_ TRUE] -> w1489
          tunnel: [_ "Error"] -> w1490
          frame No Error {
          }
          frame Error {
          }
        }
      }
      frame "Check Test item” RBdeltaE” result" {
        n642 = Unbundle By Name(w1523) -> ("Table"=w1530:string[][])
        n643 = call "Select_Table_Vaule Enable_Disable.vi"("Action"=w1529, "Table"=w1530) -> ("Enable"=w1528:bool)  [unwired: 8 in, 1 out]
        n644 = case shown="True" w1528 {
          tunnel: ["Skip" ("response") w1546] -> w1531
          tunnel: w1530 -> [_ w1549]
          tunnel: w1529 -> [_ w1548]
          tunnel: [_ w1542] -> w1524
          tunnel: w1522 -> [_ _]
          frame False {
          }
          frame True {
            w1555 = "UIdisplay" ("Process (\"\" - local)")
            # "35~45"
            # "Config external Light"
            n645 = call "SendCmd.vi"() -> ("error out"=w1542:errorcluster, "standard output"=w1543:string, "return code"=w1545:i32, "standard error"=w1544:string)  [unwired: 8 in]
            n646 = Equal To 0?(x=w1545) -> (x = 0?=w1541:bool)
            n647 = case shown="True" w1541 {
              tunnel: w1543 -> [_ w1558]
              tunnel: [w1557 w1558] -> w1546
              tunnel: w1544 -> [w1557 _]
              frame False {
              }
              frame True {
              }
            }
            n648 = call "Select_Table_Vaule.vi"("Vaule"=w1546, "Action"=w1548, "Table"=w1549) -> ("Result"=w1550:bool, "vaule"=w1556:string[])  [unwired: 7 in]
            n649 = Append True/False String(1:w1550, 2:"FAIL" ("真字符串"), 3:"PASS" ("真字符串")) -> (0:w1547:string)  [unwired: 1 in]
            n650 = Build Array (concatenate)(w1556, w1546, w1547) -> (w1554:string[])
            n651 = Flatten To XML(anything=w1554) -> (xml string=w1553:string)
            n652 = call "AMC Send Local Message.vi"("Process (\"\" - local)"=w1555, "Message Value"=w1553, "Message Name"=w1555) -> ()  [unwired: 7 in, 2 out]
          }
        }
        n653 = call <vilib>:"Space Constant.vi"() -> ("String"=w1532:string)
        n654 = Concatenate Strings(w1529, w1532, w1531) -> (w1533:string)
        n655 = call "LogStatus.vi"("error in (no error)"=w1524, "last message"=w1535, "message"=w1533) -> ("error  out"=w1536:errorcluster)  [unwired: 8 in]
        n656 = case shown="Error" w1524 {
          tunnel: [_ TRUE] -> w1526
          tunnel: [_ "Error"] -> w1527
          frame No Error {
          }
          frame Error {
          }
        }
      }
      frame "Check Test item” BWdeltaE” result" {
        n657 = Unbundle By Name(w1560) -> ("Table"=w1567:string[][])
        n658 = call "Select_Table_Vaule Enable_Disable.vi"("Action"=w1566, "Table"=w1567) -> ("Enable"=w1565:bool)  [unwired: 8 in, 1 out]
        n659 = case shown="True" w1565 {
          tunnel: ["Skip" ("response") w1583] -> w1568
          tunnel: w1567 -> [_ w1586]
          tunnel: w1566 -> [_ w1585]
          tunnel: [_ w1579] -> w1561
          tunnel: w1559 -> [_ _]
          frame False {
          }
          frame True {
            w1592 = "UIdisplay" ("Process (\"\" - local)")
            # ">80"
            # "Config external Light"
            n660 = call "SendCmd.vi"() -> ("error out"=w1579:errorcluster, "standard output"=w1580:string, "return code"=w1582:i32, "standard error"=w1581:string)  [unwired: 8 in]
            n661 = Equal To 0?(x=w1582) -> (x = 0?=w1578:bool)
            n662 = case shown="True" w1578 {
              tunnel: w1580 -> [_ w1595]
              tunnel: [w1594 w1595] -> w1583
              tunnel: w1581 -> [w1594 _]
              frame False {
              }
              frame True {
              }
            }
            n663 = call "Select_Table_Vaule.vi"("Vaule"=w1583, "Action"=w1585, "Table"=w1586) -> ("Result"=w1587:bool, "vaule"=w1593:string[])  [unwired: 7 in]
            n664 = Append True/False String(1:w1587, 2:"FAIL" ("真字符串"), 3:"PASS" ("真字符串")) -> (0:w1584:string)  [unwired: 1 in]
            n665 = Build Array (concatenate)(w1593, w1583, w1584) -> (w1591:string[])
            n666 = Flatten To XML(anything=w1591) -> (xml string=w1590:string)
            n667 = call "AMC Send Local Message.vi"("Process (\"\" - local)"=w1592, "Message Value"=w1590, "Message Name"=w1592) -> ()  [unwired: 7 in, 2 out]
          }
        }
        n668 = call <vilib>:"Space Constant.vi"() -> ("String"=w1569:string)
        n669 = Concatenate Strings(w1566, w1569, w1568) -> (w1570:string)
        n670 = call "LogStatus.vi"("error in (no error)"=w1561, "last message"=w1572, "message"=w1570) -> ("error  out"=w1573:errorcluster)  [unwired: 8 in]
        n671 = case shown="Error" w1561 {
          tunnel: [_ TRUE] -> w1563
          tunnel: [_ "Error"] -> w1564
          frame No Error {
          }
          frame Error {
          }
        }
      }
      frame "Check Test item” WRdeltaE” result" {
        n672 = Unbundle By Name(w1597) -> ("Table"=w1604:string[][])
        n673 = call "Select_Table_Vaule Enable_Disable.vi"("Action"=w1603, "Table"=w1604) -> ("Enable"=w1602:bool)  [unwired: 8 in, 1 out]
        n674 = case shown="True" w1602 {
          tunnel: ["Skip" ("response") w1620] -> w1605
          tunnel: w1604 -> [_ w1623]
          tunnel: w1603 -> [_ w1622]
          tunnel: [_ w1616] -> w1598
          tunnel: w1596 -> [_ _]
          frame False {
          }
          frame True {
            w1629 = "UIdisplay" ("Process (\"\" - local)")
            # "45~58"
            # "Config external Light"
            n675 = call "SendCmd.vi"() -> ("error out"=w1616:errorcluster, "standard output"=w1617:string, "return code"=w1619:i32, "standard error"=w1618:string)  [unwired: 8 in]
            n676 = Equal To 0?(x=w1619) -> (x = 0?=w1615:bool)
            n677 = case shown="True" w1615 {
              tunnel: w1617 -> [_ w1632]
              tunnel: [w1631 w1632] -> w1620
              tunnel: w1618 -> [w1631 _]
              frame False {
              }
              frame True {
              }
            }
            n678 = call "Select_Table_Vaule.vi"("Vaule"=w1620, "Action"=w1622, "Table"=w1623) -> ("Result"=w1624:bool, "vaule"=w1630:string[])  [unwired: 7 in]
            n679 = Append True/False String(1:w1624, 2:"FAIL" ("真字符串"), 3:"PASS" ("真字符串")) -> (0:w1621:string)  [unwired: 1 in]
            n680 = Build Array (concatenate)(w1630, w1620, w1621) -> (w1628:string[])
            n681 = Flatten To XML(anything=w1628) -> (xml string=w1627:string)
            n682 = call "AMC Send Local Message.vi"("Process (\"\" - local)"=w1629, "Message Value"=w1627, "Message Name"=w1629) -> ()  [unwired: 7 in, 2 out]
          }
        }
        n683 = call <vilib>:"Space Constant.vi"() -> ("String"=w1606:string)
        n684 = Concatenate Strings(w1603, w1606, w1605) -> (w1607:string)
        n685 = call "LogStatus.vi"("error in (no error)"=w1598, "last message"=w1609, "message"=w1607) -> ("error  out"=w1610:errorcluster)  [unwired: 8 in]
        n686 = case shown="Error" w1598 {
          tunnel: [_ TRUE] -> w1600
          tunnel: [_ "Error"] -> w1601
          frame No Error {
          }
          frame Error {
          }
        }
      }
      frame "Check Test item” deltaa” result" {
        n687 = Unbundle By Name(w1634) -> ("Table"=w1641:string[][])
        n688 = call "Select_Table_Vaule Enable_Disable.vi"("Action"=w1640, "Table"=w1641) -> ("Enable"=w1639:bool)  [unwired: 8 in, 1 out]
        n689 = case shown="True" w1639 {
          tunnel: ["Skip" ("response") w1657] -> w1642
          tunnel: w1641 -> [_ w1660]
          tunnel: w1640 -> [_ w1659]
          tunnel: [_ w1653] -> w1635
          tunnel: w1633 -> [_ _]
          frame False {
          }
          frame True {
            w1666 = "UIdisplay" ("Process (\"\" - local)")
            # "<2.0"
            # "Config external Light"
            n690 = call "SendCmd.vi"() -> ("error out"=w1653:errorcluster, "standard output"=w1654:string, "return code"=w1656:i32, "standard error"=w1655:string)  [unwired: 8 in]
            n691 = Equal To 0?(x=w1656) -> (x = 0?=w1652:bool)
            n692 = case shown="True" w1652 {
              tunnel: w1654 -> [_ w1669]
              tunnel: [w1668 w1669] -> w1657
              tunnel: w1655 -> [w1668 _]
              frame False {
              }
              frame True {
              }
            }
            n693 = call "Select_Table_Vaule.vi"("Vaule"=w1657, "Action"=w1659, "Table"=w1660) -> ("Result"=w1661:bool, "vaule"=w1667:string[])  [unwired: 7 in]
            n694 = Append True/False String(1:w1661, 2:"FAIL" ("真字符串"), 3:"PASS" ("真字符串")) -> (0:w1658:string)  [unwired: 1 in]
            n695 = Build Array (concatenate)(w1667, w1657, w1658) -> (w1665:string[])
            n696 = Flatten To XML(anything=w1665) -> (xml string=w1664:string)
            n697 = call "AMC Send Local Message.vi"("Process (\"\" - local)"=w1666, "Message Value"=w1664, "Message Name"=w1666) -> ()  [unwired: 7 in, 2 out]
          }
        }
        n698 = call <vilib>:"Space Constant.vi"() -> ("String"=w1643:string)
        n699 = Concatenate Strings(w1640, w1643, w1642) -> (w1644:string)
        n700 = call "LogStatus.vi"("error in (no error)"=w1635, "last message"=w1646, "message"=w1644) -> ("error  out"=w1647:errorcluster)  [unwired: 8 in]
        n701 = case shown="Error" w1635 {
          tunnel: [_ TRUE] -> w1637
          tunnel: [_ "Error"] -> w1638
          frame No Error {
          }
          frame Error {
          }
        }
      }
      frame "Check Test item” deltab” result" {
        n702 = Unbundle By Name(w1671) -> ("Table"=w1678:string[][])
        n703 = call "Select_Table_Vaule Enable_Disable.vi"("Action"=w1677, "Table"=w1678) -> ("Enable"=w1676:bool)  [unwired: 8 in, 1 out]
        n704 = case shown="True" w1676 {
          tunnel: ["Skip" ("response") w1694] -> w1679
          tunnel: w1678 -> [_ w1697]
          tunnel: w1677 -> [_ w1696]
          tunnel: [_ w1690] -> w1672
          tunnel: w1670 -> [_ _]
          frame False {
          }
          frame True {
            w1703 = "UIdisplay" ("Process (\"\" - local)")
            # "<2.0"
            n705 = call "SendCmd.vi"() -> ("error out"=w1690:errorcluster, "standard output"=w1691:string, "return code"=w1693:i32, "standard error"=w1692:string)  [unwired: 8 in]
            n706 = Equal To 0?(x=w1693) -> (x = 0?=w1689:bool)
            n707 = case shown="True" w1689 {
              tunnel: w1691 -> [_ w1706]
              tunnel: [w1705 w1706] -> w1694
              tunnel: w1692 -> [w1705 _]
              frame False {
              }
              frame True {
              }
            }
            n708 = call "Select_Table_Vaule.vi"("Vaule"=w1694, "Action"=w1696, "Table"=w1697) -> ("Result"=w1698:bool, "vaule"=w1704:string[])  [unwired: 7 in]
            n709 = Append True/False String(1:w1698, 2:"FAIL" ("真字符串"), 3:"PASS" ("真字符串")) -> (0:w1695:string)  [unwired: 1 in]
            n710 = Build Array (concatenate)(w1704, w1694, w1695) -> (w1702:string[])
            n711 = Flatten To XML(anything=w1702) -> (xml string=w1701:string)
            n712 = call "AMC Send Local Message.vi"("Process (\"\" - local)"=w1703, "Message Value"=w1701, "Message Name"=w1703) -> ()  [unwired: 7 in, 2 out]
          }
        }
        n713 = call <vilib>:"Space Constant.vi"() -> ("String"=w1680:string)
        n714 = Concatenate Strings(w1677, w1680, w1679) -> (w1681:string)
        n715 = call "LogStatus.vi"("error in (no error)"=w1672, "last message"=w1683, "message"=w1681) -> ("error  out"=w1684:errorcluster)  [unwired: 8 in]
        n716 = case shown="Error" w1672 {
          tunnel: [_ TRUE] -> w1674
          tunnel: [_ "Error"] -> w1675
          frame No Error {
          }
          frame Error {
          }
        }
      }
      frame "Color Check Results" {
        n717 = Unbundle By Name(w1708) -> ("Table"=w1715:string[][])
        n718 = call "Select_Table_Vaule Enable_Disable.vi"("Action"=w1714, "Table"=w1715) -> ("Enable"=w1713:bool)  [unwired: 8 in, 1 out]
        n719 = case shown="True" w1713 {
          tunnel: ["Skip" ("response") w1731] -> w1716
          tunnel: w1715 -> [_ w1734]
          tunnel: w1714 -> [_ w1733]
          tunnel: [_ w1727] -> w1709
          tunnel: w1707 -> [_ _]
          frame False {
          }
          frame True {
            w1740 = "UIdisplay" ("Process (\"\" - local)")
            # "Color Check Results"
            n720 = call "SendCmd.vi"() -> ("error out"=w1727:errorcluster, "standard output"=w1728:string, "return code"=w1730:i32, "standard error"=w1729:string)  [unwired: 8 in]
            n721 = Equal To 0?(x=w1730) -> (x = 0?=w1726:bool)
            n722 = case shown="True" w1726 {
              tunnel: w1728 -> [_ w1743]
              tunnel: [w1742 w1743] -> w1731
              tunnel: w1729 -> [w1742 _]
              frame False {
              }
              frame True {
              }
            }
            n723 = call "Select_Table_Vaule.vi"("Vaule"=w1731, "Action"=w1733, "Table"=w1734) -> ("Result"=w1735:bool, "vaule"=w1741:string[])  [unwired: 7 in]
            n724 = Append True/False String(1:w1735, 2:"FAIL" ("真字符串"), 3:"PASS" ("真字符串")) -> (0:w1732:string)  [unwired: 1 in]
            n725 = Build Array (concatenate)(w1741, w1731, w1732) -> (w1739:string[])
            n726 = Flatten To XML(anything=w1739) -> (xml string=w1738:string)
            n727 = call "AMC Send Local Message.vi"("Process (\"\" - local)"=w1740, "Message Value"=w1738, "Message Name"=w1740) -> ()  [unwired: 7 in, 2 out]
          }
        }
        n728 = call <vilib>:"Space Constant.vi"() -> ("String"=w1717:string)
        n729 = Concatenate Strings(w1714, w1717, w1716) -> (w1718:string)
        n730 = call "LogStatus.vi"("error in (no error)"=w1709, "last message"=w1720, "message"=w1718) -> ("error  out"=w1721:errorcluster)  [unwired: 8 in]
        n731 = case shown="Error" w1709 {
          tunnel: [_ TRUE] -> w1711
          tunnel: [_ "Error"] -> w1712
          frame No Error {
          }
          frame Error {
          }
        }
      }
      frame "Stop Camera" {
        n732 = Unbundle By Name(w1745) -> ("Table"=w1752:string[][])
        n733 = call "Select_Table_Vaule Enable_Disable.vi"("Action"=w1751, "Table"=w1752) -> ("Enable"=w1750:bool)  [unwired: 8 in, 1 out]
        n734 = case shown="True" w1750 {
          tunnel: ["Skip" ("response") w1771] -> w1753
          tunnel: w1752 -> [_ w1774]
          tunnel: w1751 -> [_ w1773]
          tunnel: [_ w1767] -> w1746
          tunnel: w1744 -> [_ w1765]
          frame False {
          }
          frame True {
            w1780 = "UIdisplay" ("Process (\"\" - local)")
            # "Color Check Results"
            n735 = Unbundle By Name(w1765) -> ("Stop Camera"=w1764:string)
            n736 = call "SendCmd.vi"("cmd"=w1764, "exe"="D:\\Program Files\\MVTec\\HALCON-17.12-Progress\\bin\\x64-win64\\hdevelop.exe") -> ("error out"=w1767:errorcluster, "standard output"=w1768:string, "return code"=w1770:i32, "standard error"=w1769:string)  [unwired: 6 in]
            n737 = Equal To 0?(x=w1770) -> (x = 0?=w1766:bool)
            n738 = case shown="True" w1766 {
              tunnel: w1768 -> [_ w1783]
              tunnel: [w1782 w1783] -> w1771
              tunnel: w1769 -> [w1782 _]
              frame False {
              }
              frame True {
              }
            }
            n739 = call "Select_Table_Vaule.vi"("Vaule"=w1771, "Action"=w1773, "Table"=w1774) -> ("Result"=w1775:bool, "vaule"=w1781:string[])  [unwired: 7 in]
            n740 = Append True/False String(1:w1775, 2:"FAIL" ("真字符串"), 3:"PASS" ("真字符串")) -> (0:w1772:string)  [unwired: 1 in]
            n741 = Build Array (concatenate)(w1781, w1771, w1772) -> (w1779:string[])
            n742 = Flatten To XML(anything=w1779) -> (xml string=w1778:string)
            n743 = call "AMC Send Local Message.vi"("Process (\"\" - local)"=w1780, "Message Value"=w1778, "Message Name"=w1780) -> ()  [unwired: 7 in, 2 out]
          }
        }
        n744 = call <vilib>:"Space Constant.vi"() -> ("String"=w1754:string)
        n745 = Concatenate Strings(w1751, w1754, w1753) -> (w1755:string)
        n746 = call "LogStatus.vi"("error in (no error)"=w1746, "last message"=w1757, "message"=w1755) -> ("error  out"=w1758:errorcluster)  [unwired: 8 in]
        n747 = case shown="Error" w1746 {
          tunnel: [_ TRUE] -> w1748
          tunnel: [_ "Error"] -> w1749
          frame No Error {
          }
          frame Error {
          }
        }
      }
      frame "Stop Test mode" {
        n748 = Unbundle By Name(w1785) -> ("Table"=w1792:string[][])
        n749 = call "Select_Table_Vaule Enable_Disable.vi"("Action"=w1791, "Table"=w1792) -> ("Enable"=w1790:bool)  [unwired: 8 in, 1 out]
        n750 = case shown="True" w1790 {
          tunnel: ["Skip" ("response") w1811] -> w1793
          tunnel: w1792 -> [_ w1814]
          tunnel: w1791 -> [_ w1813]
          tunnel: [_ w1807] -> w1786
          tunnel: w1784 -> [_ w1805]
          frame False {
          }
          frame True {
            w1820 = "UIdisplay" ("Process (\"\" - local)")
            # "Stop Test mode"
            n751 = Unbundle By Name(w1805) -> ("Stop Test Mode"=w1804:string)
            n752 = call "SendCmd.vi"("cmd"=w1804, "exe"="D:\\Program Files\\MVTec\\HALCON-17.12-Progress\\bin\\x64-win64\\hdevelop.exe") -> ("error out"=w1807:errorcluster, "standard output"=w1808:string, "return code"=w1810:i32, "standard error"=w1809:string)  [unwired: 6 in]
            n753 = Equal To 0?(x=w1810) -> (x = 0?=w1806:bool)
            n754 = case shown="True" w1806 {
              tunnel: w1808 -> [_ w1823]
              tunnel: [w1822 w1823] -> w1811
              tunnel: w1809 -> [w1822 _]
              frame False {
              }
              frame True {
              }
            }
            n755 = call "Select_Table_Vaule.vi"("Vaule"=w1811, "Action"=w1813, "Table"=w1814) -> ("Result"=w1815:bool, "vaule"=w1821:string[])  [unwired: 7 in]
            n756 = Append True/False String(1:w1815, 2:"FAIL" ("真字符串"), 3:"PASS" ("真字符串")) -> (0:w1812:string)  [unwired: 1 in]
            n757 = Build Array (concatenate)(w1821, w1811, w1812) -> (w1819:string[])
            n758 = Flatten To XML(anything=w1819) -> (xml string=w1818:string)
            n759 = call "AMC Send Local Message.vi"("Process (\"\" - local)"=w1820, "Message Value"=w1818, "Message Name"=w1820) -> ()  [unwired: 7 in, 2 out]
          }
        }
        n760 = call <vilib>:"Space Constant.vi"() -> ("String"=w1794:string)
        n761 = Concatenate Strings(w1791, w1794, w1793) -> (w1795:string)
        n762 = call "LogStatus.vi"("error in (no error)"=w1786, "last message"=w1797, "message"=w1795) -> ("error  out"=w1798:errorcluster)  [unwired: 8 in]
        n763 = case shown="Error" w1786 {
          tunnel: [_ TRUE] -> w1788
          tunnel: [_ "Error"] -> w1789
          frame No Error {
          }
          frame Error {
          }
        }
      }
      frame "Shutdown UUT" {
        (unwired) TRUE
        n764 = Unbundle By Name(w1825) -> ("Table"=w1832:string[][])
        n765 = call "Select_Table_Vaule Enable_Disable.vi"("Action"=w1831, "Table"=w1832) -> ("Enable"=w1830:bool)  [unwired: 8 in, 1 out]
        n766 = case shown="True" w1830 {
          tunnel: ["Skip" ("response") w1851] -> w1833
          tunnel: w1832 -> [_ w1854]
          tunnel: w1831 -> [_ w1853]
          tunnel: [_ w1847] -> w1826
          tunnel: w1824 -> [_ w1845]
          frame False {
          }
          frame True {
            w1860 = "UIdisplay" ("Process (\"\" - local)")
            # "TBD"
            n767 = Unbundle By Name(w1845) -> ("Stop Test Mode"=w1844:string)
            n768 = call "SendCmd.vi"("cmd"=w1844, "exe"="D:\\Program Files\\MVTec\\HALCON-17.12-Progress\\bin\\x64-win64\\hdevelop.exe") -> ("error out"=w1847:errorcluster, "standard output"=w1848:string, "return code"=w1850:i32, "standard error"=w1849:string)  [unwired: 6 in]
            n769 = Equal To 0?(x=w1850) -> (x = 0?=w1846:bool)
            n770 = case shown="True" w1846 {
              tunnel: w1848 -> [_ w1863]
              tunnel: [w1862 w1863] -> w1851
              tunnel: w1849 -> [w1862 _]
              frame False {
              }
              frame True {
              }
            }
            n771 = call "Select_Table_Vaule.vi"("Vaule"=w1851, "Action"=w1853, "Table"=w1854) -> ("Result"=w1855:bool, "vaule"=w1861:string[])  [unwired: 7 in]
            n772 = Append True/False String(1:w1855, 2:"FAIL" ("真字符串"), 3:"PASS" ("真字符串")) -> (0:w1852:string)  [unwired: 1 in]
            n773 = Build Array (concatenate)(w1861, w1851, w1852) -> (w1859:string[])
            n774 = Flatten To XML(anything=w1859) -> (xml string=w1858:string)
            n775 = call "AMC Send Local Message.vi"("Process (\"\" - local)"=w1860, "Message Value"=w1858, "Message Name"=w1860) -> ()  [unwired: 7 in, 2 out]
          }
        }
        n776 = call <vilib>:"Space Constant.vi"() -> ("String"=w1834:string)
        n777 = Concatenate Strings(w1831, w1834, w1833) -> (w1835:string)
        n778 = call "LogStatus.vi"("error in (no error)"=w1826, "last message"=w1837, "message"=w1835) -> ("error  out"=w1838:errorcluster)  [unwired: 8 in]
        n779 = case shown="Error" w1826 {
          tunnel: [_ TRUE] -> w1828
          tunnel: [_ "Error"] -> w1829
          frame No Error {
          }
          frame Error {
          }
        }
      }
      frame "ECO_MODE" {
        w1875 = "UIdisplay" ("Process (\"\" - local)")
        w1871 = "Enable" ("元素")
        n780 = Unbundle By Name(w1866) -> ("Table"=w1874:string[][])
        n781 = call "LogStatus.vi"("error in (no error)"=w1891, "last message"=w1890, "message"=w1872) -> ("error  out"=w1889:errorcluster)  [unwired: 8 in]
        n782 = call "Select_Table_Vaule.vi"("Vaule"=w1871, "Action"=w1872, "Table"=w1874) -> ("Result"=w1882:bool, "vaule"=w1881:string[])  [unwired: 7 in]
        n783 = call "3.1.0_ECO_Mode.vi"("Data in"=w1866, "error in (no error)"=w1889, "AllControls In"=w1864, 10:w1873, "Message Queue out"=w1887) -> ("error out"=w1888:errorcluster, "Flow"=w1870:string, "Data"=w1885:T4, "Message Queue Out"=w1886:T5, "Data out"=w1865:T1)  [unwired: 2 in]
        n784 = Append True/False String(1:w1882, 2:"FAIL" ("真字符串"), 3:"PASS" ("真字符串")) -> (0:w1880:string)  [unwired: 1 in]
        n785 = Build Array (concatenate)(w1881, w1871, w1880) -> (w1878:string[])
        n786 = Flatten To XML(anything=w1878) -> (xml string=w1879:string)
        n787 = call "AMC Send Local Message.vi"("Process (\"\" - local)"=w1875, "Message Value"=w1879, "Message Name"=w1875) -> ()  [unwired: 7 in, 2 out]
        n788 = Equal?(x=w1870, y="Error") -> (x = y?=w1867:bool)
        n789 = Equal?(x=w1870, y="Finalization_NG_unit") -> (x = y?=w1883:bool)
        n790 = Or(x=w1883, y=w1867) -> (x .or. y?=w1868:bool)
      }
      frame "BOOST_MODE" {
        w1908 = "UIdisplay" ("Process (\"\" - local)")
        w1906 = "Enable" ("元素")
        n791 = Unbundle By Name(w1895) -> ("Table"=w1907:string[][])
        n792 = call "Select_Table_Vaule.vi"("Vaule"=w1906, "Action"=w1904, "Table"=w1907) -> ("Result"=w1915:bool, "vaule"=w1914:string[])  [unwired: 7 in]
        n793 = call "LogStatus.vi"("error in (no error)"=w1922, "last message"=w1921, "message"=w1904) -> ("error  out"=w1920:errorcluster)  [unwired: 8 in]
        n794 = Append True/False String(1:w1915, 2:"FAIL" ("真字符串"), 3:"PASS" ("真字符串")) -> (0:w1913:string)  [unwired: 1 in]
        n795 = Build Array (concatenate)(w1914, w1906, w1913) -> (w1911:string[])
        n796 = call "3.2.0_BOOST_MODE.vi"("Data in"=w1895, "error in (no error)"=w1920, "AllControls In"=w1897, 10:w1905, "Message Queue out"=w1918) -> ("error out"=w1919:errorcluster, "Flow"=w1893:string, "Data"=w1916:T4, "Message Queue Out"=w1917:T5, "Data out"=w1896:T1)  [unwired: 2 in]
        n797 = Flatten To XML(anything=w1911) -> (xml string=w1912:string)
        n798 = call "AMC Send Local Message.vi"("Process (\"\" - local)"=w1908, "Message Value"=w1912, "Message Name"=w1908) -> ()  [unwired: 7 in, 2 out]
        n799 = Flush Queue(queue=w1917) -> (queue out=w1898:T5)  [unwired: 1 in, 2 out]
        n800 = Equal?(x="Airwatts_Tunings_&_Performance_Test_Max_Power_MODE", y=w1893) -> (x = y?=w1892:bool)
        n801 = Equal?(x=w1893, y="Error") -> (x = y?=w1900:bool)
        n802 = Equal?(x=w1893, y="Finalization_NG_unit") -> (x = y?=w1902:bool)
        n803 = Compound Arithmetic op=OR ("复合运算")(w1892, w1902, w1900) -> (w1899:bool)
      }
      frame "BOOST_Stop_motor" {
        w1923 = "BOOST_Save_Calibration"
        n804 = Unbundle By Name(w1936) -> ("Table"=w1942:string[][], "daemon reference"=w1946:refnum<k5>)
        n805 = call "Select_Table_Vaule Enable_Disable.vi"("Action"=w1943, "Table"=w1942) -> ("Enable"=w1941:bool)  [unwired: 8 in, 1 out]
        n806 = case shown="True" w1941 {
          tunnel: w1946 -> [w1953 w1964]
          tunnel: [w1953 w1963] -> w1934
          tunnel: ["" ("software string") w1956] -> w1938
          tunnel: w1943 -> [_ w1962]
          tunnel: w1942 -> [_ w1961]
          tunnel: [_ w1958] -> w1935
          tunnel: [_ w1956] -> _
          tunnel: [_ w1955] -> _
          tunnel: [_ w1954] -> _
          frame False {
            (unwired) TRUE
          }
          frame True {
            w1954 = "STOP" ("Power Mode")
            w1969 = "UIdisplay" ("Process (\"\" - local)")
            n807 = call "drive_motor.vi"("Power Mode"=w1954, "daemon reference in"=w1964) -> ("error out"=w1957:errorcluster, "response"=w1956:string, "daemon reference out"=w1963:refnum<k5>)  [unwired: 6 in, 1 out]
            n808 = call "Time Delay"("error in (no error)"=w1957) -> ("error out"=w1958:errorcluster)  [unwired: 10 in]
            n809 = call "Select_Table_Vaule.vi"("Vaule"=w1956, "Action"=w1962, "Table"=w1961) -> ("Result"=w1959:bool, "vaule"=w1960:string[])  [unwired: 7 in]
            n810 = Append True/False String(1:w1959, 2:"FAIL" ("真字符串"), 3:"PASS" ("真字符串")) -> (0:w1955:string)  [unwired: 1 in]
            n811 = Build Array (concatenate)(w1960, w1956, w1955) -> (w1968:string[])
            n812 = Flatten To XML(anything=w1968) -> (xml string=w1967:string)
            n813 = call "AMC Send Local Message.vi"("Process (\"\" - local)"=w1969, "Message Value"=w1967, "Message Name"=w1969) -> ()  [unwired: 7 in, 2 out]
          }
        }
        n814 = call <vilib>:"Space Constant.vi"() -> ("String"=w1945:string)
        n815 = Concatenate Strings(w1943, w1945, w1938) -> (w1944:string)
        n816 = Unbundle By Name(w1925) -> ("MES bool"=w1931:refnum<vi>)
        n817 = call "HD_Config.vi"("Step"=enum16{"Initial", "Write", "Read"}."Read") -> ("HD Config out"=w1932:T7)  [unwired: 9 in, 1 out]
        n818 = property class="Bool (严格)"(reference=w1931) -> ("Value"=w1929:bool)  [unwired: 1 in, 2 out]
        n819 = Unbundle By Name(w1932) -> ("Fail_resume_mode"=w1930:bool)
        n820 = Not(x=w1929) -> (.not. x?=w1927:bool)
        n821 = Or(x=w1930, y=w1927) -> (x .or. y?=w1928:bool)
        n822 = Bundle By Name(cluster=w1936, "daemon reference"=w1934) -> (w1933:T1)
        n823 = Select(t="BOOST_Get_AW_Calibration_value", s=w1928, f=w1923) -> ()  [unwired: 1 out]
        n824 = call "LogStatus.vi"("error in (no error)"=w1935, "last message"=w1947, "message"=w1944) -> ("error  out"=w1948:errorcluster)  [unwired: 8 in]
        n825 = case shown="Error" w1935 {
          tunnel: [_ TRUE] -> w1939
          tunnel: [_ "Error"] -> w1940
          frame No Error {
          }
          frame Error {
          }
        }
      }
      frame "BOOST_Save_Calibration" {
        n826 = Unbundle By Name(w1983) -> ("Table"=w1990:string[][], "daemon reference"=w1995:refnum<k5>, "Config"=w1988:string[][])
        n827 = Unbundle By Name(w1971) -> ("MES bool"=w1976:refnum<vi>)
        n828 = call "HD_Config.vi"("Step"=enum16{"Initial", "Write", "Read"}."Read") -> ("HD Config out"=w1977:T7)  [unwired: 9 in, 1 out]
        n829 = property class="Bool (严格)"(reference=w1976) -> ("Value"=w1974:bool)  [unwired: 1 in, 2 out]
        n830 = Unbundle By Name(w1977) -> ("Fail_resume_mode"=w1975:bool)
        n831 = call "Select_Table_Vaule Enable_Disable.vi"("Action"=w1991, "Table"=w1990) -> ("Enable"=w1989:bool)  [unwired: 8 in, 1 out]
        n832 = Not(x=w1974) -> (.not. x?=w1973:bool)
        n833 = Or(x=w1975, y=w1973) -> (x .or. y?=w1970:bool)
        n834 = case shown="False" w1989 {
          tunnel: w1995 -> [w2002 w2012]
          tunnel: [w2002 w2011] -> w1981
          tunnel: [w2001 w2005] -> w1985
          tunnel: w1991 -> [_ w2010]
          tunnel: w1990 -> [_ w2009]
          tunnel: w1988 -> [_ _]
          tunnel: [_ w2006] -> w1982
          tunnel: [w2001 w2005] -> w1979
          tunnel: [w2001 w2004] -> w1978
          tunnel: w1970 -> [_ w2003]
          frame False {
            w2001 = "Skip" ("software string")
            (unwired) TRUE
          }
          frame True {
            w2015 = "UIdisplay" ("Process (\"\" - local)")
            n835 = case shown="False" w2003 {
              tunnel: w2012 -> [w2024 w2026]
              tunnel: [w2023 w2026] -> w2011
              tunnel: [w2022 _] -> w2006
              tunnel: [w2021 "Skip" ("response")] -> w2005
              frame False {
                n836 = call "finalise_calibration.vi"("daemon reference in"=w2024) -> ("error out"=w2022:errorcluster, "response"=w2021:string, "daemon reference out"=w2023:refnum<k5>)  [unwired: 7 in, 1 out]
                n837 = call "时间延迟2"("error in (no error)"=w2022) -> ()  [unwired: 10 in, 1 out]
              }
              frame True {
              }
            }
            n838 = call "Select_Table_Vaule.vi"("Vaule"=w2005, "Action"=w2010, "Table"=w2009) -> ("Result"=w2007:bool, "vaule"=w2008:string[])  [unwired: 7 in]
            n839 = case shown="False" w2003 {
              tunnel: w2007 -> [w2017 _]
              tunnel: [w2016 "Skip" ("response")] -> w2004
              frame False {
                n840 = Append True/False String(1:w2017, 2:"FAIL" ("真字符串"), 3:"PASS" ("真字符串")) -> (0:w2016:string)  [unwired: 1 in]
              }
              frame True {
              }
            }
            n841 = Build Array (concatenate)(w2008, w2005, w2004) -> (w2014:string[])
            n842 = Flatten To XML(anything=w2014) -> (xml string=w2013:string)
            n843 = call "AMC Send Local Message.vi"("Process (\"\" - local)"=w2015, "Message Value"=w2013, "Message Name"=w2015) -> ()  [unwired: 7 in, 2 out]
          }
        }
        n844 = call <vilib>:"Space Constant.vi"() -> ("String"=w1994:string)
        n845 = Concatenate Strings(w1991, w1994, w1985) -> (w1993:string)
        n846 = Bundle By Name(cluster=w1983, "daemon reference"=w1981, "BOOST.Finalise Calibration"=w1979, "BOOST_Status.Finalise Calibration"=w1978) -> (w1980:T1)
        n847 = call "LogStatus.vi"("error in (no error)"=w1982, "last message"=w1996, "message"=w1993) -> ("error  out"=w1997:errorcluster)  [unwired: 8 in]
        n848 = case shown="Error" w1982 {
          tunnel: [_ TRUE] -> w1986
          tunnel: [_ "Error"] -> w1987
          frame No Error {
          }
          frame Error {
          }
        }
      }
      frame "BOOST_Get_AW_Calibration_value" {
        n849 = Unbundle By Name(w2047) -> ("Table"=w2051:string[][], "daemon reference"=w2050:refnum<k5>)
        n850 = Unbundle By Name(w2049) -> ("ECO.Delta_P"=w2056:dbl, "BOOST.Delta_P"=w2055:dbl)
        n851 = Build Array(w2056, w2055) -> (w2054:dbl[])
        n852 = call "Select_Table_Vaule Enable_Disable.vi"("Action"=w2058, "Table"=w2051) -> ("Enable"=w2057:bool)  [unwired: 8 in, 1 out]
        n853 = case shown="True" w2057 {
          tunnel: w2050 -> [w2072 w2096]
          tunnel: [w2072 w2095] -> w2044
          tunnel: [w2071 w2086] -> w2048
          tunnel: w2058 -> [_ w2098]
          tunnel: w2051 -> [_ w2097]
          tunnel: [_ w2084] -> w2034
          tunnel: w2054 -> [_ w2078]
          tunnel: [_ w2083] -> w2046
          tunnel: [w2070 w2076] -> w2045
          tunnel: [w2070 w2073] -> w2029
          frame False {
            w2071 = "Skip" ("software string")
            (unwired) TRUE
            n854 = Initialize Array(w2071, 2 ("维数大小")) -> (w2070:string[])
          }
          frame True {
            w2094 = "UIdisplay" ("Process (\"\" - local)")
            n855 = Number To Fractional String(number=w2078) -> (F-format string=w2080:string[])  [unwired: 3 in]
            n856 = for {
              shift-right: [w2109] -> w2095
              shift-left: w2096 -> [w2119]
              tunnel: u32[] [0, 1] -> [w2118] mode=indexing
              tunnel: [w2117] -> w2077 mode=indexing
              shift-right: [w2116] -> w2086
              shift-left: "" -> [w2115]
              tunnel: [w2111] -> w2083
              tunnel: [w2110] -> w2081 mode=indexing
              n857 = call "get_aw_tune.vi"("Index"=w2118, "daemon reference in"=w2119) -> ("error out"=w2111:errorcluster, "AW Tune Parameter"=w2110:T3, "response"=w2114:string, "daemon reference out"=w2109:refnum<k5>)  [unwired: 5 in, 1 out]
              n858 = Unbundle By Name(w2110) -> ("Offset power mW"=w2117:i64)
              n859 = Concatenate Strings(w2114, ";" ("字符串")) -> (w2112:string)
              n860 = Concatenate Strings(w2115, w2112) -> (w2116:string)
            }
            "Array" <- w2081
            n861 = for {
              tunnel: w2080 -> [w2105] mode=indexing
              tunnel: "NaN" -> [w2108]
              tunnel: [w2106] -> w2082 mode=indexing
              tunnel: w2078 -> [w2103] mode=indexing
              n862 = Equal?(x=w2105, y=w2108) -> (x = y?=w2107:bool)
              n863 = Select(t=0.0, s=w2107, f=w2103) -> (s? t:f=w2106:dbl)
            }
            n864 = To Long Integer(number=w2082) -> (32bit integer=w2075:i32[])
            n865 = call "Select_Table_Vaule.vi"("Vaule"=w2086, "Action"=w2098, "Table"=w2097) -> ("vaule"=w2088:string[])  [unwired: 7 in, 1 out]
            n866 = Equal?(x=w2077, y=w2075) -> (x = y?=w2074:bool[])
            n867 = And Array Elements(Boolean array=w2074) -> (logical AND=w2084:bool)
            n868 = for {
              tunnel: w2074 -> [w2100] mode=indexing
              tunnel: [w2099] -> w2073 mode=indexing
              n869 = Append True/False String(1:w2100, 2:"FAIL" ("真字符串"), 3:"PASS" ("真字符串")) -> (0:w2099:string)  [unwired: 1 in]
            }
            n870 = Append True/False String(1:w2084, 2:"FAIL" ("真字符串"), 3:"PASS" ("真字符串")) -> (0:w2089:string)  [unwired: 1 in]
            n871 = Build Array (concatenate)(w2088, w2086, w2089) -> (w2093:string[])
            n872 = Number To Fractional String(number=w2077) -> (F-format string=w2076:string[])  [unwired: 3 in]
            n873 = Flatten To XML(anything=w2093) -> (xml string=w2092:string)
            n874 = call "AMC Send Local Message.vi"("Process (\"\" - local)"=w2094, "Message Value"=w2092, "Message Name"=w2094) -> ()  [unwired: 7 in, 2 out]
          }
        }
        n875 = Unbundle By Name(w2036) -> ("MES bool"=w2041:refnum<vi>)
        n876 = call "HD_Config.vi"("Step"=enum16{"Initial", "Write", "Read"}."Read") -> ("HD Config out"=w2042:T7)  [unwired: 9 in, 1 out]
        n877 = Unbundle By Name(w2042) -> ("Fail_resume_mode"=w2040:bool)
        n878 = property class="Bool (严格)"(reference=w2041) -> ("Value"=w2039:bool)  [unwired: 1 in, 2 out]
        n879 = Not(x=w2039) -> (.not. x?=w2038:bool)
        n880 = call <vilib>:"Space Constant.vi"() -> ("String"=w2060:string)
        n881 = Or(x=w2040, y=w2038) -> (x .or. y?=w2035:bool)
        n882 = Concatenate Strings(w2058, w2060, w2048) -> (w2059:string)
        n883 = Select(t=TRUE, s=w2035, f=w2034) -> (s? t:f=w2033:bool)
        n884 = case shown="No Error" w2046 {
          tunnel: w2033 -> [w2065 _]
          tunnel: [w2064 "Error"] -> w2052
          frame No Error {
            n885 = Select(t="Airwatts_Tunings_&_Performance_Test_Max_Power_MODE", s=w2065, f="Finalization_NG_unit") -> (s? t:f=w2064:string)
          }
          frame Error {
          }
        }
        n886 = Index Array(array=w2045) -> (element #1=w2031:string, element #2=w2030:string)  [unwired: 2 in]
        n887 = Index Array(array=w2029) -> (element #1=w2028:string, element #2=w2027:string)  [unwired: 2 in]
        n888 = Bundle By Name(cluster=w2047, "daemon reference"=w2044, "BOOST.ECO - Get AW Calibration value"=w2031, "BOOST.BOOST - Get AW Calibration value"=w2030, "BOOST_Status.ECO - Get AW Calibration value"=w2028, "BOOST_Status.BOOST - Get AW Calibration value"=w2027) -> (w2043:T1)
        n889 = call "LogStatus.vi"("error in (no error)"=w2046, "last message"=w2061, "message"=w2059) -> ("error  out"=w2062:errorcluster)  [unwired: 8 in]
      }
    }
    n890 = call "6-AlarmStatus.vi"("Step"=enum16{"Initial", "Write", "Read"}."Read") -> ("AlarmValue Out"=w20:bool[])  [unwired: 9 in, 1 out]
    n891 = call "Stop.vi"("Step"=enum16{"Initial", "Write", "Read"}."Read") -> ("Stop Out"=w28:bool)  [unwired: 9 in, 1 out]
    n892 = call "Exit.vi"("Step"=enum16{"Initial", "Write", "Read"}."Read" ("step")) -> ("Exit Out"=w27:bool)  [unwired: 9 in, 1 out]
    n893 = Or Array Elements(Boolean array=w20) -> (logical OR=w19:bool)
    n894 = Compound Arithmetic op=OR(w26, w28, w27, w19) -> (w25:bool)
    n895 = call "AMC Run Step.vi"("Message Queue In"=w46, "Message Name"=w34, "Message Value"=w32, "error in (no error)"=w41, "Mli/Sig"=FALSE) -> ("Message Queue Out"=w45:T5, "error out"=w40:errorcluster)  [unwired: 13 in]
  }
  "Message Queue Out" <- w8
  "error out" <- w7
  "Data" <- w12
  "Flow" <- w10
  "Data out" <- w5
